vi "BIMS for Export Control.vi"() -> ()   [LabVIEW 2015]
doc: "This program is currently beta software. It is designed to address the data requirements defined primarily by the DHB Ballistic Test Report.\n\nThe general operation of this program is based on the Ballistics Version 2005 application developed internally by DuPont as a research tool for the Spruance Plant Ballistics Lab in Richmond, VA.\n\nPlease note that the original trigger control logic was modified and no longer depends on a safety interlock system to enable operation of a ballistic test.\n\nDuPont makes no warranties and assumes no liabilities in connection with any use of this program."
uses:
  <vilib>/addons/database/NI_Database_API.lvlib
  <vilib>/addons/database/Connection.llb/Conn Execute.vi
  <vilib>/addons/database/Recordset.llb/Rec Destroy - Connection.vi
  <vilib>/Utility/config.llb/NI_LVConfig.lvlib
  <vilib>/Utility/config.llb/Write Key (I32).vi
  Shot Record.ctl
  BIMS_Collector Globals.vi
  Collector State.ctl
  DataSource.ctl
  <vilib>/registry/registry.llb/Registry RtKey.ctl
  <vilib>/Utility/config.llb/Write Key (String).vi
  <vilib>/addons/database/Connection.llb/DB Tools Open Connec (Path).vi
panel:
  out "Loading":u16(ring)
  in  "runtimeMenusVisible":bool=TRUE
  in  "diagPageVisible":bool
  in  "RESET All":bool
  out "ConfigName":string
  out "TimeNow":string
  in  "EXIT":bool
  in  "mainTabCntrl":enum32{"Setup", "Measure", "History", "System"}(tab)=enum."System"
  in  "SampleEntryTabCntrl":enum32{"Environment", "Sample"}(tab)
  in  "ThreatDetails":u16(ring) caption="Detail" items=["2gr 223 cal.   FSP", "4gr 223 cal.   FSP", "16gr 223 cal.", "64gr .357 cal."]
  in  "ThreatGroups":u16(ring) caption="Group" items=["", "RCC", "FSP", "44 Magnum", "40 S&W", "9mm Luger", "357 Magnum", "357 Sig", "5.56 NATO / 223", "7.62 Win"]
  in  "PowderTypes":u16(ring) caption="Type" items=["", "ACCURATE, NO.2", "ACCURATE, NO.9", "Alliant Herc. Bullseye", "Alliant 2400", "Hercules", "Hi-Skor 700x", "Hi-Skor 800x", "IMR-4198", "IMR-4756", "IMR-4895", "Power Pistol", "Winchester Ball", "WINCHESTER-231", "WINCHESTER-296", "OTHER"]
  in  "Ballisticians":u16(ring) caption="Ballistician" items=["", "Luke Jeter", "Pat Fitzgerald", "James Singletary", "Aldo Tavarez"]
  in  "Recorders":u16(ring) caption="Recorder"
  in  "Shooters":u16(ring) caption="Shooter"
  in  "Methods":u16(ring) caption="Method" items=["", "V50", "NIJ", "V0", "Custom"]
  in  "RoomT":sgl caption="Temperature (° F)" format="%.1f"
  in  "RoomHum":sgl caption="Humidity (%)" min=0 max=100 format="%.1f"
  in  "SampleBackings":u16(ring)=3 caption="Type" items=["", "Clay", "Aluminum", "Air"]
  in  "clayCalArray":i16[](array[numeric])=[0, 0, 0, 0, 0] caption="Calibration (mm)" min=0 max=99 format="%02.0f"
  out "clayAverage":sgl caption="Clay Average (mm)" format="%#.1f"
  in  "clayTemp":sgl caption="Clay Temp (° F)" format="%.1f"
  out "threatDetails":T1 caption="Description"
  in  "SampleClamping":u16(ring) caption="Clamping" items=["", "None", "12 x 12", "12 x 15", "15 x 15 Flat", "15 x 15 Teeth", "16 x 16 Flat", "16 x 16 Teeth", "18 x 18", "20 x 20", "Hydro Pneumatic"]
  in  "Sample SubTabCntrl":T2(tab)
  in  "SampleID":string caption="Sample ID"
  in  "SampleDimensions":u16(ring) caption="Dimensions" items=["", "15 x 15", "12 x 12", "10.25 x 11.75", "15 x 16", "26 x 26", "8.5 x 11", "12 x 15", "16 x 16", "18 x 18", "20 x 16", "15 x 18", "24 x 24", "13 x 13", "7.5 x 7.5", "VEST PANEL", "CHEST PLATE", "HELMET", "NOT APPLICABLE"]
  in  "ModelMfrs":u16(ring) caption="Manufacturer" items=["DuPont Experimental", "Clark Schwebel", "Industriales Textiles", "Maydown", "Second Chance Body Armor", "Point Blank-Marine Interceptor", "Safari Land", "American Body Armor", "Europe", "Force One", "Textile Filter", "Hexcel Schwebel", "BGF", "M.C. GILL", "COLUMBIA", "Britax HEATH TECN", "ARLON", "TEX TECH INC.", "TELAIR", "CADDIN BODY ARMOR", "GEPCO", "3 TEX", "PACA BODY ARMOR", "VON ROL ISOLA", "SIOUX MANUFACTURING", "APEJ-TAIWAN", "FLOPPY BODY ARMOR", "UNICOR", "n/a", "Point Blank", "Diamond Back", "Other"]
  in  "SampleTypes":u16(ring) caption="Sample Type" items=["", "Fabric", "Hard", "Helmet", "Vest", "Paper"]
  in  "Submitters":u16(ring) caption="Submitter" items=["", "Aldo Tavarez", "James Singletary", "Jeff Hanks", "Karl Chang", "Minshon Chiou", "Other", "Navin Tejani", "Pat Fitzgerald", "Ron Egres", "Bryce VanArsdalen", "Kevin Mulcahy"]
  in  "ProjectID":string caption="Project ID"
  in  "BackLayers":i32 caption="# of Layers" min=0 max=99 step=5
  in  "FrontLayers":i32 caption="# of Layers" min=0 max=99 step=5
  in  "BackLayer":u16(ring) caption="Back Layer" items=["", "n/a", "CORDURA 500d"]
  in  "FrontLayer":u16(ring) caption="Front Layer" items=["", "n/a", "CORDURA 1000d"]
  out "totalNumLayers":i32 caption="Total # of Layers" min=0 max=100 step=5
  out "totalBAW":sgl caption="Total BAW (psf)" format="%.2f"
  in  "LayerTabControl":enum32{"1", "2", "3", "4", "5", "6"}(tab) caption="Inner Layers"
  out "fab1_totalWt":sgl caption="Fab1 Wt" min=0 max=99 step=5 format="%.2f"
  out "SampleAttribs_1":T3 caption="fabricAttribs_1"
  in  "Layer_1":T4={"plyNum"=0, "LotNum"="n/a", "RollNum"="n/a"} caption="Fabric #1" {"plyNum" min=0 max=99 step=5}
  in  "SampleStyle_1":u16(ring) items=["", "215490", "215590", "217583", "2182", "2710", "2722", "2754", "275580", "400063", "440094", "440094ML", "FC-TWE-1096-160.0-1072"]
  in  "Mfr_1":u16(ring) caption="vendor" items=["", "Barrday", "DSM", "DuPont AFS", "Dyneema", "Honeywell", "JPS", "TexTech"]
  in  "layerStitch_1":u16(ring) caption="Stitch" items=["", "1-inch quilt", "2-inch quilt", "Corner Bartack", "Corners", "Custom (Panel)", "Custom (Vest)", "Diamond", "Edge", "n/a", "Normal"]
  out "fab2_totalWt":sgl caption="Fab2 Wt" min=0 max=99 step=5 format="%.2f"
  out "SampleAttribs_2":T3 caption="fabricAttribs_2"
  in  "Layer_2":T4={"plyNum"=0, "LotNum"="n/a", "RollNum"="n/a"} caption="Fabric #2" {"plyNum" min=0 max=99 step=5}
  in  "SampleStyle_2":u16(ring)
  in  "Mfr_2":u16(ring) caption="vendor" items=["", "Barrday", "DSM", "DuPont AFS", "Dyneema", "Honeywell", "JPS", "TexTech"]
  in  "layerStitch_2":u16(ring) caption="Stitch" items=["", "1-inch quilt", "2-inch quilt", "Corner Bartack", "Corners", "Custom (Panel)", "Custom (Vest)", "Diamond", "Edge", "n/a", "Normal"]
  out "fab3_totalWt":sgl caption="Fab3 Wt" min=0 max=99 step=5 format="%.2f"
  out "SampleAttribs_3":T3 caption="fabricAttribs_3"
  in  "Layer_3":T4={"plyNum"=0, "LotNum"="n/a", "RollNum"="n/a"} caption="Fabric #3" {"plyNum" min=0 max=99 step=5}
  in  "SampleStyle_3":u16(ring)
  in  "Mfr_3":u16(ring) caption="vendor" items=["", "Barrday", "DSM", "DuPont AFS", "Dyneema", "Honeywell", "JPS", "TexTech"]
  in  "layerStitch_3":u16(ring) caption="Stitch" items=["", "1-inch quilt", "2-inch quilt", "Corner Bartack", "Corners", "Custom (Panel)", "Custom (Vest)", "Diamond", "Edge", "n/a", "Normal"]
  out "fab4_totalWt":sgl caption="Fab4 Wt" min=0 max=99 step=5 format="%.2f"
  out "SampleAttribs_4":T3 caption="fabricAttribs_4"
  in  "Layer_4":T4={"plyNum"=0, "LotNum"="n/a", "RollNum"="n/a"} caption="Fabric #4" {"plyNum" min=0 max=99 step=5}
  in  "SampleStyle_4":u16(ring)
  in  "Mfr_4":u16(ring) caption="vendor" items=["", "Barrday", "DSM", "DuPont AFS", "Dyneema", "Honeywell", "JPS", "TexTech"]
  in  "layerStitch_4":u16(ring) caption="Stitch" items=["", "1-inch quilt", "2-inch quilt", "Corner Bartack", "Corners", "Custom (Panel)", "Custom (Vest)", "Diamond", "Edge", "n/a", "Normal"]
  out "fab5_totalWt":sgl caption="Fab5 Wt" min=0 max=99 step=5 format="%.2f"
  out "SampleAttribs_5":T3 caption="fabricAttribs_5"
  in  "Layer_5":T4={"plyNum"=0, "LotNum"="n/a", "RollNum"="n/a"} caption="Fabric #5" {"plyNum" min=0 max=99 step=5}
  in  "SampleStyle_5":u16(ring)
  in  "Mfr_5":u16(ring) caption="vendor" items=["", "Barrday", "DSM", "DuPont AFS", "Dyneema", "Honeywell", "JPS", "TexTech"]
  in  "layerStitch_5":u16(ring) caption="Stitch" items=["", "1-inch quilt", "2-inch quilt", "Corner Bartack", "Corners", "Custom (Panel)", "Custom (Vest)", "Diamond", "Edge", "n/a", "Normal"]
  out "fab6_totalWt":sgl caption="Fab6 Wt" min=0 max=99 step=5 format="%.2f"
  out "SampleAttribs_6":T3 caption="fabricAttribs_6"
  in  "Layer_6":T4={"plyNum"=0, "LotNum"="n/a", "RollNum"="n/a"} caption="Fabric #6" {"plyNum" min=0 max=99 step=5}
  in  "SampleStyle_6":u16(ring)
  in  "Mfr_6":u16(ring) caption="vendor" items=["", "Barrday", "DSM", "DuPont AFS", "Dyneema", "Honeywell", "JPS", "TexTech"]
  in  "layerStitch_6":u16(ring) caption="Stitch" items=["", "1-inch quilt", "2-inch quilt", "Corner Bartack", "Corners", "Custom (Panel)", "Custom (Vest)", "Diamond", "Edge", "n/a", "Normal"]
  in  "SampleCoverings":u16(ring) caption="Sample Covering" items=["None", "RipStop", "Plastic bag", "Other"]
  in  "Assemblers":u16(ring) caption="Technician" items=["", "Not Known", "none", "Ron Egres", "Bryce VanArsdalen", "Mary Revels", "Matthew Street", "Patty Whitlow", "Tom Boyer"]
  in  "Thickness":dbl caption="Thickness (in)" format="%.3f"
  in  "totalSampleWt":sgl caption="Total Weight (lbs)" format="%.3f"
  in  "Comments":string caption="Remarks (optional):"
  in  "TestConditions":u16(ring) caption="Sample Condition" items=["", "Dry", "Wet", "Hot 160 DEG. F", "Cold", "Weapon Lubricant", "Motor Oil", "Conditioned", "Accelerated Aging"]
  in  "shotsTabCntrl":T5(tab)
  in  "Frag Rod":sgl format="%.1f"
  in  "MeasSrc":T6=enum."Screens" caption="Source"
  in  "Drag Corrected":bool=TRUE
  in  "ARM":bool
  in  "readyClock":bool caption="Clock"
  out "Impact/speed":sgl caption="Chronograph 1" min=0 max=10000 step=0.1 format="%.1f"
  out "SHOT STATUS":u16(ring) caption="Penetration" items=["Partial", "Complete"]
  out "residual/speed":sgl caption="Residual" min=0 max=10000 step=0.1 format="%.1f"
  out "SUBMIT DATE/TIME":string
  out "BACKFACE DEPTH":sgl caption="Backface\nDepth" min=0 max=200 step=5
  in  "MeasVelScrnSet1":sgl caption="Set #1" min=0 max=10000 step=0.1 format="%.1f"
  in  "Current/sthotstatus":u16(ring) caption="Penetration" items=["Partial", "Complete"]
  in  "Current/residual/speed":sgl caption="Residual Set" min=0 max=10000 step=0.1 format="%.1f"
  in  "currentDateTime":string caption="Date/Time"
  in  "MeasVelScrnSet2":sgl caption="Set #2" min=0 max=1000000 step=0.1 format="%.1f"
  out "%_Difference":sgl caption="% Vel Diff" format="%.3f"
  in  "backdepth":sgl caption="BF Depth"
  out "Redundant/speed":sgl caption="Chronograph 2" min=0 max=10000 step=0.1 format="%.1f"
  out "Current/avg/speed":sgl caption="Average" min=0 max=1000000 step=0.1 format="%.1f"
  out "Avg/speed":sgl caption="Average" min=0 max=10000 step=0.1 format="%.1f"
  out "SafetyInterlock":cluster{"ARMED":bool}
  out "DC_ factor":sgl=1.0 caption="DC Factor" format="%.4f"
  in  "Barrel Temp":sgl format="%.1f"
  in  "Shot Description":string caption="Description (optional)"
  in  "Powder Loading":sgl caption="Powder Load" min=0 max=100 step=0.1 format="%.3f"
  in  "Shot Angle":u16 max=90 step=1
  out "Projectile Mass":sgl caption="Projectile Mass (grains)" min=0 step=1
  in  "N.I.J":u16(ring) items=["n/a", "PASS", "FAIL"]
  out "Device S/N":string
  in  "addShot":bool caption="RANGE SETUP must be selected before shots can be added."
  in  "loadingUnits":enum32{"grams", "grains"}(radio)
  out "instruct_addShot":string="RANGE SETUP and THREAT must be selected before shots can be added."
  out "Set#1 Separation":sgl=4.0 caption="Outer" format="%.2f"
  out "Set#2 Separation":sgl=4.0 caption="Inner" format="%.2f"
  out "saveReq":string="Number of layers in sample ply specification and number of shots in shots table must be greater than 0 to enable saving."
  in  "VsVr Report":bool caption="Report"
  out "Table of Shots":string[][](table) caption="Shot Table"
  in  "MC Listbox of Shots":i32(listbox)
  in  "saveShots":bool
  in  "clearShots":bool
  out "highPartial":i32 caption="High Partial" min=0 max=10000 step=1
  out "lowComplete":i32 caption="Low Complete" min=0 max=10000 step=1
  out "rangeOfResults":i32 caption="Range of Results" min=0 max=10000 step=1
  out "zmr 2":sgl caption="Low C minus High P" format="%.1f"
  out "computed_V50":sgl caption="V50" format="%.1f"
  out "Pairs":i16 min=0 max=100 step=1
  in  "reportV50":bool caption="Report"
  in  "maxDev":sgl=125.0 caption="Max Deviation" min=0 max=300 step=25
  in  "undoLastShot":bool
  in  "deleteShot":bool
  in  "nextShot":bool
  in  "SHOTS":T7[](array[typedef]) {"Frag Rod" format="%.1f"; "UncorrectedAvgVel_PB" format="%.1f"; "UncorrectedRed_PB" format="%.1f"; "strikeVel_PB" format="%.1f"; "velLoss_PB" format="%.1f"; "avgVel_PB" format="%.1f"; "Redundant_Velocity" format="%.1f"; "Energy Loss (J)" format="%.3e"; "Projectile Mass" min=0 step=1 format="%.4f"; "Corrected residual" format="%.2f"; "Uncorrected Residual" format="%.1f"; "Corrected Impact" format="%.2f"; "Uncorrected Impact" format="%.1f"; "Shot Angle" max=90 step=1; "SHOT STATUS" items=["Partial", "Complete"]; "IMPACT VELOCITY" min=0 max=10000 step=0.1 format="%.1f"; "Barrel Temperature" format="%.1f"; "Powder Loading" format="%.4f"; "RESIDUAL  VELOCITY" min=0 max=10000 step=0.1 format="%.1f"}
  out "velProfile":cluster{dbl, dbl}[](graph) caption="Shot Velocity Measurement Profile"
  out "velCompProf":cluster{"vStrike":dbl, "vA":dbl} caption="Velocity in fps\n(computed)"
  out "velMeasProf":T8 caption="Velocity in fps\n(measured)"
  out "relativeTime":cluster{"ts2":dbl, "ts3":dbl, "ts1":dbl} caption="Relative time\n(microsec)"
  out "displacement":T9={"ds_v2"=6.75, "ds2"=5.0833, "ds_vB"=4.9167, "ds3"=4.75, "ds_vAvg"=6.9167, "ds_v1"=7.0833, "ds1"=8.75, "ds_vA"=8.9167, "ds0"=9.0833} caption="Distance from\ntarget (ft)" {"ds0" format="%_4g"; "ds_vA" format="%_4g"; "ds1" format="%_4g"; "ds_v1" format="%_4g"; "ds_vAvg" format="%_4g"; "ds3" format="%_4g"; "ds_vB" format="%#_4g"; "ds2" format="%#_4g"; "ds_v2" format="%_4g"}
  out "arrIDC":dbl[](array[numeric]) caption="Instantaneous Drag Coefficient"
  in  "rangeSetup":u16(ring)=1 caption="Range Dimensions" items=["Short (small frag)", "Standard (handgun)", "Long (rifle)"]
  out "mid_to_targ_dist":sgl=5.0 caption="Mid To Target (ft)"
  in  "historyTabCntrl":enum32{"Powder Loading", "Panel Search"}(tab)=enum."Panel Search"
  in  "Threat.freeTxt":string caption="Threat"
  in  "Powder.freeTxt":string caption="Powder"
  in  "QueryLoad":bool
  in  "lkupEndDate":timestamp caption="End Date" format="%<%x>T"
  in  "lkupStartDate":timestamp caption="Begin Date" format="%<%x>T"
  out "Vel.vs.Loading":cluster{dbl[], dbl[]}(graph)
  out "v50_table":string[][](table)
  in  "maxRecs":u16=1001 caption="Max # of SHOT Records" min=1 max=10000 step=100
  out "ActualNumRecs":i32=1001 caption="Actual # Returned"
  in  "ThreatSize_0":u16(ring) caption="Threat Size" items=["", "2", "4", "16", "17", "44", "55", "62", "64", "85", "123", "124", "125", "148", "158", "166", "180", "207", "240"]
  in  "panelSearch":bool
  in  "Mfr_0":u16(ring) caption="Manufacturer" items=["", "Barrday", "DSM", "DuPont AFS", "Dyneema", "Honeywell", "JPS", "TexTech"]
  in  "SampleStyle_0":u16(ring) caption="Sample Style"
  in  "srchParams":T10={"maxPanels"=1001, "lkupPanelStartDate"=timestamp(0 s since 1904-01-01), "lkupPanelEndDate"=timestamp(3345122114.0909824 s since 1904-01-01)} {"lkupPanelEndDate" format="%<%x>T"; "lkupPanelStartDate" format="%<%x>T"; "maxPanels" min=1 max=10000 step=100}
  out "actualNumPanels":i32 caption="Actual # Returned"
  out "pastPanels":string[][](table)
  in  "Record #":i32=1 min=0 max=16
  in  "reportV50_History":bool
  out "SampleAttribs_0":T11 caption="fabricAttribs_1"
  in  "Requestors_0":u16(ring) caption="Requestor" items=["", "Aldo Tavarez", "Bryce VanArsdalen", "James Singletary", "Jeff Hanks", "Karl Chang", "Kevin Mulcahy", "Minshon Chiou", "Navin Tejani", "Other", "Pat Fitzgerald", "Ron Egres"]
  in  "aboutTabCntrl":T12(tab)
  in  "RefreshMetadata":bool
  out "LastShot":i32 caption="Shot"
  out "LastSample":i32 caption="Sample"
  in  "PublishNewRecords":bool
  in  "Folder":string="esvrs11" caption="Publish Folder"
  in  "clearErrors":bool
  in  "useBMC":bool caption="Use Message Center?"
  in  "Server":string="esvrs11"
  in  "Site":string="ICE1"
  in  "TestStandards":u16(ring)=2 caption="Standard" items=["n/a", "NIJ 0101.04", "MIL-STD-662F"]
  in  "WeaponTypes":u16(ring) caption="Weapon" items=["", "Universal Receiver", "Other"]
  in  "processShots":bool
  out "DIO":u32=21 format="%.0b"
  in  "line direction map":i32=1792 format="%.0b"
  out "Corrected Average":sgl=1527.9313 format="%.2f"
  out "CorrectedVelScrnSet2":sgl=1551.8816 caption="Corrected Redundant" format="%.2f"
  out "conversion factor":sgl=0.3048037 format="%.5f"
  out "#_completes":i32
  out "#_partials":i32
  in  "percent warning":sgl=1.0 format="%.2f"
  in  "SoftwareVersion":dbl caption="Version" format="%.2f"
  out "impact/ID":u32=83886081 format="%.0x"
  out "residual/ID":u32=83951617 format="%.0x"
  out "Red/ID":u32=84017153 format="%.0x"
  out "correction coefficient":sgl format="%.8f"
  out "Corrected Residual":sgl=751.9905 format="%.2f"
  out "CorrectedVelScrnSet1":sgl=1503.981 format="%.2f"
  out "Barrel to Screen":sgl=7.8333 format="%.2f"
  in  "Set#1_to_Target":sgl=7.083333 format="%.2f"
  out "Residual/Separation":sgl=4.0 format="%.2f"
  in  "Residual/Target Dist":sgl=7.083333 format="%.2f"
  out "Z.M.R.":sgl min=0 step=0.1 format="%.1f"
  in  "old threat":u16
  out "Complete":sgl[](array[numeric]) format="%.2f"
  out "factor array":sgl[](array[numeric]) format="%.4f"
  out "Partial":sgl[](array[numeric]) format="%.2f"
  in  "DAQ Card":i16=1
  in  "Impact Timer":i16 min=0 max=3 step=1
  in  "Redundant Timer":i16=1 min=0 max=3 step=1
  in  "Residual  Timer":i16=2 min=0 max=3 step=1
  out "Impact factor":sgl=1.0 caption="Impact" min=0 max=1 format="%.5f"
  out "Residual factor":sgl=1.0 caption="Residual" min=0 max=1 format="%.5f"
  in  "Areal Density":dbl format="%.2f"
  in  "Areal density text":string
  in  "Fabric Description":string caption="Fabric Desc"
  in  "clayCalib":string="##-##-##-##-##" caption="Calibration"
  in  "lookupRec":bool caption="lookup"
  out "STOP (Shots MC LB)":bool=TRUE
  out "configPath":path=path "P:/Private/My Projects/AFS/BIMS/2008/BIMS_Collector.ini" caption="Configuration Path (INI)"
  in  "minV50":i32=1500 caption="Minimum V50"
  in  "Type of work":string="QC"
  in  "Threat":u16(ring) caption="Threat (long description)"
  out "massUnits":string="GRAMS" caption="Weight Units"
  out "lengthUnits":string="FOOT" caption="Distance Units"
  in  "SampleDescrip":u16(ring) caption="Misc. Sample Description (legacy)"
  in  "serialNum":string caption="Serial #"
  in  "Models":u16(ring) caption="Model #" items=["n/a"]
  in  "InterlockExists":bool=TRUE caption="Safety Interlock Hardware Exist?"
  in  "ScreenSetAvgg":bool caption="Average Screen Sets?"
  in  "Sort by AVG":bool=TRUE caption="Sort shots by average velocity"
  in  "useBallisitican":bool=TRUE caption="Use Ballistician field in Setup?"
  in  "useRecorder":bool caption="Use Recorder field in Setup?"
  in  "useShooter":bool caption="Use Shooter field in Setup?"
  out "SMErr":errorcluster
  out "U/I EvErr":errorcluster
  out "booleanDump":bool
  out "GrainSize":u16 caption="Grain"
  in  "LayerStitchTypes":u16(ring) caption="Stitch" items=["", "Custom (Vest)", "Corners", "1-inch quilt", "2-inch quilt", "Normal", "Custom (Panel)", "Corner Bartack", "Diamond", "Edge", "n/a"]
  # "Effectively restarts the application from scratch, as if the user pressed the EXIT button and then restarted the application."
  # "Configured for"
  # "Threat"
  # "*"
  # "*"
  # "Test"
  # "Powder"
  # "*"
  # "Personnel"
  # "Room"
  # "*"
  # "Backing"
  # "*"
  # "*"
  # "*"
  # "Body Side"
  # "Strike Face"
  # "Layer"
  # "Mfr"
  # "Style"
  # "# of Plies"
  # "Lot"
  # "Roll"
  # "Stitch"
  # "Internal ID"
  # "Fiber"
  # "Denier"
  # "Construction"
  # "Weave"
  # "Finish"
  # "Basis weight (oz/yd²)"
  # "Yarn Merge"
  # "Total Weight"
  # "*"
  # "*"
  # "*"
  # "1"
  # "2"
  # "3"
  # "4"
  # "5"
  # "6"
  # "Required"
  # "*"
  # "Timing System"
  # "Shot Parameters"
  # "cm"
  # "deg"
  # "degF"
  # "Velocity Measurements"
  # "Observations"
  # "Screens\nSeparation"
  # "Ft"
  # "Table Functions"
  # "Summary"
  # "Reports"
  # "Test Record"
  # "Edit Shot Records"
  # "Corrected"
  # "Shot #"
  # "t0"
  # "0"
  # "S Strike"
  # "0"
  # "Internal ID#"
  # "Fiber"
  # "Denier"
  # "Pick"
  # "Weave"
  # "Finish"
  # "oz/yd²"
  # "Asset"
  # "DuPont Ballistics Information Management System\n\nBIMS\nFor Export Control\n\n\nBallistic Performance\nData Collector\n\nJune 2010"
  # "DuET Measurement System Technologies\nDUCOM 8 695-2330 for technical support\n\nCopyright © 2010 DuPont Company"
  # "Last Assigned\nRecord Numbers"
  # "Deployment Configuration"
  # "Data items support Point Blank requirements:"
  # "Correction Factors"
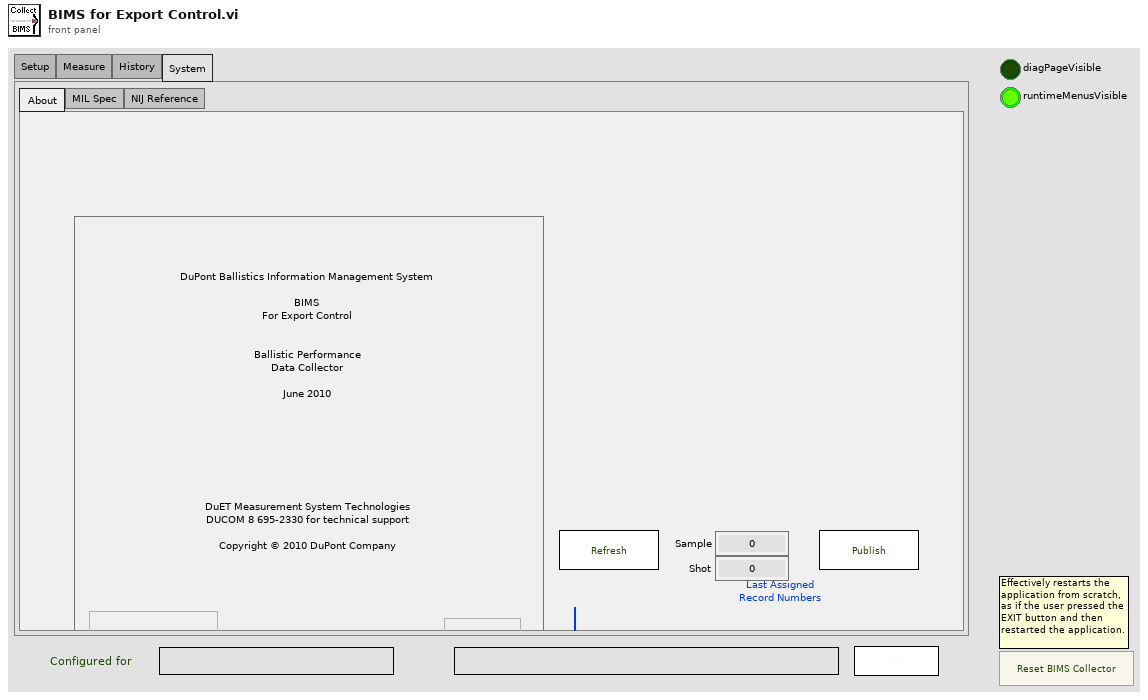
[diagram p1: front panel]
types:
  T1 = cluster{"barrelLength":string, "dragCorrection":string, "detailDescription":string, "barrelCaliber":string, "grainSize":string, "Make":string, "Model":string}
  T2 = enum32{"General Specification", "Ply Specification", "Preparation"}
  T3 = cluster{"Fabric.fiber":string, "Fabric.denier":string, "pick":string, "weave":string, "finish":string, "ozPerYd2":string, "fabricID_DHB":string, "yarnMerge":string}
  T4 = cluster{"plyNum":i32, "LotNum":string, "RollNum":string}
  T5 = enum32{"Ready-Aim-Fire", "Shots Table", "Edit", "Instantaneous DC"}
  T6 = typedef "DataSource.ctl" = enum16{"Simulated", "Radar", "Screens"}
  T7 = typedef "Shot Record.ctl" = cluster{"Uncorrected Impact":sgl, "Uncorrected Residual":sgl, "avgVel_PB":sgl, "IMPACT VELOCITY":sgl, "RESIDUAL  VELOCITY ":sgl, "Shot Description":string, "Powder Loading ":sgl, "Barrel Temperature":sgl, "TIME / DATE":string, "shot order":i32, "SHOT STATUS":u16, "Shot Angle":u16, "Corrected Impact":sgl, "Corrected residual":sgl, "Projectile Mass":sgl, "usedv50":bool, "Energy Loss (J)":sgl, "BackFace\nDepth":sgl, "BackFace\nDiameter":sgl, "Redundant_Velocity":sgl, "velLoss_PB":sgl, "strikeVel_PB":sgl, "UncorrectedRed_PB":sgl, "CorrectedRed_PB":sgl, "UncorrectedAvgVel_PB":sgl, "V50userExcl":bool, "Frag Rod":sgl}
  T8 = cluster{"v2":dbl, "vB":dbl, "vOuter":dbl, "v1":dbl, "vA":dbl, "vInner":dbl}
  T9 = cluster{"ds_v2":dbl, "ds2":dbl, "ds_vB":dbl, "ds3":dbl, "ds_vAvg":dbl, "ds_v1":dbl, "ds1":dbl, "ds_vA":dbl, "ds0":dbl}
  T10 = cluster{"maxPanels":u16, "lkupPanelStartDate":timestamp, "lkupPanelEndDate":timestamp}
  T11 = cluster{"Fabric.fiber":string, "Fabric.denier":string, "pick":string, "weave":string, "finish":string, "ozPerYd2":string, "fabricID_DHB":string, "asset":string}
  T12 = enum32{"About ", "MIL Spec", "NIJ Reference", "Internal Use"}
  T13 = typedef "Collector State.ctl" = enum16{"POLL", "INITIALIZE", "V50 Report or GET Record", "VsVr Report", "SAVE SHOTS", "ADD SHOT", "CLEAR SHOTS", "NEXT SHOT", "DELETE SHOT", "READY CLOCK", "PROC SHOTS", "CHECK DAQ"}
  T14 = enum8{"Enabled", "Disabled", "Disabled and Grayed Out"}
  T15 = enum32{"Page Enabled", "Page Disabled", "Page Disabled & Grayed"}
  T16 = typedef "Registry RtKey.ctl" = enum32{"HKEY_CLASSES_ROOT", "HKEY_CURRENT_USER", "HKEY_LOCAL_MACHINE", "HKEY_USERS", "HKEY_PERFORMANCE_DATA", "HKEY_CURRENT_CONFIG", "HKEY_DYN_DATA"}
  T17 = cluster{"[0]":string, "[1]":string, "[2]":string, "[3]":string, "[4]":string, "[5]":string, "[6]":string, "[7]":string, "[8]":string, "[9]":string}[]
  T18 = cluster{"[0]":string, "[1]":string, "[2]":string, "[3]":string, "[4]":string, "[5]":string, "[6]":string, "[7]":string, "[8]":string}[]
  T19 = typedef "Collector State.ctl" = enum16{"POLL", "INITIALIZE", "V50 Report or GET Record", "VsVr Report", "SAVE SHOTS", "ADD SHOT", "CLEAR SHOTS", "NEXT SHOT", "DELETE SHOT", "PROCESS SHOTS", "READY CLOCK", "CHECK DAQ"}
  T20 = cluster{"Fabric.fiber":string, "Fabric.denier":string, "pick":string, "weave":string, "finish":string, "ozPerYd2":string, "fabricID_DHB":string, "yarnMerge":string}[]
  T21 = cluster{"SampleTypes":refnum<vi>, "SampleDescrip":refnum<vi>}
  T22 = cluster{"max dev":sgl, "residual separation":sgl, "Set#1 Separation":sgl, "Set#2 Separation ":sgl, "impact target dist":sgl, "resid target dist":sgl, "barrel screen dist":sgl, "midpt_to_target_dist":sgl}
  T23 = cluster{"fiber":string, "denier":string, "pick":string, "weave":string, "finish":string, "ozPerYd2":string, "internal_ID":string, "asset":string}[]
  T24 = cluster{"numOfPlies":i32, "LotNum":string, "RollNum":string}[]
  T25 = cluster{string, string, string, string, string, string, string, string, "clayCalib":string, string}
  T26 = cluster{string, string, string, string, string, string, string}
  T27 = cluster{"SampleID":string, "element":string, "Type of work":string, "serialNum":string, "element":string, string, string, string, "element":string, string}
  T28 = cluster{"SampleID":string, "element":string, string, string, string, "element":string}
  T29 = cluster{"[0]":string, "[1]":string, "[2]":string, "[3]":string, "[4]":string, "[5]":string, "[6]":string, "[7]":string, "[8]":string, "[9]":string}
  T30 = cluster{"[0]":string, "[1]":string, "[2]":string, "[3]":string, "[4]":string, "[5]":string, "[6]":string, "[7]":string, "[8]":string}
  T31 = cluster{"element":string, "element":string, "grainSize":string, "element":string, "barrelLength":string, string, "element":string, "element":string, "element":string}
  T32 = cluster{"element":string, "grainSize":string, "element":string, "barrelLength":string, string, "element":string}
  T33 = typedef "NI_Database_API.lvlib/Conn ObjectReference.ctl" = refnum<k1>
  T34 = typedef "NI_Database_API.lvlib/Rec ObjectReference.ctl" = refnum<k1>
  T35 = typedef "NI_LVConfig.lvlib/Config Data RefNum.ctl" = refnum<k1>
  T36 = cluster{"task ID out":u32, "task ID out":u32, "task ID out":u32}
  T37 = enum32{"invalid app kind", "Development System", "Run Time System", "Student Edition", "Embedded LabVIEW", "Evaluation", "Custom"}
  T38 = typedef "LVRowAndColumnTypeDef.ctl" = cluster{"Row":i32, "Column":i32}
  T39 = cluster{"barrelLength":string, "dragCoefficient":string, "detailDescription":string, "barrelCaliber":string, "grainSize":string, "Make":string, "Model":string}
  T40 = cluster{"fiber":string, "denier":string, "construction":string, "weave":string, "finish":string, "ozPerYd2":string, "fabricStyle_DHB":string, "yarnMerge":string}
  T41 = cluster{"plyNum":i32, "LotNum":string, "RollNum":string}[]
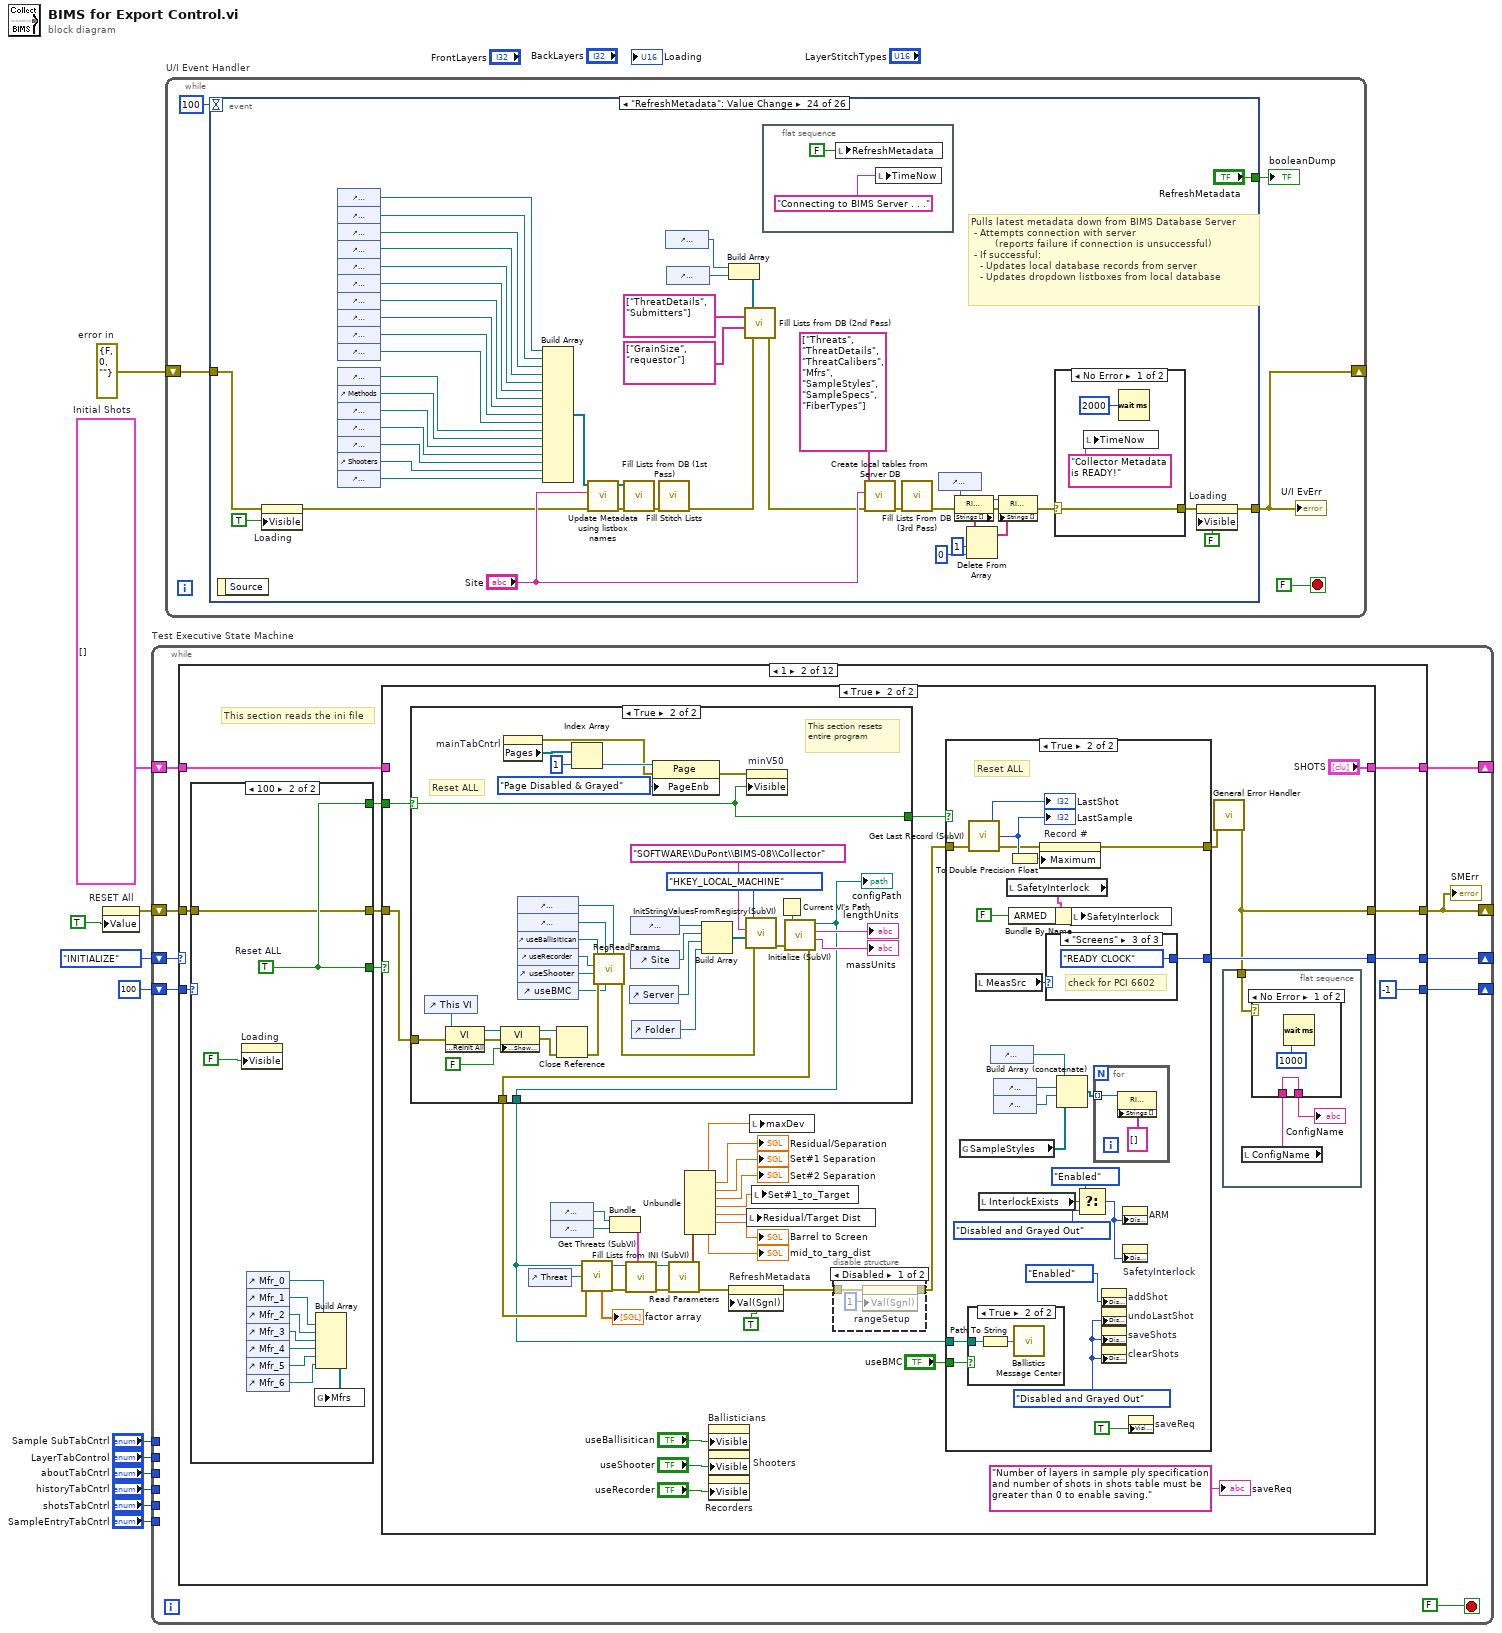
[diagram p0: block diagram]
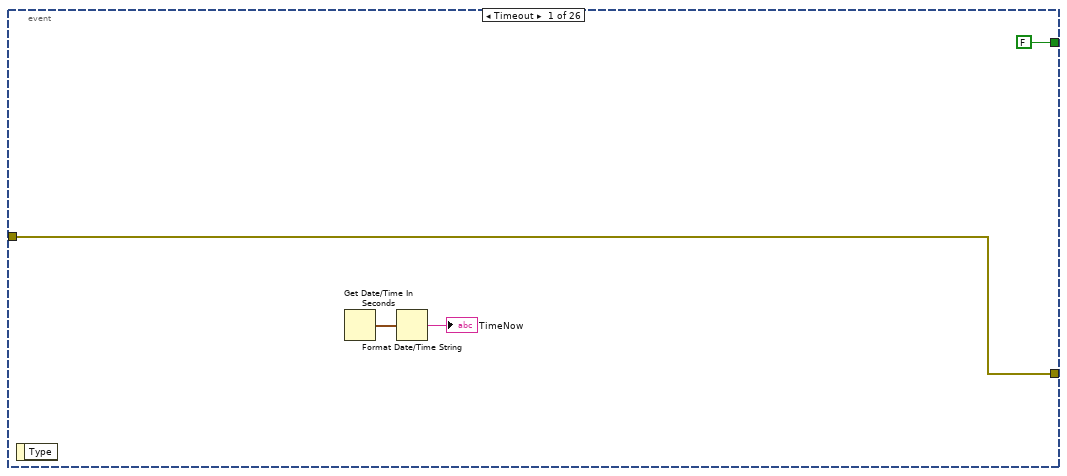
[diagram p2: hidden frame]
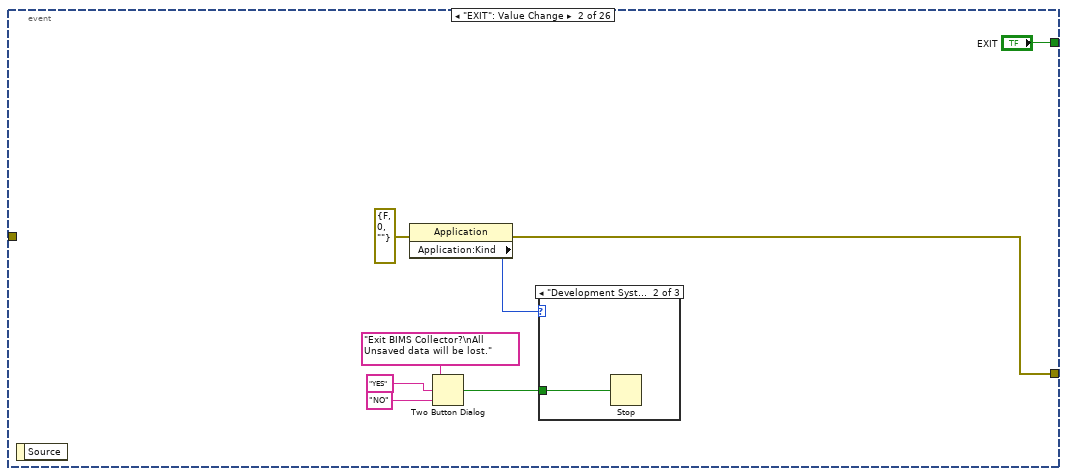
[diagram p3: hidden frame]
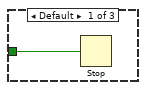
[diagram p4: hidden frame]
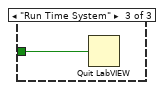
[diagram p5: hidden frame]
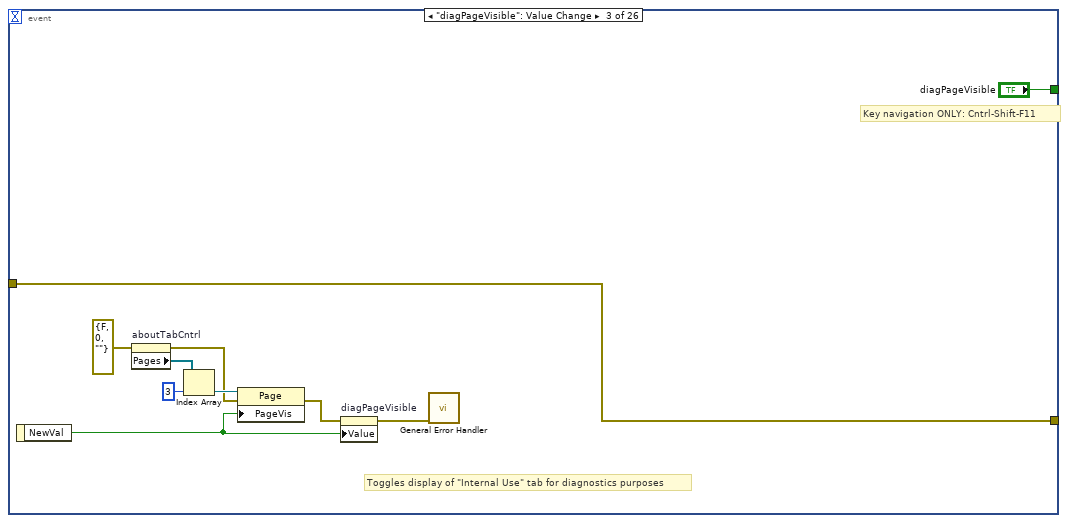
[diagram p6: hidden frame]
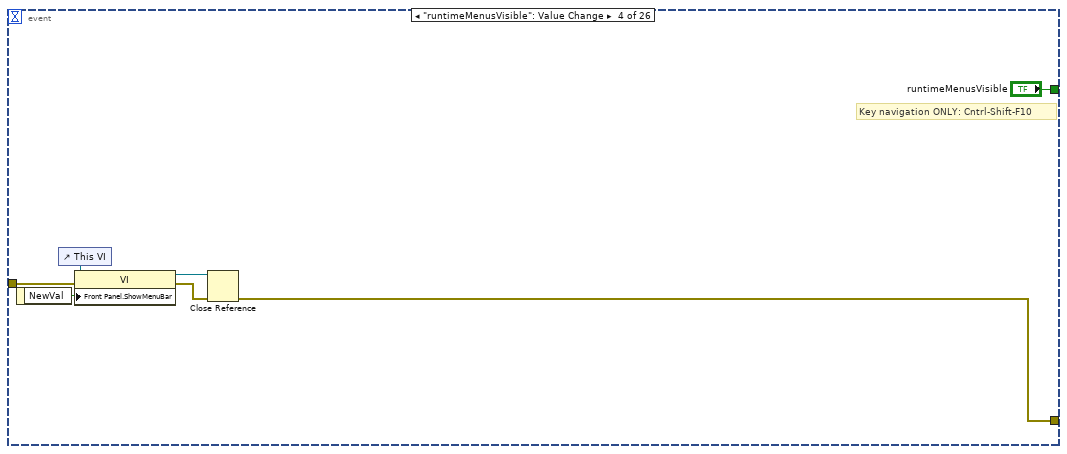
[diagram p7: hidden frame]
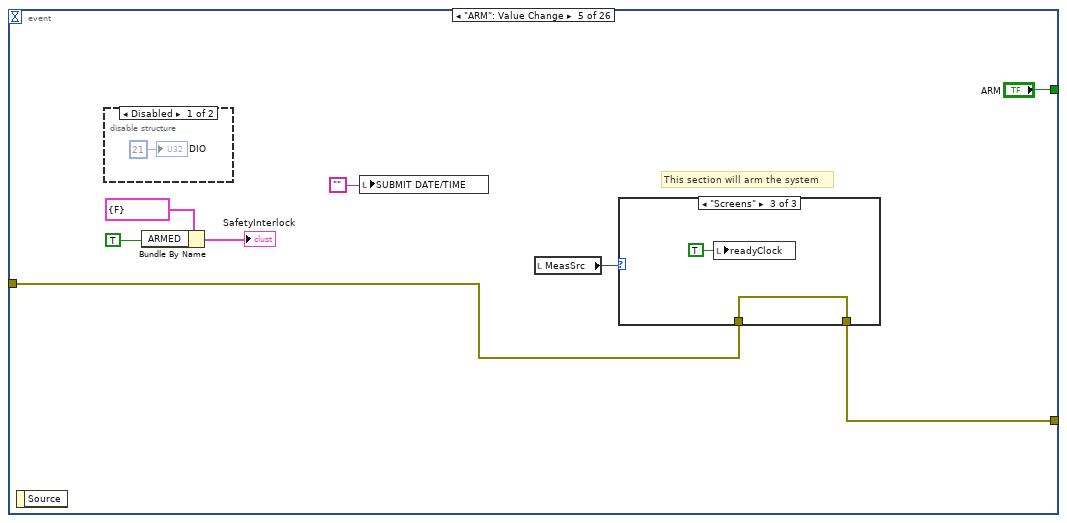
[diagram p8: hidden frame]
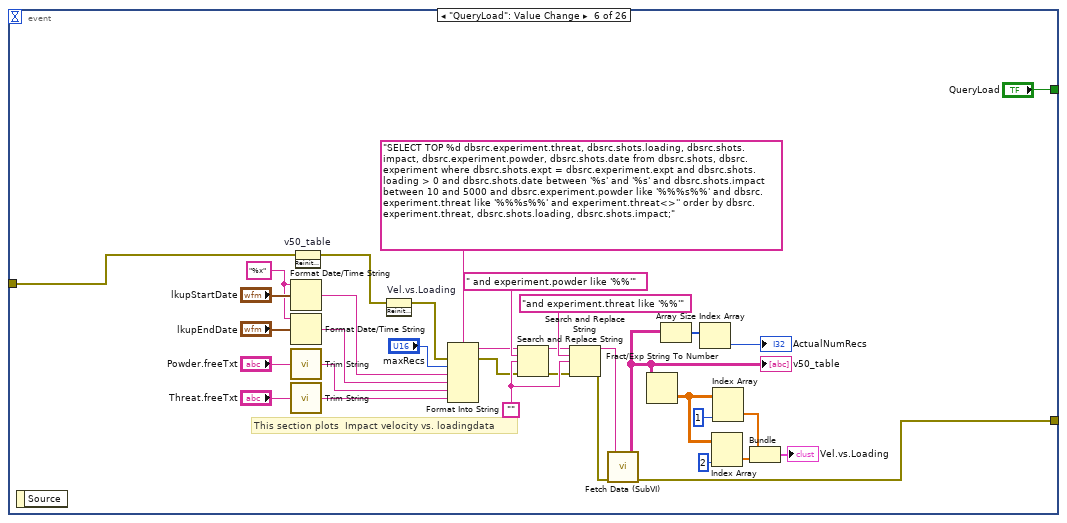
[diagram p12: hidden frame]
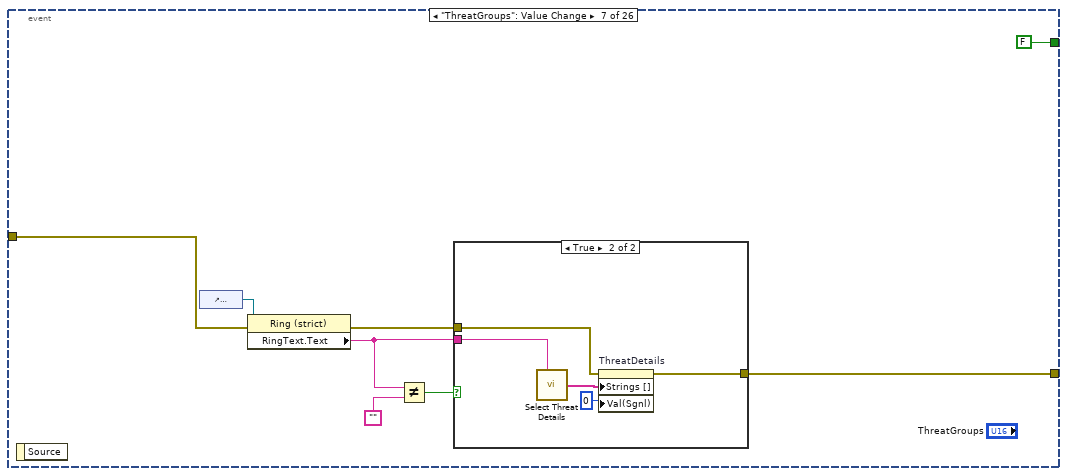
[diagram p13: hidden frame]
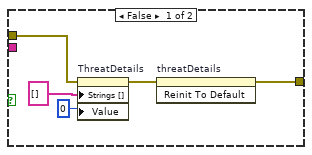
[diagram p14: hidden frame]
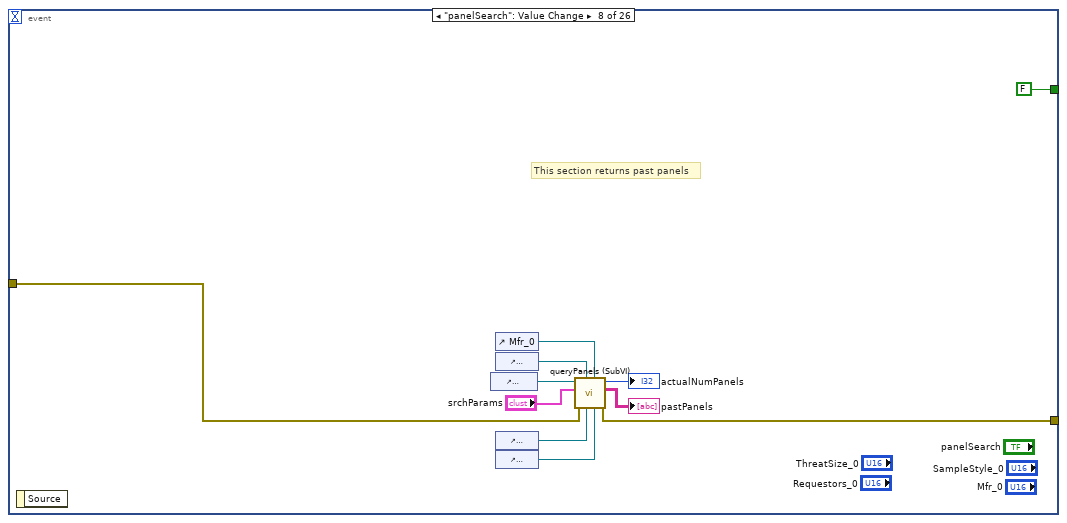
[diagram p15: hidden frame]
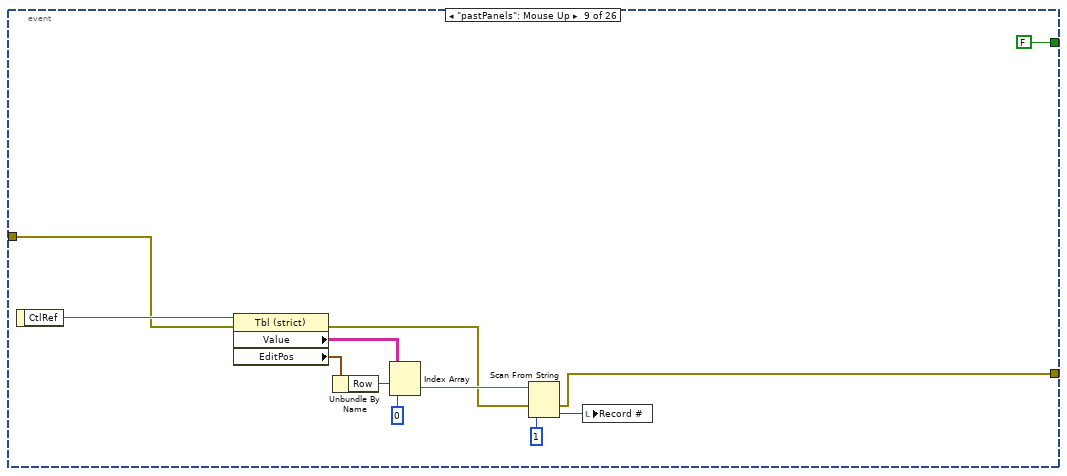
[diagram p16: hidden frame]
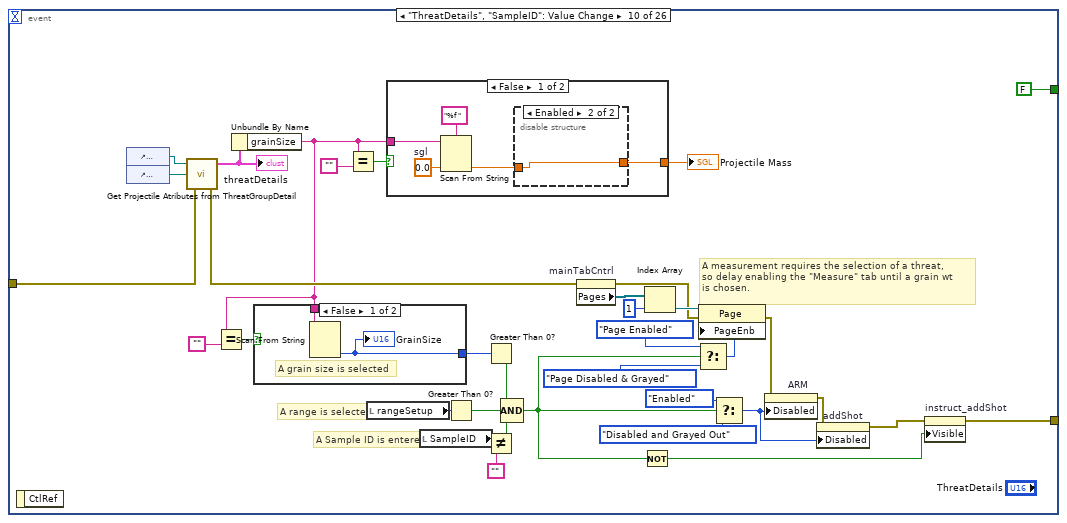
[diagram p17: hidden frame]
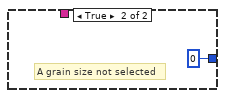
[diagram p18: hidden frame]
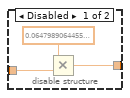
[diagram p19: hidden frame]
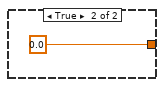
[diagram p20: hidden frame]
diagram:
  w7 = errorcluster {"status"=FALSE, "code"=0, "source"=""}  # error in
  w8 = T7[] []  # Initial Shots
  n1 = property on="RESET All" class="Bool (strict)"("Value"=TRUE ("RESET")) -> (error out=w10:errorcluster)  [unwired: 2 in, 1 out]
  n2 = while "Test Executive State Machine" {
    shift-left: 100 -> [w18]
    shift-right: [w19] -> _
    shift-left: Collector_State."INITIALIZE" ("progState") -> [w15]
    shift-right: [w20] -> _
    shift-right: [w16] -> _
    shift-left: w8 -> [w17]
    shift-right: [w13] -> _
    shift-left: w10 -> [w14]
    tunnel: "LayerTabControl" -> [_]
    tunnel: "aboutTabCntrl" -> [_]
    tunnel: "historyTabCntrl" -> [_]
    tunnel: "shotsTabCntrl" -> [_]
    tunnel: "SampleEntryTabCntrl" -> [_]
    tunnel: "Sample SubTabCntrl" -> [_]
    stop <- FALSE stop-if-true
    n3 = case shown="1" w15 {
      tunnel: [w37 w137 Collector_State."POLL" ("progState") Collector_State."POLL" ("progState") w1073 Collector_State."PROCESS SHOTS" ("progState") Collector_State."POLL" ("progState") Collector_State."PROCESS SHOTS" ("progState") Collector_State."PROCESS SHOTS" ("progState") Collector_State."POLL" ("progState") Collector_State."POLL" ("progState") w1736] -> w20
      tunnel: [-1 -1 ("index of element") -1 ("index of element") -1 ("index of element") w1072 -1 ("index of element") -1 -1 ("index of element") -1 ("index of element") -1 -1 ("index of element") w1735] -> w19
      tunnel: w18 -> [_ w138 _ _ _ _ _ _ _ _ _ _]
      tunnel: w17 -> [w34 w136 w293 w820 w1066 w1329 w1374 w1397 w1403 w1456 w1508 w1739]
      tunnel: [w34 w135 w293 w820 w1065 w1324 w1378 w1396 w1402 w1456 w1512 w1739] -> w16
      tunnel: w14 -> [_ w131 w290 w818 w1068 w1323 w1370 w1386 w1398 w1452 w1507 w1730]
      tunnel: [w28 w132 w289 w817 w1067 w1321 w1370 w1384 w1399 w1451 w1506 w1731] -> w13
      frame 0, Default {
        w53 = Collector_State."POLL"  # progStateType
        w43 = TRUE  # element
        w46 = 4  # SAVE
        # "This section checks for any buttons, maintains routine check of the paramters"
        n4 = case shown="\"System\"" "mainTabCntrl" {
          tunnel: w34 -> [_ w98 _ _]
          frame "Setup", Default {
            n5 = control-ref of="layerStitch_1"() -> (w66:refnum<vi>)
            n6 = control-ref of="layerStitch_2"() -> (w65:refnum<vi>)
            n7 = control-ref of="layerStitch_3"() -> (w64:refnum<vi>)
            n8 = control-ref of="layerStitch_4"() -> (w63:refnum<vi>)
            n9 = control-ref of="layerStitch_5"() -> (w62:refnum<vi>)
            n10 = control-ref of="layerStitch_6"() -> (w61:refnum<vi>)
            n11 = control-ref of="SampleStyle_0"() -> (w59:refnum<vi>)
            n12 = control-ref of="SampleStyle_1"() -> (w80:refnum<vi>)
            n13 = control-ref of="SampleStyle_2"() -> (w81:refnum<vi>)
            n14 = control-ref of="SampleStyle_3"() -> (w82:refnum<vi>)
            n15 = control-ref of="SampleStyle_4"() -> (w83:refnum<vi>)
            n16 = control-ref of="SampleStyle_5"() -> (w84:refnum<vi>)
            n17 = control-ref of="SampleStyle_6"() -> (w85:refnum<vi>)
            n18 = Build Array(w59, w80, w81, w82, w83, w84, w85) -> (w78:refnum<vi>[])
            n19 = global write "BIMS_Collector Globals.vi" "SampleStyles"(w78) -> ()
            n20 = Build Array(w66, w65, w64, w63, w62, w61) -> (w67:refnum<vi>[])
            n21 = global write "BIMS_Collector Globals.vi" "LayerStitchTypeRefs"(w67) -> ()
            n22 = local read "SampleAttribs_1"() -> (w72:T3)
            n23 = local read "SampleAttribs_2"() -> (w74:T3)
            n24 = local read "SampleAttribs_3"() -> (w75:T3)
            n25 = local read "SampleAttribs_4"() -> (w76:T3)
            n26 = local read "SampleAttribs_5"() -> (w77:T3)
            n27 = local read "SampleAttribs_6"() -> (w73:T3)
            n28 = Build Array(w72, w74, w75, w76, w77, w73) -> (w71:T20)
            n29 = global write "BIMS_Collector Globals.vi" "SampleAttribs"(w71) -> ()
            n30 = local read "Fabric Description"() -> (w70:string)
            n31 = control-ref of="Mfr_0"() -> (w60:refnum<vi>)
            n32 = control-ref of="Mfr_1"() -> (w91:refnum<vi>)
            n33 = control-ref of="Mfr_2"() -> (w90:refnum<vi>)
            n34 = control-ref of="Mfr_3"() -> (w89:refnum<vi>)
            n35 = control-ref of="Mfr_4"() -> (w88:refnum<vi>)
            n36 = control-ref of="Mfr_5"() -> (w87:refnum<vi>)
            n37 = control-ref of="Mfr_6"() -> (w86:refnum<vi>)
            n38 = String Subset(string=w70, length (rest)=75 ("length (rest)")) -> (substring=w69:string)  [unwired: 1 out]
            n39 = Build Array(w60, w91, w90, w89, w88, w87, w86) -> (w79:refnum<vi>[])
            n40 = local write "Fabric Description"(w69) -> ()
            n41 = global write "BIMS_Collector Globals.vi" "Mfrs"(w79) -> ()
          }
          frame "Measure" {
            # "Disable and gray out the \"Save\" button\nIF the shot table has no shots, \nOR if there are no plies; otherwise, enable it."
            # "Disable and gray out the \"Clear Shots\" button\nIF the shot table has no shots; otherwise, enable it."
            n42 = local read "totalNumLayers"() -> (w107:i32)
            n43 = Array Size(array=w98) -> (size(s)=w108:i32)
            n44 = Equal To 0?(x=w107) -> (x = 0?=w106:bool)
            n45 = Equal To 0?(x=w108) -> (x = 0?=w104:bool)
            n46 = Or(x=w104, y=w106) -> (x .or. y?=w97:bool)
            n47 = property on="saveReq" class="Str"("Visible"=w97) -> ()  [unwired: 2 in, 2 out]
            n48 = Select(t=T14."Disabled and Grayed Out" ("Disabled"), s=w104, f=T14."Enabled" ("Disabled")) -> (s? t:f=w105:T14)
            n49 = Select(t=T14."Disabled and Grayed Out" ("Disabled"), s=w97, f=T14."Enabled" ("Disabled")) -> (s? t:f=w92:T14)
            n50 = property on="reportV50" class="Bool"("Disabled"=w92) -> ()  [unwired: 2 in, 2 out]
            n51 = property on="saveShots" class="Bool"("Disabled"=w92) -> ()  [unwired: 2 in, 2 out]
            n52 = property on="clearShots" class="Bool"("Disabled"=w105) -> ()  [unwired: 2 in, 2 out]
            n53 = local read "Shot Description"() -> (w101:string)
            n54 = String Subset(string=w101, length (rest)=30 ("length (rest)")) -> (substring=w99:string)  [unwired: 1 out]
            n55 = local write "Shot Description"(w99) -> ()
            "SHOT STATUS" <- "Current/sthotstatus"
            "BACKFACE DEPTH" <- "backdepth"
          }
          frame "History" {
          }
          frame "System" {
          }
        }
        n56 = Get Date/Time String(want seconds? (F)=TRUE) -> (date string=w26:string, time string=w27:string)  [unwired: 2 in]
        n57 = call <vilib>:"Space Constant.vi"() -> ("String"=w24:string)
        n58 = Concatenate Strings(w26, w24, w27) -> (w25:string)
        n59 = local write "currentDateTime"(w25) -> ()
        n60 = Or(x="undoLastShot", y="deleteShot") -> (x .or. y?=w41:bool)
        n61 = Or(x="reportV50", y="reportV50_History") -> (x .or. y?=w49:bool)
        n62 = flat-sequence {
          tunnel: [w58] -> w22
          frame #0 {
            n63 = Wait (ms)(milliseconds to wait=u32 200 ("millisecond timer value")) -> ()  [unwired: 1 out]
          }
          frame #1 {
            n64 = local read "SMErr"() -> (w58:errorcluster)
          }
        }
        n65 = Build Array("RESET All", w49, "VsVr Report", "saveShots", "addShot", "clearShots", "nextShot", w41, "processShots", "readyClock") -> (w44:bool[])
        n66 = Search 1D Array(1D array=w44, element=w43) -> (index of element=w55:i32)  [unwired: 1 out]
        n67 = Increment(x=w55) -> (x+1=w56:i32)
        n68 = Equal?(x=w56, y=w46) -> (x = y?=w47:bool)
        n69 = case shown="False" w47 {
          tunnel: w56 -> [w110 w122]
          tunnel: [w111 w127] -> w54
          tunnel: w22 -> [w109 w118]
          tunnel: [w109 w116] -> w28
          frame False {
            w113 = 0  # Not Found
            n70 = Equal?(x=w110, y=w113) -> (x = y?=w112:bool)
            n71 = case shown="True" w112 {
              tunnel: w110 -> [w114 _]
              tunnel: [w114 w115] -> w111
              frame False {
              }
              frame True {
                w115 = 11  # CheckDAQ
                # "USUAL SCENARIO"
              }
            }
          }
          frame True {
            # "Before allowing data record to be saved,\nprompt user to validate."
            n72 = call "Get Last Record (SubVI).vi"("error in"=w118) -> ("error out"=w117:errorcluster, "experiment record"=w119:i32, "shot record"=w120:i32)  [unwired: 2 out]
            n73 = local write "LastShot"(w120) -> ()
            n74 = local write "LastSample"(w119) -> ()
            n75 = To Double Precision Float(number=w119) -> (double precision float=w121:dbl)
            n76 = Two Button Dialog(message="Are ALL Data Valid?", 1:"NO" ("F button name (\"Cancel\")"), 2:"YES" ("T button name (\"OK\")")) -> (T button?=w126:bool)
            n77 = property on="Record #" class="DigNum (strict)"(error in=w117, "Maximum"=w121) -> (error out=w116:errorcluster)  [unwired: 1 in, 1 out]
            n78 = case shown="True" w126 {
              tunnel: [0 ("index of element") w129] -> w127
              tunnel: w122 -> [_ w129]
              frame False {
                # "POLL"
              }
              frame True {
              }
            }
          }
        }
        n79 = To Variant(anything=w54) -> (Variant=w52:variant)
        n80 = Variant To Data(type=w53, Variant=w52) -> (data=w37:T13)  [unwired: 1 in, 1 out]
        "STOP (Shots MC LB)" <- TRUE ("STOP (Shots MC LB)")
      }
      frame 1 {
        # "This section reads the ini file"
        n81 = case shown="100" w138 {
          tunnel: [w144 w163] -> w139
          tunnel: [w142 w163] -> w134
          tunnel: w131 -> [w141 w155]
          tunnel: [w140 w155] -> w130
          frame 0, Default {
            n82 = local read "RESET All"() -> (w143:bool)
            n83 = case shown="True" w143 {
              tunnel: [TRUE w151] -> w144
              tunnel: [FALSE w151] -> w142
              tunnel: w141 -> [w145 w148]
              tunnel: [w145 w148] -> w140
              frame False {
                # "Refresh"
              }
              frame True {
                n84 = Two Button Dialog(message="Resetting will remove all unsaved data.\n\nDo you really  want to reset? ", 1:"NO" ("F button name (\"Cancel\")"), 2:"YES" ("T button name (\"OK\")")) -> (T button?=w151:bool)
              }
            }
          }
          frame 100 {
            w163 = TRUE  # Reset ALL
            n85 = property on="Loading" class="Ring (strict)"("Visible"=FALSE) -> ()  [unwired: 2 in, 2 out]
            n86 = control-ref of="Mfr_0"() -> (w153:refnum<vi>)
            n87 = control-ref of="Mfr_1"() -> (w162:refnum<vi>)
            n88 = control-ref of="Mfr_2"() -> (w161:refnum<vi>)
            n89 = control-ref of="Mfr_3"() -> (w160:refnum<vi>)
            n90 = control-ref of="Mfr_4"() -> (w159:refnum<vi>)
            n91 = control-ref of="Mfr_5"() -> (w158:refnum<vi>)
            n92 = control-ref of="Mfr_6"() -> (w157:refnum<vi>)
            n93 = Build Array(w153, w162, w161, w160, w159, w158, w157) -> (w156:refnum<vi>[])
            n94 = global write "BIMS_Collector Globals.vi" "Mfrs"(w156) -> ()
          }
        }
        n95 = case shown="True" w139 {
          tunnel: [Collector_State."POLL" ("progState") w201] -> w137
          tunnel: w136 -> [w166 _]
          tunnel: [w166 "SHOTS"] -> w135
          tunnel: w134 -> [_ w202]
          tunnel: [w164 w181] -> w132
          tunnel: w130 -> [w164 w200]
          frame False {
            n96 = local write "RESET All"(FALSE ("RESET")) -> ()
          }
          frame True {
            n97 = case shown="True" w202 {
              selector: w202 -> [_ w233]
              tunnel: [w216 w233] -> w182
              tunnel: [w215 w248] -> w183
              tunnel: w200 -> [w215 w235]
              tunnel: [w214 w232] -> w179
              frame False {
                w216 = FALSE  # Reset All
                # "Refresh"
                n98 = local read "configPath"() -> (w214:path)
              }
              frame True {
                # "This section resets\nentire program"
                # "Reset ALL"
                n99 = control-ref of="This VI"() -> (w225:refnum<vi>)
                n100 = invoke on="Invoke Node" class="VI" method="Default Vals.Reinit All"(reference=w225, error in=w235) -> (reference out=w224:refnum<vi>, error out=w223:errorcluster)  [unwired: 1 in, 1 out]
                n101 = property class="VI"(reference=w224, error in=w223, "Front Panel.ShowMenuBar"=FALSE ("Front Panel Window:Show Menu Bar")) -> (reference out=w221:refnum<vi>, error out=w219:errorcluster)
                n102 = property on="mainTabCntrl" class="TabCtl (strict)"() -> (error out=w227:errorcluster, "Pages"=w229:refnum<vi>[])  [unwired: 2 in, 1 out]
                n103 = control-ref of="ScreenSetAvgg"() -> (w243:refnum<vi>)
                n104 = control-ref of="InterlockExists"() -> (w244:refnum<vi>)
                n105 = control-ref of="useBallisitican"() -> (w245:refnum<vi>)
                n106 = control-ref of="useRecorder"() -> (w246:refnum<vi>)
                n107 = control-ref of="useShooter"() -> (w247:refnum<vi>)
                n108 = control-ref of="useBMC"() -> (w218:refnum<vi>)
                n109 = Close Reference(reference=w221, error in (no error)=w219) -> (error out=w220:errorcluster)
                n110 = Index Array(array=w229, index=1) -> (element=w231:refnum<vi>)
                n111 = call "RegReadParams.vi"("ScreenSetAveraging_Ref"=w243, "useBMC_Ref"=w218, "InterlockExist_Ref"=w244, "errorIN"=w220, "useShooter_Ref"=w247, "useRecorder_Ref"=w246, "useBallistician_Ref"=w245) -> ("error out"=w242:errorcluster)  [unwired: 4 out]
                n112 = control-ref of="Server"() -> (w234:refnum<vi>)
                n113 = control-ref of="ConfigName"() -> (w238:refnum<vi>)
                n114 = control-ref of="Site"() -> (w236:refnum<vi>)
                n115 = control-ref of="Folder"() -> (w217:refnum<vi>)
                n116 = property on="Property Node" class="Page"(reference=w231, error in=w227, "PageEnb"=T15."Page Disabled & Grayed" ("Page Enabled State")) -> (error out=w226:errorcluster)  [unwired: 1 out]
                n117 = Build Array(w238, w236, w234, w217) -> (w239:refnum<vi>[])
                n118 = call "InitStringValuesFromRegistry(SubVI).vi"("error in"=w242, "String References"=w239, "subkey"="SOFTWARE\\DuPont\\BIMS-08\\Collector", "root key (HKEY_LOCAL_MACHINE)"=Registry_RtKey."HKEY_LOCAL_MACHINE") -> ("error out"=w241:errorcluster)  [unwired: 3 out]
                n119 = property on="minV50" class="DigNum (strict)"(error in=w226, "Visible"=w233) -> ()  [unwired: 1 in, 2 out]
                n120 = Current VI's Path() -> (path=w251:path)
                n121 = call "Initialize (SubVI).vi"("path"=w251, "error IN"=w241) -> ("pathConfigOUT"=w232:path, "lengthUnits"=→"lengthUnits":string, "massUnits"=→"massUnits":string, "error out"=w248:errorcluster)  [unwired: 1 out]
                "configPath" <- w232
              }
            }
            n122 = control-ref of="Threat"() -> (w186:refnum<vi>)
            n123 = control-ref of="SampleTypes"() -> (w188:refnum<vi>)
            n124 = control-ref of="SampleDescrip"() -> (w195:refnum<vi>)
            n125 = call "Get Threats (SubVI).vi"("pathConfigIN"=w179, "refThreat"=w186, "error in"=w183) -> ("pathConfigOUT"=w190:path, "factorOut"=→"factor array":sgl[], "error out"=w193:errorcluster)  [unwired: 4 out]
            n126 = Bundle("SampleTypes"=w188, "SampleDescrip"=w195) -> (w194:T21)  [unwired: 1 out]
            n127 = call "Fill Lists from INI (SubVI).vi"("clusterListboxes"=w194, "error in"=w193, "pathConfigIN"=w190) -> ("error out"=w192:errorcluster, "pathConfigOUT"=w191:path)  [unwired: 4 out]
            n128 = call "Read Parameters.vi"("error in (no error)"=w192, "appended path"=w191) -> ("error out"=w185:errorcluster, "rangeParams"=w187:T22)  [unwired: 4 out]
            n129 = Unbundle(w187) -> ("max dev"=w168:sgl, "residual separation"=→"Residual/Separation":sgl, "Set#1 Separation"=→"Set#1 Separation":sgl, "Set#2 Separation"=→"Set#2 Separation":sgl, "impact target dist"=w172:sgl, "resid target dist"=w173:sgl, "barrel screen dist"=→"Barrel to Screen":sgl, "midpt_to_target_dist"=→"mid_to_targ_dist":sgl)
            n130 = property on="Ballisticians" class="Ring (strict)"("Visible"="useBallisitican") -> ()  [unwired: 2 in, 2 out]
            n131 = property on="Shooters" class="Ring (strict)"("Visible"="useShooter") -> ()  [unwired: 2 in, 2 out]
            n132 = property on="Recorders" class="Ring (strict)"("Visible"="useRecorder") -> ()  [unwired: 2 in, 2 out]
            n133 = property on="RefreshMetadata" class="Bool (strict)"(error in=w185, "Val(Sgnl)"=TRUE) -> (error out=w180:errorcluster)  [unwired: 1 in, 1 out]
            n134 = local write "Residual/Target Dist"(w173) -> ()
            n135 = local write "maxDev"(w168) -> ()
            n136 = local write "Set#1_to_Target"(w172) -> ()
            n137 = disable-structure shown="Disabled" {
              disable-tunnel: w180 -> [w205 w207]
              disable-tunnel: [w204 w207] -> w176
              frame Disabled {
                n138 = property on="rangeSetup" class="Ring (strict)"(error in=w205, "Val(Sgnl)"=u16 1 ("Value (Signaling)")) -> (error out=w204:errorcluster)  [unwired: 1 in, 1 out]
              }
              frame Enabled {
              }
            }
            n139 = case shown="True" w182 {
              tunnel: [Collector_State."POLL" ("progState") w277] -> w201
              tunnel: [w252 w262] -> w199
              tunnel: w176 -> [w252 w271]
              tunnel: w179 -> [_ w261]
              tunnel: "useBMC" -> [_ w260]
              frame False {
                # "Refresh"
              }
              frame True {
                w254 = T14."Disabled and Grayed Out" ("Disabled")
                # "Reset ALL"
                n140 = global read "BIMS_Collector Globals.vi" "SampleStyles"() -> (w264:refnum<vi>[])
                n141 = case shown="True" w260 {
                  tunnel: w261 -> [_ w279]
                  frame False {
                  }
                  frame True {
                    n142 = Path To String(path=w279) -> (string=w280:string)
                    n143 = call "Ballistics Message Center.vi"("INI File Name"=w280) -> ()
                  }
                }
                n144 = call "Get Last Record (SubVI).vi"("error in"=w271) -> ("error out"=w263:errorcluster, "experiment record"=w269:i32, "shot record"=→"LastShot":i32)  [unwired: 2 out]
                "LastSample" <- w269
                n145 = local read "MeasSrc"() -> (w278:T6)
                n146 = local read "InterlockExists"() -> (w276:bool)
                n147 = control-ref of="ThreatDetails"() -> (w259:refnum<vi>)
                n148 = control-ref of="SampleStyle_0"() -> (w266:refnum<vi>)
                n149 = control-ref of="ThreatGroups"() -> (w265:refnum<vi>)
                n150 = local read "SafetyInterlock"() -> (w274:cluster{"ARMED":bool})
                n151 = Bundle By Name(cluster=w274, "ARMED"=FALSE) -> (w273:cluster{"ARMED":bool})
                n152 = To Double Precision Float(number=w269) -> (double precision float=w268:dbl)
                n153 = property on="Record #" class="DigNum (strict)"(error in=w263, "Maximum"=w268) -> (error out=w262:errorcluster)  [unwired: 1 in, 1 out]
                n154 = case shown="\"Screens\"" w278 {
                  tunnel: [Collector_State."POLL" ("progState") Collector_State."POLL" ("progState") Collector_State."READY CLOCK" ("progState")] -> w277
                  frame "Simulated", Default {
                  }
                  frame "Radar" {
                  }
                  frame "Screens" {
                    # "check for PCI 6602"
                  }
                }
                n155 = Build Array (concatenate)(w259, w266, w265, w264) -> (w267:refnum<vi>[])
                n156 = local write "SafetyInterlock"(w273) -> ()
                n157 = Select(t=T14."Enabled" ("Disabled"), s=w276, f=T14."Disabled and Grayed Out" ("Disabled")) -> (s? t:f=w275:T14)
                n158 = for {
                  tunnel: w267 -> [w281] mode=indexing
                  n159 = property on="Property Node" class="Ring (strict)"(reference=w281, "Strings []"=string[] []) -> ()  [unwired: 1 in, 2 out]
                }
                n160 = property on="addShot" class="Bool"("Disabled"=T14."Enabled") -> ()  [unwired: 2 in, 2 out]
                n161 = property on="undoLastShot" class="Bool"("Disabled"=w254) -> ()  [unwired: 2 in, 2 out]
                n162 = property on="saveShots" class="Bool"("Disabled"=w254) -> ()  [unwired: 2 in, 2 out]
                n163 = property on="clearShots" class="Bool"("Disabled"=w254) -> ()  [unwired: 2 in, 2 out]
                n164 = property on="ARM" class="Bool"("Disabled"=w275) -> ()  [unwired: 2 in, 2 out]
                n165 = property on="SafetyInterlock" class="Clust (strict)"("Disabled"=w275) -> ()  [unwired: 2 in, 2 out]
                n166 = property on="saveReq" class="Str"("Visible"=TRUE) -> ()  [unwired: 2 in, 2 out]
              }
            }
            n167 = call <vilib>:"General Error Handler.vi"("error in (no error)"=w199) -> ("error out"=w181:errorcluster)  [unwired: 2 in, 12 out]
            n168 = flat-sequence {
              tunnel: w181 -> [w208]
              frame #0 {
                n169 = local read "ConfigName"() -> (w209:string)
                n170 = case shown="No Error" w208 {
                  tunnel: [w212 "NOT READY!" ("ConfigName")] -> w210
                  tunnel: w209 -> [w212 _]
                  frame No Error {
                    n171 = Wait (ms)(milliseconds to wait=u32 1000) -> ()  [unwired: 1 out]
                  }
                  frame Error {
                  }
                }
                "ConfigName" <- w210
              }
            }
            "saveReq" <- "Number of layers in sample ply specification and number of shots in shots table must be greater than 0 to enable saving." ("saveReq")
          }
        }
      }
      frame 2 {
        w319 = TRUE  # Enable
        # "The custom Excel template file is \nexpected in the C:\\Ballistics folder."
        n172 = case shown="False" "lookupRec" {
          selector: "lookupRec" -> [_ w799]
          tunnel: [w336 w786] -> w317
          tunnel: [w335 w772] -> w316
          tunnel: [w334 w789] -> w315
          tunnel: [w333 w791] -> w314
          tunnel: [w332 w787] -> w313
          tunnel: [w331 w749] -> w312
          tunnel: [w330 w736] -> w299
          tunnel: [w329 w738] -> w298
          tunnel: [w328 w739] -> w297
          tunnel: [w327 "Record #"] -> w296
          tunnel: [w326 w788] -> w295
          tunnel: [w325 w738] -> w288
          tunnel: w293 -> [w324 _]
          tunnel: [w323 w761] -> w291
          tunnel: w290 -> [w323 w762]
          tunnel: [w322 w733] -> w286
          frame False {
            n173 = stacked-sequence {
              tunnel: [_ _ _ _ _ w659] -> w331
              tunnel: [_ w398 _ _ _ _] -> w335
              tunnel: [_ _ _ _ w503 _] -> w332
              tunnel: [_ _ _ w449 _ _] -> w333
              tunnel: [_ _ w420 _ _ _] -> w334
              tunnel: [w342 _ _ _ _ _] -> w336
              tunnel: [_ _ _ _ _ w665] -> w330
              tunnel: [_ _ _ _ _ w661] -> w329
              tunnel: [_ _ _ _ _ w660] -> w328
              tunnel: [_ _ _ _ _ w664] -> w327
              tunnel: [_ _ _ _ _ w663] -> w326
              tunnel: [_ _ _ _ _ w662] -> w325
              tunnel: w324 -> [_ _ w419 _ w502 _]
              frame #0 {
                # "FABRIC"
                n174 = local read "fab1_totalWt"() -> (w345:sgl)
                n175 = local read "fab3_totalWt"() -> (w347:sgl)
                n176 = local read "fab5_totalWt"() -> (w349:sgl)
                n177 = global read "BIMS_Collector Globals.vi" "LayerStitchTypeRefs"() -> (w337:refnum<vi>[])
                n178 = global read "BIMS_Collector Globals.vi" "SampleAttribs"() -> (w338:T23)
                n179 = global read "BIMS_Collector Globals.vi" "SampleStyles"() -> (w340:refnum<vi>[])
                n180 = global read "BIMS_Collector Globals.vi" "LayerSpecs"() -> (w339:T24)
                n181 = global read "BIMS_Collector Globals.vi" "Mfrs"() -> (w341:refnum<vi>[])
                n182 = local read "fab2_totalWt"() -> (w346:sgl)
                n183 = local read "fab4_totalWt"() -> (w348:sgl)
                n184 = local read "fab6_totalWt"() -> (w350:sgl)
                n185 = Build Array(w345, w346, w347, w348, w349, w350) -> (w344:sgl[])
                n186 = for {
                  tunnel: w344 -> [w352] mode=indexing
                  tunnel: [w358] -> w343 mode=indexing
                  tunnel: w338 -> [w356] mode=indexing
                  tunnel: w339 -> [w355] mode=indexing
                  tunnel: w341 -> [w354] mode=indexing
                  tunnel: w340 -> [w353] mode=indexing
                  tunnel: w337 -> [w351] mode=indexing
                  n187 = Less Or Equal To 0?(x=w352) -> (x <= 0?=w357:bool)
                  n188 = case shown="False" w357 {
                    tunnel: [w380 w382] -> w358
                    tunnel: w356 -> [w379 _]
                    tunnel: w355 -> [w364 _]
                    tunnel: w354 -> [w373 _]
                    tunnel: w353 -> [w370 _]
                    tunnel: w352 -> [w363 _]
                    tunnel: w351 -> [w359 _]
                    frame False {
                      n189 = Unbundle By Name(w364) -> ("numOfPlies"=w362:i32, "LotNum"=w376:string, "RollNum"=w377:string)
                      n190 = Unbundle By Name(w379) -> ("internal_ID"=w367:string, "fiber"=w368:string, "denier"=w375:string, "pick"=w374:string, "weave"=w365:string, "finish"=w366:string, "ozPerYd2"=w378:string)
                      n191 = Format Into String(w362) -> (resulting string=w372:string)  [unwired: 3 in, 1 out]
                      n192 = call "Dropdown Selection (SubVI).vi"("reference"=w373) -> ("element"=w371:string)
                      n193 = call "Dropdown Selection (SubVI).vi"("reference"=w370) -> ("element"=w369:string)
                      n194 = Format Into String(w363) -> (resulting string=w361:string)  [unwired: 3 in, 1 out]
                      n195 = call "Dropdown Selection (SubVI).vi"("reference"=w359) -> ("element"=w360:string)
                      n196 = Build Array(w372, w371, w369, w367, w368, w375, w374, w365, w366, w376, w377, w378, w361, w360) -> (w380:string[])
                    }
                    frame True {
                      n197 = call <vilib>:"Space Constant.vi"() -> ("String"=w383:string)
                      n198 = Initialize Array(w383, 12 ("dimension size")) -> (w382:string[])
                    }
                  }
                }
                n199 = Transpose 2D Array(2D array=w343) -> (transposed array=w342:string[][])
              }
              frame #1 {
                w384 = "%.1f" ("format string")
                # "muzzel / midpoint"
                # "muzzle / scr#1"
                # "muzzle / target"
                # "scr#2 / target"
                # "RANGE"
                n200 = local read "Set#1 Separation"() -> (w391:sgl)
                n201 = local read "mid_to_targ_dist"() -> (w388:sgl)
                n202 = local read "Barrel to Screen"() -> (w385:sgl)
                n203 = local read "clayAverage"() -> (w406:sgl)
                n204 = Divide(x=w391, y=sgl 2.0) -> (x/y=w386:sgl)
                n205 = local read "RoomHum"() -> (w401:sgl)
                n206 = local read "clayTemp"() -> (w404:sgl)
                n207 = local read "clayCalib"() -> (w407:string)
                n208 = local read "RoomT"() -> (w402:sgl)
                n209 = Add(x=w385, y=w388) -> (x+y=w392:sgl)
                n210 = Subtract(x=w385, y=w386) -> (x-y=w387:sgl)
                n211 = Subtract(x=w388, y=w386) -> (x-y=w389:sgl)
                n212 = Format Into String(w392) -> (resulting string=w393:string)  [unwired: 3 in, 1 out]
                n213 = Format Into String(w387) -> (resulting string=w394:string)  [unwired: 3 in, 1 out]
                n214 = Format Into String(w391) -> (resulting string=w395:string)  [unwired: 3 in, 1 out]
                n215 = Format Into String(w389) -> (resulting string=w396:string)  [unwired: 3 in, 1 out]
                n216 = Format Into String(w388) -> (resulting string=w397:string)  [unwired: 3 in, 1 out]
                n217 = Format Into String(w401) -> (resulting string=w399:string)  [unwired: 3 in, 1 out]
                n218 = Format Into String(format string=w384, w402) -> (resulting string=w400:string)  [unwired: 2 in, 1 out]
                n219 = Format Into String(format string=w384, w404) -> (resulting string=w403:string)  [unwired: 2 in, 1 out]
                n220 = Format Into String(format string=w384, w406) -> (resulting string=w405:string)  [unwired: 2 in, 1 out]
                n221 = Bundle(w393, w394, w395, w396, w397, w399, w400, w403, "clayCalib"=w407, w405) -> (w408:T25)  [unwired: 1 out]
                n222 = Cluster To Array(cluster=w408) -> (array=w398:string[])
              }
              frame #2 {
                # "RESULTS"
                n223 = control-ref of="Methods"() -> (w409:refnum<vi>)
                n224 = call "Dropdown Selection (SubVI).vi"("reference"=w409) -> ("element"=w410:string)
                n225 = for {
                  tunnel: w419 -> [w447] mode=indexing
                  tunnel: [w446] -> w418 mode=indexing
                  tunnel: [w445] -> w417
                  i -> [w445]
                  n226 = Unbundle By Name(w447) -> ("BackFace\nDepth"=w446:sgl)
                }
                n227 = Increment(x=w417) -> (x+1=w415:i32)
                n228 = Add Array Elements(numeric array=w418) -> (sum=w416:sgl)
                n229 = To Single Precision Float(number=w415) -> (single precision float=w414:sgl)
                n230 = Divide(x=w416, y=w414) -> (x/y=w413:sgl)
                n231 = Format Into String(format string="%1.1f", w413) -> (resulting string=w412:string)  [unwired: 2 in, 1 out]
                n232 = case shown="\"V50\"" w410 {
                  tunnel: [w435 w444] -> w422
                  tunnel: w412 -> [w423 w443]
                  frame "V50" {
                    w429 = "%1d" ("format string")
                    n233 = local read "Z.M.R."() -> (w427:sgl)
                    n234 = Less Than 0?(x=w427) -> (x < 0?=w428:bool)
                    n235 = local read "rangeOfResults"() -> (w431:i32)
                    n236 = local read "computed_V50"() -> (w434:sgl)
                    n237 = local read "lowComplete"() -> (w432:i32)
                    n238 = local read "highPartial"() -> (w433:i32)
                    n239 = case shown="True" w428 {
                      tunnel: w427 -> [w440 _]
                      tunnel: [w440 sgl 0.0 ("Z.M.R.")] -> w426
                      frame False {
                      }
                      frame True {
                      }
                    }
                    n240 = Format Into String(format string="%1.1f", w434) -> (resulting string=w438:string)  [unwired: 2 in, 1 out]
                    n241 = Format Into String(format string=w429, w433) -> (resulting string=w437:string)  [unwired: 2 in, 1 out]
                    n242 = Format Into String(format string=w429, w432) -> (resulting string=w436:string)  [unwired: 2 in, 1 out]
                    n243 = Format Into String(format string=w429, w431) -> (resulting string=w439:string)  [unwired: 2 in, 1 out]
                    n244 = Format Into String(format string="%1.1f", w426) -> (resulting string=w425:string)  [unwired: 2 in, 1 out]
                    n245 = Bundle(w438, w437, w436, w439, w425, w423, w423) -> (w435:T26)  [unwired: 1 out]
                  }
                  frame Default {
                    w442 = "" ("Empty String Constant")
                    n246 = Bundle(w442, w442, w442, w442, w442, w443, w443) -> (w444:T26)  [unwired: 1 out]
                  }
                }
                n247 = Cluster To Array(cluster=w422) -> (array=w421:string[])
                n248 = Build Array(w421) -> (w420:string[][])
              }
              frame #3 {
                # "SAMPLE"
                n249 = local read "Site"() -> (w448:string)
                n250 = case shown="\"SPR1\"" w448 {
                  tunnel: [w451 w475 w488] -> w449
                  frame "ICE1", Default {
                    # "PB Req"
                    n251 = control-ref of="Methods"() -> (w452:refnum<vi>)
                    n252 = call "Dropdown Selection (SubVI).vi"("reference"=w452) -> ("element"=w454:string)
                    n253 = Equal?(x=w454, y="V50") -> (x = y?=w453:bool)
                    n254 = local read "totalSampleWt"() -> (w464:sgl)
                    n255 = case shown="True" w453 {
                      tunnel: ["n/a" w474] -> w458
                      frame False {
                      }
                      frame True {
                        n256 = local read "minV50"() -> (w473:i32)
                        n257 = Format Into String(w473) -> (resulting string=w474:string)  [unwired: 3 in, 1 out]
                      }
                    }
                    n258 = control-ref of="SampleDimensions"() -> (w470:refnum<vi>)
                    n259 = control-ref of="SampleCoverings"() -> (w471:refnum<vi>)
                    n260 = control-ref of="Models"() -> (w457:refnum<vi>)
                    n261 = local read "serialNum"() -> (w466:string)
                    n262 = local read "SampleID"() -> (w468:string)
                    n263 = local read "Thickness"() -> (w461:dbl)
                    n264 = local read "totalBAW"() -> (w460:sgl)
                    n265 = call "Dropdown Selection (SubVI).vi"("reference"=w470) -> ("element"=w467:string)
                    n266 = call "Dropdown Selection (SubVI).vi"("reference"=w457) -> ("element"=w456:string)
                    n267 = call "Dropdown Selection (SubVI).vi"("reference"=w471) -> ("element"=w465:string)
                    n268 = Format Into String(w464) -> (resulting string=w463:string)  [unwired: 3 in, 1 out]
                    n269 = Format Into String(w461) -> (resulting string=w462:string)  [unwired: 3 in, 1 out]
                    n270 = Format Into String(w460) -> (resulting string=w459:string)  [unwired: 3 in, 1 out]
                    n271 = Bundle("SampleID"=w468, "element"=w467, "Type of work"="Type of work", "serialNum"=w466, "element"=w456, w463, w462, w459, "element"=w465, w458) -> (w469:T27)  [unwired: 1 out]
                    n272 = Cluster To Array(cluster=w469) -> (array=w451:string[])
                  }
                  frame "SPR0" {
                    n273 = local read "totalSampleWt"() -> (w481:sgl)
                    n274 = control-ref of="SampleDimensions"() -> (w486:refnum<vi>)
                    n275 = control-ref of="SampleCoverings"() -> (w487:refnum<vi>)
                    n276 = local read "SampleID"() -> (w484:string)
                    n277 = local read "Thickness"() -> (w478:dbl)
                    n278 = local read "totalBAW"() -> (w477:sgl)
                    n279 = call "Dropdown Selection (SubVI).vi"("reference"=w486) -> ("element"=w483:string)
                    n280 = call "Dropdown Selection (SubVI).vi"("reference"=w487) -> ("element"=w482:string)
                    n281 = Format Into String(w481) -> (resulting string=w480:string)  [unwired: 3 in, 1 out]
                    n282 = Format Into String(w478) -> (resulting string=w479:string)  [unwired: 3 in, 1 out]
                    n283 = Format Into String(w477) -> (resulting string=w476:string)  [unwired: 3 in, 1 out]
                    n284 = Bundle("SampleID"=w484, "element"=w483, w480, w479, w476, "element"=w482) -> (w485:T28)  [unwired: 1 out]
                    n285 = Cluster To Array(cluster=w485) -> (array=w475:string[])
                  }
                  frame "SPR1" {
                    n286 = local read "totalSampleWt"() -> (w494:sgl)
                    n287 = control-ref of="SampleDimensions"() -> (w499:refnum<vi>)
                    n288 = control-ref of="SampleCoverings"() -> (w500:refnum<vi>)
                    n289 = local read "SampleID"() -> (w497:string)
                    n290 = local read "Thickness"() -> (w491:dbl)
                    n291 = local read "totalBAW"() -> (w490:sgl)
                    n292 = call "Dropdown Selection (SubVI).vi"("reference"=w499) -> ("element"=w496:string)
                    n293 = call "Dropdown Selection (SubVI).vi"("reference"=w500) -> ("element"=w495:string)
                    n294 = Format Into String(w494) -> (resulting string=w493:string)  [unwired: 3 in, 1 out]
                    n295 = Format Into String(w491) -> (resulting string=w492:string)  [unwired: 3 in, 1 out]
                    n296 = Format Into String(w490) -> (resulting string=w489:string)  [unwired: 3 in, 1 out]
                    n297 = Bundle("SampleID"=w497, "element"=w496, w493, w492, w489, "element"=w495) -> (w498:T28)  [unwired: 1 out]
                    n298 = Cluster To Array(cluster=w498) -> (array=w488:string[])
                  }
                }
              }
              frame #4 {
                n299 = local read "Site"() -> (w501:string)
                n300 = case shown="\"ICE1\", Default" w501 {
                  tunnel: [w513 w563 w615] -> w503
                  tunnel: w502 -> [w506 w556 w608]
                  frame "ICE1", Default {
                    # "SHOT TABLE"
                    n301 = control-ref of="Methods"() -> (w505:refnum<vi>)
                    n302 = call "Dropdown Selection (SubVI).vi"("reference"=w505) -> ("element"=w504:string)
                    n303 = for {
                      tunnel: w506 -> [w545] mode=indexing
                      shift-right: [w522] -> _
                      shift-left: T17 [] -> [w524]
                      tunnel: [w522] -> w509
                      tunnel: w504 -> [w518]
                      n304 = Unbundle By Name(w545) -> ("shot order"=w544:i32, "Powder Loading"=w543:sgl, "Uncorrected Impact"=w542:sgl, "UncorrectedRed_PB"=w541:sgl, "UncorrectedAvgVel_PB"=w540:sgl, "velLoss_PB"=w539:sgl, "strikeVel_PB"=w538:sgl, "SHOT STATUS"=w527:u16, "usedv50"=w537:bool, "Shot Angle"=w519:u16, "BackFace\nDepth"=w520:sgl)
                      n305 = case shown="\"V50\"" w518 {
                        tunnel: w537 -> [w547 _]
                        tunnel: [w546 w551] -> w536
                        tunnel: w519 -> [_ w550]
                        frame "V50" {
                          n306 = case shown="True" w547 {
                            tunnel: ["" ("Empty String Constant") "*"] -> w546
                            frame False {
                            }
                            frame True {
                            }
                          }
                        }
                        frame Default {
                          n307 = Format Into String(w550) -> (resulting string=w551:string)  [unwired: 3 in, 1 out]
                        }
                      }
                      n308 = case shown="1" w527 {
                        tunnel: ["P" "C"] -> w526
                        frame 0, Default {
                        }
                        frame 1 {
                        }
                      }
                      n309 = Format Into String(format string="%2d", w544) -> (resulting string=w529:string)  [unwired: 2 in, 1 out]
                      n310 = Format Into String(w543) -> (resulting string=w530:string)  [unwired: 3 in, 1 out]
                      n311 = Format Into String(w542) -> (resulting string=w531:string)  [unwired: 3 in, 1 out]
                      n312 = Format Into String(w541) -> (resulting string=w532:string)  [unwired: 3 in, 1 out]
                      n313 = Format Into String(w540) -> (resulting string=w533:string)  [unwired: 3 in, 1 out]
                      n314 = Format Into String(w539) -> (resulting string=w534:string)  [unwired: 3 in, 1 out]
                      n315 = Format Into String(w538) -> (resulting string=w535:string)  [unwired: 3 in, 1 out]
                      n316 = Format Into String(w520) -> (resulting string=w528:string)  [unwired: 3 in, 1 out]
                      n317 = Build Array(w529, w530, w531, w532, w533, w534, w535, w526, w536, w528) -> (w523:string[])
                      n318 = Array To Cluster(array=w523) -> (cluster=w525:T29)
                      n319 = Build Array (concatenate)(w524, w525) -> (w522:T17)
                    }
                    n320 = Array Size(array=w509) -> (size(s)=w511:i32)
                    n321 = Equal To 0?(x=w511) -> (x = 0?=w507:bool)
                    n322 = case shown="True" w507 {
                      tunnel: [w514 T17 [{"[0]"="", "[1]"="", "[2]"="", "[3]"="", "[4]"="", "[5]"="", "[6]"="", "[7]"="", "[8]"="", "[9]"=""}]] -> w508
                      tunnel: w509 -> [w514 _]
                      frame False {
                      }
                      frame True {
                      }
                    }
                    n323 = Sort 1D Array(array=w508) -> (sorted array=w510:T17)
                    n324 = for {
                      tunnel: w510 -> [w517] mode=indexing
                      tunnel: [w516] -> w513 mode=indexing
                      n325 = Cluster To Array(cluster=w517) -> (array=w516:string[])
                    }
                  }
                  frame "SPR0" {
                    # "SHOT TABLE"
                    n326 = control-ref of="Methods"() -> (w555:refnum<vi>)
                    n327 = call "Dropdown Selection (SubVI).vi"("reference"=w555) -> ("element"=w554:string)
                    n328 = for {
                      tunnel: w556 -> [w593] mode=indexing
                      shift-right: [w574] -> _
                      shift-left: T18 [] -> [w576]
                      tunnel: [w574] -> w559
                      tunnel: w554 -> [w570]
                      n329 = Unbundle By Name(w593) -> ("shot order"=w592:i32, "Powder Loading"=w591:sgl, "Uncorrected Impact"=w590:sgl, "UncorrectedRed_PB"=w589:sgl, "strikeVel_PB"=w588:sgl, "SHOT STATUS"=w579:u16, "usedv50"=w587:bool, "Shot Angle"=w571:u16, "BackFace\nDepth"=w572:sgl, "V50userExcl"=w569:bool, "Shot Description"=w568:string)
                      n330 = case shown="\"V50\"" w570 {
                        tunnel: w587 -> [w596 _]
                        tunnel: [w595 w603] -> w586
                        tunnel: w571 -> [_ w602]
                        tunnel: w569 -> [w594 _]
                        frame "V50" {
                          n331 = case shown="True" w594 {
                            tunnel: w596 -> [w598 _]
                            tunnel: [w597 "!"] -> w595
                            frame False {
                              n332 = case shown="False" w598 {
                                tunnel: ["" ("Empty String Constant") "*"] -> w597
                                frame False {
                                }
                                frame True {
                                }
                              }
                            }
                            frame True {
                            }
                          }
                        }
                        frame Default {
                          n333 = Format Into String(w602) -> (resulting string=w603:string)  [unwired: 3 in, 1 out]
                        }
                      }
                      n334 = case shown="1" w579 {
                        tunnel: ["P" "C"] -> w578
                        frame 0, Default {
                        }
                        frame 1 {
                        }
                      }
                      n335 = Format Into String(format string="%2d", w592) -> (resulting string=w581:string)  [unwired: 2 in, 1 out]
                      n336 = Format Into String(w591) -> (resulting string=w582:string)  [unwired: 3 in, 1 out]
                      n337 = Format Into String(w590) -> (resulting string=w583:string)  [unwired: 3 in, 1 out]
                      n338 = Format Into String(w589) -> (resulting string=w584:string)  [unwired: 3 in, 1 out]
                      n339 = Format Into String(w588) -> (resulting string=w585:string)  [unwired: 3 in, 1 out]
                      n340 = Format Into String(w572) -> (resulting string=w580:string)  [unwired: 3 in, 1 out]
                      n341 = Build Array(w581, w582, w583, w584, w585, w578, w586, w580, w568) -> (w575:string[])
                      n342 = Array To Cluster(array=w575) -> (cluster=w577:T30)
                      n343 = Build Array (concatenate)(w576, w577) -> (w574:T18)
                    }
                    n344 = Array Size(array=w559) -> (size(s)=w561:i32)
                    n345 = Equal To 0?(x=w561) -> (x = 0?=w557:bool)
                    n346 = case shown="True" w557 {
                      tunnel: [w564 T18 [{"[0]"="", "[1]"="", "[2]"="", "[3]"="", "[4]"="", "[5]"="", "[6]"="", "[7]"="", "[8]"=""}]] -> w558
                      tunnel: w559 -> [w564 _]
                      frame False {
                      }
                      frame True {
                      }
                    }
                    n347 = Sort 1D Array(array=w558) -> (sorted array=w560:T18)
                    n348 = for {
                      tunnel: w560 -> [w567] mode=indexing
                      tunnel: [w566] -> w563 mode=indexing
                      n349 = Cluster To Array(cluster=w567) -> (array=w566:string[])
                    }
                  }
                  frame "SPR1" {
                    # "SHOT TABLE"
                    n350 = control-ref of="Methods"() -> (w607:refnum<vi>)
                    n351 = call "Dropdown Selection (SubVI).vi"("reference"=w607) -> ("element"=w606:string)
                    n352 = for {
                      tunnel: w608 -> [w645] mode=indexing
                      shift-right: [w626] -> _
                      shift-left: T18 [] -> [w628]
                      tunnel: [w626] -> w611
                      tunnel: w606 -> [w622]
                      n353 = Unbundle By Name(w645) -> ("shot order"=w644:i32, "Powder Loading"=w643:sgl, "Uncorrected Impact"=w642:sgl, "UncorrectedRed_PB"=w641:sgl, "strikeVel_PB"=w640:sgl, "SHOT STATUS"=w631:u16, "usedv50"=w639:bool, "Shot Angle"=w623:u16, "BackFace\nDepth"=w624:sgl, "V50userExcl"=w621:bool, "Shot Description"=w620:string)
                      n354 = case shown="\"V50\"" w622 {
                        tunnel: w639 -> [w648 _]
                        tunnel: [w647 w655] -> w638
                        tunnel: w623 -> [_ w654]
                        tunnel: w621 -> [w646 _]
                        frame "V50" {
                          n355 = case shown="True" w646 {
                            tunnel: w648 -> [w650 _]
                            tunnel: [w649 "!"] -> w647
                            frame False {
                              n356 = case shown="False" w650 {
                                tunnel: ["" ("Empty String Constant") "*"] -> w649
                                frame False {
                                }
                                frame True {
                                }
                              }
                            }
                            frame True {
                            }
                          }
                        }
                        frame Default {
                          n357 = Format Into String(w654) -> (resulting string=w655:string)  [unwired: 3 in, 1 out]
                        }
                      }
                      n358 = case shown="1" w631 {
                        tunnel: ["P" "C"] -> w630
                        frame 0, Default {
                        }
                        frame 1 {
                        }
                      }
                      n359 = Format Into String(format string="%2d", w644) -> (resulting string=w633:string)  [unwired: 2 in, 1 out]
                      n360 = Format Into String(w643) -> (resulting string=w634:string)  [unwired: 3 in, 1 out]
                      n361 = Format Into String(w642) -> (resulting string=w635:string)  [unwired: 3 in, 1 out]
                      n362 = Format Into String(w641) -> (resulting string=w636:string)  [unwired: 3 in, 1 out]
                      n363 = Format Into String(w640) -> (resulting string=w637:string)  [unwired: 3 in, 1 out]
                      n364 = Format Into String(w624) -> (resulting string=w632:string)  [unwired: 3 in, 1 out]
                      n365 = Build Array(w633, w634, w635, w636, w637, w630, w638, w632, w620) -> (w627:string[])
                      n366 = Array To Cluster(array=w627) -> (cluster=w629:T30)
                      n367 = Build Array (concatenate)(w628, w629) -> (w626:T18)
                    }
                    n368 = Array Size(array=w611) -> (size(s)=w613:i32)
                    n369 = Equal To 0?(x=w613) -> (x = 0?=w609:bool)
                    n370 = case shown="True" w609 {
                      tunnel: [w616 T18 [{"[0]"="", "[1]"="", "[2]"="", "[3]"="", "[4]"="", "[5]"="", "[6]"="", "[7]"="", "[8]"=""}]] -> w610
                      tunnel: w611 -> [w616 _]
                      frame False {
                      }
                      frame True {
                      }
                    }
                    n371 = Sort 1D Array(array=w610) -> (sorted array=w612:T18)
                    n372 = for {
                      tunnel: w612 -> [w619] mode=indexing
                      tunnel: [w618] -> w615 mode=indexing
                      n373 = Cluster To Array(cluster=w619) -> (array=w618:string[])
                    }
                  }
                }
              }
              frame #5 {
                n374 = local read "Site"() -> (w658:string)
                n375 = case shown="\"SPR1\"" w658 {
                  tunnel: [w689 w710 w730] -> w665
                  tunnel: [w688 w709 w729] -> w664
                  tunnel: [w687 w708 w728] -> w663
                  tunnel: [w686 w693 w713] -> w662
                  tunnel: ["" ("projNum") w693 w713] -> w661
                  tunnel: [w684 w707 w727] -> w660
                  tunnel: [w668 w696 w716] -> w659
                  frame "ICE1", Default {
                    # "THREAT"
                    # "Range # (supports a PB reporting requirement)"
                    # "Project Name goes here.\nSupports a PB reporting requirement."
                    # "GENERAL"
                    n376 = local read "threatDetails"() -> (w667:T1)
                    n377 = Unbundle By Name(w667) -> ("barrelLength"=w671:string)
                    n378 = Unbundle By Name(w667) -> ("grainSize"=w666:string)
                    n379 = local read "Shot Angle"() -> (w672:u16)
                    n380 = control-ref of="WeaponTypes"() -> (w681:refnum<vi>)
                    n381 = control-ref of="ThreatGroups"() -> (w680:refnum<vi>)
                    n382 = control-ref of="PowderTypes"() -> (w679:refnum<vi>)
                    n383 = control-ref of="Recorders"() -> (w682:refnum<vi>)
                    n384 = control-ref of="Shooters"() -> (w683:refnum<vi>)
                    n385 = Format Into String(w672) -> (resulting string=w673:string)  [unwired: 3 in, 1 out]
                    n386 = call "Dropdown Selection (SubVI).vi"("reference"=w681) -> ("element"=w677:string)
                    n387 = call "Dropdown Selection (SubVI).vi"("reference"=w680) -> ("element"=w676:string)
                    n388 = call "Dropdown Selection (SubVI).vi"("reference"=w679) -> ("element"=w675:string)
                    n389 = call "Dropdown Selection (SubVI).vi"("reference"=w682) -> ("element"=w674:string)
                    n390 = call "Dropdown Selection (SubVI).vi"("reference"=w683) -> ("element"=w670:string)
                    n391 = local read "Comments"() -> (w687:string)
                    n392 = local read "ProjectID"() -> (w684:string)
                    n393 = local read "LastSample"() -> (w692:i32)
                    n394 = Bundle("element"=w677, "element"=w676, "grainSize"=w666, "element"=w675, "barrelLength"=w671, w673, "element"="1", "element"=w670, "element"=w674) -> (w678:T31)  [unwired: 1 out]
                    n395 = control-ref of="TestStandards"() -> (w691:refnum<vi>)
                    n396 = control-ref of="Methods"() -> (w690:refnum<vi>)
                    n397 = Cluster To Array(cluster=w678) -> (array=w668:string[])
                    n398 = call "Dropdown Selection (SubVI).vi"("reference"=w691) -> ("element"=w686:string)
                    n399 = call "Dropdown Selection (SubVI).vi"("reference"=w690) -> ("element"=w689:string)
                    n400 = Increment(x=w692) -> (x+1=w688:i32)
                  }
                  frame "SPR0" {
                    w693 = "" ("projNum")
                    # "THREAT"
                    # "Project Name goes here.\nSupports a PB reporting requirement."
                    # "GENERAL"
                    n401 = local read "threatDetails"() -> (w695:T1)
                    n402 = Unbundle By Name(w695) -> ("barrelLength"=w698:string)
                    n403 = Unbundle By Name(w695) -> ("grainSize"=w694:string)
                    n404 = local read "Shot Angle"() -> (w699:u16)
                    n405 = control-ref of="ThreatGroups"() -> (w705:refnum<vi>)
                    n406 = control-ref of="PowderTypes"() -> (w704:refnum<vi>)
                    n407 = control-ref of="Ballisticians"() -> (w706:refnum<vi>)
                    n408 = Format Into String(w699) -> (resulting string=w700:string)  [unwired: 3 in, 1 out]
                    n409 = call "Dropdown Selection (SubVI).vi"("reference"=w705) -> ("element"=w702:string)
                    n410 = call "Dropdown Selection (SubVI).vi"("reference"=w704) -> ("element"=w701:string)
                    n411 = call "Dropdown Selection (SubVI).vi"("reference"=w706) -> ("element"=w697:string)
                    n412 = local read "Comments"() -> (w708:string)
                    n413 = local read "ProjectID"() -> (w707:string)
                    n414 = local read "LastSample"() -> (w712:i32)
                    n415 = Bundle("element"=w702, "grainSize"=w694, "element"=w701, "barrelLength"=w698, w700, "element"=w697) -> (w703:T32)  [unwired: 1 out]
                    n416 = control-ref of="Methods"() -> (w711:refnum<vi>)
                    n417 = Cluster To Array(cluster=w703) -> (array=w696:string[])
                    n418 = call "Dropdown Selection (SubVI).vi"("reference"=w711) -> ("element"=w710:string)
                    n419 = Increment(x=w712) -> (x+1=w709:i32)
                  }
                  frame "SPR1" {
                    w713 = "" ("projNum")
                    # "THREAT"
                    # "Project Name goes here.\nSupports a PB reporting requirement."
                    # "GENERAL"
                    n420 = local read "threatDetails"() -> (w715:T1)
                    n421 = Unbundle By Name(w715) -> ("barrelLength"=w718:string)
                    n422 = Unbundle By Name(w715) -> ("grainSize"=w714:string)
                    n423 = local read "Shot Angle"() -> (w719:u16)
                    n424 = control-ref of="ThreatGroups"() -> (w725:refnum<vi>)
                    n425 = control-ref of="PowderTypes"() -> (w724:refnum<vi>)
                    n426 = control-ref of="Ballisticians"() -> (w726:refnum<vi>)
                    n427 = Format Into String(w719) -> (resulting string=w720:string)  [unwired: 3 in, 1 out]
                    n428 = call "Dropdown Selection (SubVI).vi"("reference"=w725) -> ("element"=w722:string)
                    n429 = call "Dropdown Selection (SubVI).vi"("reference"=w724) -> ("element"=w721:string)
                    n430 = call "Dropdown Selection (SubVI).vi"("reference"=w726) -> ("element"=w717:string)
                    n431 = local read "Comments"() -> (w728:string)
                    n432 = local read "ProjectID"() -> (w727:string)
                    n433 = local read "LastSample"() -> (w732:i32)
                    n434 = Bundle("element"=w722, "grainSize"=w714, "element"=w721, "barrelLength"=w718, w720, "element"=w717) -> (w723:T32)  [unwired: 1 out]
                    n435 = control-ref of="Methods"() -> (w731:refnum<vi>)
                    n436 = Cluster To Array(cluster=w723) -> (array=w716:string[])
                    n437 = call "Dropdown Selection (SubVI).vi"("reference"=w731) -> ("element"=w730:string)
                    n438 = Increment(x=w732) -> (x+1=w729:i32)
                  }
                }
              }
            }
            n439 = Get Date/Time String() -> (date string=w322:string)  [unwired: 3 in, 1 out]
          }
          frame True {
            w738 = ""
            # "date"
            # "method"
            # "general"
            # "remark"
            # "threat"
            # "shots"
            # "sample"
            # "results"
            # "range"
            # "fabric"
            # "query db with the entered record number and use result to populate the xlt"
            n440 = Not(x=w799) -> (.not. x?=w798:bool)
            n441 = local write "lookupRec"(w798) -> ()
            n442 = Format Into String(format string="SELECT * FROM Experiments\nWHERE expt=%d;" ("query string"), error in=w762, "Record #") -> (resulting string=w795:string, error out=w763:errorcluster)  [unwired: 1 in]
            n443 = call "Fetch Data (SubVI).vi"("error IN"=w763, "query string"=w795) -> ("error OUT"=w761:errorcluster, "recordset data"=w797:string[][])  [unwired: 4 out]
            n444 = Index Array(array=w797) -> (element=w734:string[])  [unwired: 2 in]
            n445 = Index Array(array=w734, index=111) -> (element=w765:string)
            n446 = local read "Set#1 Separation"() -> (w779:sgl)
            n447 = call "Load Shots (SubVI).vi"("Record #"="Record #", "Method"=w765) -> ("Shot Array"=w787:string[][], "AvgDef"=w770:dbl)  [unwired: 1 in]
            n448 = local read "mid_to_targ_dist"() -> (w782:sgl)
            n449 = local read "Barrel to Screen"() -> (w785:sgl)
            n450 = Format Into String(w770) -> (resulting string=w768:string)  [unwired: 3 in, 1 out]
            n451 = Match Pattern(string=w765, regular expression="N.I.J.") -> (offset past match=w767:i32)  [unwired: 4 out]
            n452 = Greater Or Equal To 0?(x=w767) -> (x >= 0?=w764:bool)
            n453 = Divide(x=w779, y=sgl 2.0) -> (x/y=w784:sgl)
            n454 = case shown="False" w764 {
              tunnel: [w810 w811] -> w769
              tunnel: w768 -> [w807 w813]
              tunnel: w734 -> [w809 _]
              frame False {
                n455 = Index Array(array=w809, index #1=94 ("index"), index #2=119 ("index"), index #5=115 ("index")) -> (element #1=w808:string, element #2=w806:string, element #3=w805:string, element #4=w804:string, element #5=w803:string)  [unwired: 2 in]
                n456 = Build Array(w808, w806, w805, w804, w803, w807) -> (w810:string[])
              }
              frame True {
                w812 = "" ("Empty String Constant")
                n457 = Build Array(w812, w812, w812, w812, w812, w813, w813) -> (w811:string[])
              }
            }
            n458 = Add(x=w785, y=w782) -> (x+y=w778:sgl)
            n459 = Subtract(x=w785, y=w784) -> (x-y=w783:sgl)
            n460 = Subtract(x=w782, y=w784) -> (x-y=w781:sgl)
            n461 = Index Array(array=w734, index #1=91 ("index"), index #2=89 ("index"), index #3=97 ("index"), index #4=12 ("index"), index #5=7 ("index")) -> (element #1=w750:string, element #2=w748:string, element #3=w747:string, element #4=w744:string, element #5=w743:string)
            n462 = Index Array(array=w734, index #1=113 ("index"), index #2=112 ("index"), index #3=103 ("index")) -> (element #1=w759:string, element #2=w758:string, element #3=w757:string, element #4=w756:string, element #5=w752:string)  [unwired: 2 in]
            n463 = Format Into String(w778) -> (resulting string=w777:string)  [unwired: 3 in, 1 out]
            n464 = Format Into String(w783) -> (resulting string=w776:string)  [unwired: 3 in, 1 out]
            n465 = Format Into String(w779) -> (resulting string=w775:string)  [unwired: 3 in, 1 out]
            n466 = Format Into String(w781) -> (resulting string=w774:string)  [unwired: 3 in, 1 out]
            n467 = Format Into String(w782) -> (resulting string=w773:string)  [unwired: 3 in, 1 out]
            n468 = Build Array(w750, w748, w747, "", w744, w743) -> (w749:string[])
            n469 = Array Subset(array=w734, index=5, length=1) -> (w791:string[])
            n470 = Build Array(w777, w776, w775, w774, w773, w759, w758, w757, w756, w752) -> (w772:string[])
            n471 = Index Array(array=w734, index #1=4 ("index"), index #2=111 ("index")) -> (element #1=w739:string, element #2=w736:string)
            n472 = Index Array(array=w734, index=107) -> (element=w788:string)
            n473 = Index Array(array=w734, index=2) -> (element=w733:string)
            n474 = Build Array(w769) -> (w789:string[][])
            n475 = call "Get Model Construction.vi"("panel record"=w734) -> ("Fabric Array"=w786:string[][])
          }
        }
        n476 = To Variant(anything=w317) -> (Variant=w311:variant)
        n477 = To Variant(anything=w316) -> (Variant=w310:variant)
        n478 = To Variant(anything=w315) -> (Variant=w309:variant)
        n479 = To Variant(anything=w314) -> (Variant=w308:variant)
        n480 = To Variant(anything=w313) -> (Variant=w307:variant)
        n481 = To Variant(anything=w312) -> (Variant=w306:variant)
        n482 = To Variant(anything=w299) -> (Variant=w305:variant)
        n483 = To Variant(anything=w298) -> (Variant=w304:variant)
        n484 = To Variant(anything=w297) -> (Variant=w303:variant)
        n485 = To Variant(anything=w296) -> (Variant=w300:variant)
        n486 = To Variant(anything=w295) -> (Variant=w301:variant)
        n487 = To Variant(anything=w288) -> (Variant=w302:variant)
        n488 = To Variant(anything=w286) -> (Variant=w287:variant)
        n489 = call "TestReport_XL.vi"("Enable"=w319, "blockFabric"=w311, "blockRange"=w310, "blockResults"=w309, "blockSample"=w308, "blockShotTbl"=w307, "error in (no error)"=w291, "blockThreat"=w306, "testDate"=w287, "method"=w305, "projName"=w304, "projNum"=w303, "recNum"=w300, "remark"=w301, "standard"=w302) -> ("error out"=w318:errorcluster)  [unwired: 4 in, 8 out]
        n490 = call <vilib>:"Simple Error Handler.vi"("error in (no error)"=w318) -> ("error out"=w320:errorcluster)  [unwired: 1 in, 7 out]
        n491 = case shown="Error" w320 {
          selector: w320 -> [w814 w816]
          tunnel: [w814 w816] -> w289
          frame No Error {
            n492 = One Button Dialog(message=" V50 Ballistic Test Report is ready") -> ()  [unwired: 2 out]
          }
          frame Error {
          }
        }
      }
      frame 3 {
        w846 = TRUE  # Enable
        # "The custom Excel template file is \nexpected in the C:\\Ballistics folder."
        n493 = stacked-sequence {
          tunnel: [_ _ _ _ _ w1037] -> w839
          tunnel: [_ w910 _ _ _ _] -> w843
          tunnel: [_ _ _ _ w994 _] -> w840
          tunnel: [_ _ _ w961 _ _] -> w841
          tunnel: [_ _ w932 _ _ _] -> w842
          tunnel: [w854 _ _ _ _ _] -> w844
          tunnel: [_ _ _ _ _ w1058] -> w826
          tunnel: [_ _ _ _ _ "" ("projNum")] -> w825
          tunnel: [_ _ _ _ _ w1053] -> w824
          tunnel: [_ _ _ _ _ w1057] -> w823
          tunnel: [_ _ _ _ _ w1056] -> w822
          tunnel: [_ _ _ _ _ w1055] -> w821
          tunnel: w820 -> [_ _ w931 _ w987 _]
          frame #0 {
            # "FABRIC"
            n494 = local read "fab1_totalWt"() -> (w857:sgl)
            n495 = local read "fab3_totalWt"() -> (w859:sgl)
            n496 = local read "fab5_totalWt"() -> (w861:sgl)
            n497 = global read "BIMS_Collector Globals.vi" "LayerStitchTypeRefs"() -> (w849:refnum<vi>[])
            n498 = global read "BIMS_Collector Globals.vi" "SampleAttribs"() -> (w850:T23)
            n499 = global read "BIMS_Collector Globals.vi" "SampleStyles"() -> (w852:refnum<vi>[])
            n500 = local read "fab2_totalWt"() -> (w858:sgl)
            n501 = local read "fab4_totalWt"() -> (w860:sgl)
            n502 = local read "fab6_totalWt"() -> (w862:sgl)
            n503 = global read "BIMS_Collector Globals.vi" "LayerSpecs"() -> (w851:T24)
            n504 = global read "BIMS_Collector Globals.vi" "Mfrs"() -> (w853:refnum<vi>[])
            n505 = Build Array(w857, w858, w859, w860, w861, w862) -> (w856:sgl[])
            n506 = for {
              tunnel: w856 -> [w864] mode=indexing
              tunnel: [w870] -> w855 mode=indexing
              tunnel: w850 -> [w868] mode=indexing
              tunnel: w851 -> [w867] mode=indexing
              tunnel: w853 -> [w866] mode=indexing
              tunnel: w852 -> [w865] mode=indexing
              tunnel: w849 -> [w863] mode=indexing
              n507 = Less Or Equal To 0?(x=w864) -> (x <= 0?=w869:bool)
              n508 = case shown="False" w869 {
                tunnel: [w892 w894] -> w870
                tunnel: w868 -> [w891 _]
                tunnel: w867 -> [w876 _]
                tunnel: w866 -> [w885 _]
                tunnel: w865 -> [w882 _]
                tunnel: w864 -> [w875 _]
                tunnel: w863 -> [w871 _]
                frame False {
                  n509 = Unbundle By Name(w876) -> ("numOfPlies"=w874:i32, "LotNum"=w888:string, "RollNum"=w889:string)
                  n510 = Unbundle By Name(w891) -> ("internal_ID"=w879:string, "fiber"=w880:string, "denier"=w887:string, "pick"=w886:string, "weave"=w877:string, "finish"=w878:string, "ozPerYd2"=w890:string)
                  n511 = Format Into String(w874) -> (resulting string=w884:string)  [unwired: 3 in, 1 out]
                  n512 = call "Dropdown Selection (SubVI).vi"("reference"=w885) -> ("element"=w883:string)
                  n513 = call "Dropdown Selection (SubVI).vi"("reference"=w882) -> ("element"=w881:string)
                  n514 = call "Dropdown Selection (SubVI).vi"("reference"=w871) -> ("element"=w872:string)
                  n515 = Format Into String(w875) -> (resulting string=w873:string)  [unwired: 3 in, 1 out]
                  n516 = Build Array(w884, w883, w881, w879, w880, w887, w886, w877, w878, w888, w889, w890, w873, w872) -> (w892:string[])
                }
                frame True {
                  n517 = call <vilib>:"Space Constant.vi"() -> ("String"=w895:string)
                  n518 = Initialize Array(w895, 12 ("dimension size")) -> (w894:string[])
                }
              }
            }
            n519 = Transpose 2D Array(2D array=w855) -> (transposed array=w854:string[][])
          }
          frame #1 {
            w896 = "%.1f" ("format string")
            # "muzzel / midpoint"
            # "muzzle / scr#1"
            # "muzzle / target"
            # "scr#2 / target"
            # "RANGE"
            n520 = local read "Set#1 Separation"() -> (w903:sgl)
            n521 = local read "mid_to_targ_dist"() -> (w900:sgl)
            n522 = local read "Barrel to Screen"() -> (w897:sgl)
            n523 = local read "clayAverage"() -> (w918:sgl)
            n524 = Divide(x=w903, y=sgl 2.0) -> (x/y=w898:sgl)
            n525 = local read "RoomHum"() -> (w913:sgl)
            n526 = local read "clayTemp"() -> (w916:sgl)
            n527 = local read "clayCalib"() -> (w919:string)
            n528 = local read "RoomT"() -> (w914:sgl)
            n529 = Add(x=w897, y=w900) -> (x+y=w904:sgl)
            n530 = Subtract(x=w897, y=w898) -> (x-y=w899:sgl)
            n531 = Subtract(x=w900, y=w898) -> (x-y=w901:sgl)
            n532 = Format Into String(w904) -> (resulting string=w905:string)  [unwired: 3 in, 1 out]
            n533 = Format Into String(w899) -> (resulting string=w906:string)  [unwired: 3 in, 1 out]
            n534 = Format Into String(w903) -> (resulting string=w907:string)  [unwired: 3 in, 1 out]
            n535 = Format Into String(w901) -> (resulting string=w908:string)  [unwired: 3 in, 1 out]
            n536 = Format Into String(w900) -> (resulting string=w909:string)  [unwired: 3 in, 1 out]
            n537 = Format Into String(w913) -> (resulting string=w911:string)  [unwired: 3 in, 1 out]
            n538 = Format Into String(format string=w896, w914) -> (resulting string=w912:string)  [unwired: 2 in, 1 out]
            n539 = Format Into String(format string=w896, w916) -> (resulting string=w915:string)  [unwired: 2 in, 1 out]
            n540 = Format Into String(format string=w896, w918) -> (resulting string=w917:string)  [unwired: 2 in, 1 out]
            n541 = Bundle(w905, w906, w907, w908, w909, w911, w912, w915, "clayCalib"=w919, w917) -> (w920:T25)  [unwired: 1 out]
            n542 = Cluster To Array(cluster=w920) -> (array=w910:string[])
          }
          frame #2 {
            # "RESULTS"
            n543 = control-ref of="Methods"() -> (w921:refnum<vi>)
            n544 = call "Dropdown Selection (SubVI).vi"("reference"=w921) -> ("element"=w922:string)
            n545 = for {
              tunnel: w931 -> [w959] mode=indexing
              tunnel: [w958] -> w930 mode=indexing
              tunnel: [w957] -> w929
              i -> [w957]
              n546 = Unbundle By Name(w959) -> ("BackFace\nDepth"=w958:sgl)
            }
            n547 = Increment(x=w929) -> (x+1=w927:i32)
            n548 = Add Array Elements(numeric array=w930) -> (sum=w928:sgl)
            n549 = To Single Precision Float(number=w927) -> (single precision float=w926:sgl)
            n550 = Divide(x=w928, y=w926) -> (x/y=w925:sgl)
            n551 = Format Into String(format string="%1.1f", w925) -> (resulting string=w924:string)  [unwired: 2 in, 1 out]
            n552 = case shown="\"V50\"" w922 {
              tunnel: [w947 w956] -> w934
              tunnel: w924 -> [w935 w955]
              frame "V50" {
                w941 = "%1d" ("format string")
                n553 = local read "Z.M.R."() -> (w939:sgl)
                n554 = Less Than 0?(x=w939) -> (x < 0?=w940:bool)
                n555 = local read "rangeOfResults"() -> (w943:i32)
                n556 = local read "computed_V50"() -> (w946:sgl)
                n557 = local read "lowComplete"() -> (w944:i32)
                n558 = local read "highPartial"() -> (w945:i32)
                n559 = case shown="True" w940 {
                  tunnel: w939 -> [w952 _]
                  tunnel: [w952 sgl 0.0 ("Z.M.R.")] -> w938
                  frame False {
                  }
                  frame True {
                  }
                }
                n560 = Format Into String(format string="%1.1f", w946) -> (resulting string=w950:string)  [unwired: 2 in, 1 out]
                n561 = Format Into String(format string=w941, w945) -> (resulting string=w949:string)  [unwired: 2 in, 1 out]
                n562 = Format Into String(format string=w941, w944) -> (resulting string=w948:string)  [unwired: 2 in, 1 out]
                n563 = Format Into String(format string=w941, w943) -> (resulting string=w951:string)  [unwired: 2 in, 1 out]
                n564 = Format Into String(format string="%1.1f", w938) -> (resulting string=w937:string)  [unwired: 2 in, 1 out]
                n565 = Bundle(w950, w949, w948, w951, w937, w935, w935) -> (w947:T26)  [unwired: 1 out]
              }
              frame Default {
                w954 = "" ("Empty String Constant")
                n566 = Bundle(w954, w954, w954, w954, w954, w955, w955) -> (w956:T26)  [unwired: 1 out]
              }
            }
            n567 = Cluster To Array(cluster=w934) -> (array=w933:string[])
            n568 = Build Array(w933) -> (w932:string[][])
          }
          frame #3 {
            # "PB Req"
            # "SAMPLE"
            n569 = control-ref of="Methods"() -> (w962:refnum<vi>)
            n570 = call "Dropdown Selection (SubVI).vi"("reference"=w962) -> ("element"=w964:string)
            n571 = Equal?(x=w964, y="V50") -> (x = y?=w963:bool)
            n572 = local read "totalSampleWt"() -> (w974:sgl)
            n573 = case shown="True" w963 {
              tunnel: ["n/a" w984] -> w968
              frame False {
              }
              frame True {
                n574 = local read "minV50"() -> (w983:i32)
                n575 = Format Into String(w983) -> (resulting string=w984:string)  [unwired: 3 in, 1 out]
              }
            }
            n576 = local read "Type of work"() -> (w960:string)
            n577 = control-ref of="SampleDimensions"() -> (w980:refnum<vi>)
            n578 = control-ref of="SampleCoverings"() -> (w981:refnum<vi>)
            n579 = control-ref of="Models"() -> (w967:refnum<vi>)
            n580 = local read "serialNum"() -> (w976:string)
            n581 = local read "SampleID"() -> (w978:string)
            n582 = local read "Thickness"() -> (w971:dbl)
            n583 = local read "totalBAW"() -> (w970:sgl)
            n584 = call "Dropdown Selection (SubVI).vi"("reference"=w980) -> ("element"=w977:string)
            n585 = call "Dropdown Selection (SubVI).vi"("reference"=w967) -> ("element"=w966:string)
            n586 = call "Dropdown Selection (SubVI).vi"("reference"=w981) -> ("element"=w975:string)
            n587 = Format Into String(w974) -> (resulting string=w973:string)  [unwired: 3 in, 1 out]
            n588 = Format Into String(w971) -> (resulting string=w972:string)  [unwired: 3 in, 1 out]
            n589 = Format Into String(w970) -> (resulting string=w969:string)  [unwired: 3 in, 1 out]
            n590 = Bundle("SampleID"=w978, "element"=w977, "Type of work"=w960, "serialNum"=w976, "element"=w966, w973, w972, w969, "element"=w975, w968) -> (w979:T27)  [unwired: 1 out]
            n591 = Cluster To Array(cluster=w979) -> (array=w961:string[])
          }
          frame #4 {
            # "SHOT TABLE"
            n592 = control-ref of="Methods"() -> (w986:refnum<vi>)
            n593 = call "Dropdown Selection (SubVI).vi"("reference"=w986) -> ("element"=w985:string)
            n594 = for {
              tunnel: w987 -> [w1026] mode=indexing
              shift-right: [w1003] -> _
              shift-left: T17 [] -> [w1005]
              tunnel: [w1003] -> w990
              tunnel: w985 -> [w999]
              n595 = Unbundle By Name(w1026) -> ("shot order"=w1025:i32, "Powder Loading"=w1024:sgl, "Uncorrected Impact"=w1023:sgl, "UncorrectedRed_PB"=w1022:sgl, "UncorrectedAvgVel_PB"=w1021:sgl, "velLoss_PB"=w1020:sgl, "strikeVel_PB"=w1019:sgl, "SHOT STATUS"=w1008:u16, "usedv50"=w1018:bool, "Shot Angle"=w1000:u16, "BackFace\nDepth"=w1001:sgl)
              n596 = case shown="\"V50\"" w999 {
                tunnel: w1018 -> [w1028 _]
                tunnel: [w1027 w1032] -> w1017
                tunnel: w1000 -> [_ w1031]
                frame "V50" {
                  n597 = case shown="True" w1028 {
                    tunnel: ["" ("Empty String Constant") "*"] -> w1027
                    frame False {
                    }
                    frame True {
                    }
                  }
                }
                frame Default {
                  n598 = Format Into String(w1031) -> (resulting string=w1032:string)  [unwired: 3 in, 1 out]
                }
              }
              n599 = case shown="1" w1008 {
                tunnel: ["P" "C"] -> w1007
                frame 0, Default {
                }
                frame 1 {
                }
              }
              n600 = Format Into String(format string="%2d", w1025) -> (resulting string=w1010:string)  [unwired: 2 in, 1 out]
              n601 = Format Into String(w1024) -> (resulting string=w1011:string)  [unwired: 3 in, 1 out]
              n602 = Format Into String(w1023) -> (resulting string=w1012:string)  [unwired: 3 in, 1 out]
              n603 = Format Into String(w1022) -> (resulting string=w1013:string)  [unwired: 3 in, 1 out]
              n604 = Format Into String(w1021) -> (resulting string=w1014:string)  [unwired: 3 in, 1 out]
              n605 = Format Into String(w1020) -> (resulting string=w1015:string)  [unwired: 3 in, 1 out]
              n606 = Format Into String(w1019) -> (resulting string=w1016:string)  [unwired: 3 in, 1 out]
              n607 = Format Into String(w1001) -> (resulting string=w1009:string)  [unwired: 3 in, 1 out]
              n608 = Build Array(w1010, w1011, w1012, w1013, w1014, w1015, w1016, w1007, w1017, w1009) -> (w1004:string[])
              n609 = Array To Cluster(array=w1004) -> (cluster=w1006:T29)
              n610 = Build Array (concatenate)(w1005, w1006) -> (w1003:T17)
            }
            n611 = Array Size(array=w990) -> (size(s)=w992:i32)
            n612 = Equal To 0?(x=w992) -> (x = 0?=w988:bool)
            n613 = case shown="True" w988 {
              tunnel: [w995 T17 [{"[0]"="", "[1]"="", "[2]"="", "[3]"="", "[4]"="", "[5]"="", "[6]"="", "[7]"="", "[8]"="", "[9]"=""}]] -> w989
              tunnel: w990 -> [w995 _]
              frame False {
              }
              frame True {
              }
            }
            n614 = Sort 1D Array(array=w989) -> (sorted array=w991:T17)
            n615 = for {
              tunnel: w991 -> [w998] mode=indexing
              tunnel: [w997] -> w994 mode=indexing
              n616 = Cluster To Array(cluster=w998) -> (array=w997:string[])
            }
          }
          frame #5 {
            # "THREAT"
            # "Range # (supports a PB reporting requirement)"
            # "Project Name goes here.\nSupports a PB reporting requirement."
            # "GENERAL"
            n617 = local read "threatDetails"() -> (w1036:T1)
            n618 = Unbundle By Name(w1036) -> ("barrelLength"=w1040:string)
            n619 = Unbundle By Name(w1036) -> ("grainSize"=w1035:string)
            n620 = local read "Shot Angle"() -> (w1041:u16)
            n621 = control-ref of="WeaponTypes"() -> (w1050:refnum<vi>)
            n622 = control-ref of="ThreatGroups"() -> (w1049:refnum<vi>)
            n623 = control-ref of="PowderTypes"() -> (w1048:refnum<vi>)
            n624 = control-ref of="Recorders"() -> (w1051:refnum<vi>)
            n625 = control-ref of="Shooters"() -> (w1052:refnum<vi>)
            n626 = Format Into String(w1041) -> (resulting string=w1042:string)  [unwired: 3 in, 1 out]
            n627 = call "Dropdown Selection (SubVI).vi"("reference"=w1050) -> ("element"=w1046:string)
            n628 = call "Dropdown Selection (SubVI).vi"("reference"=w1049) -> ("element"=w1045:string)
            n629 = call "Dropdown Selection (SubVI).vi"("reference"=w1048) -> ("element"=w1044:string)
            n630 = call "Dropdown Selection (SubVI).vi"("reference"=w1051) -> ("element"=w1043:string)
            n631 = call "Dropdown Selection (SubVI).vi"("reference"=w1052) -> ("element"=w1039:string)
            n632 = Bundle("element"=w1046, "element"=w1045, "grainSize"=w1035, "element"=w1044, "barrelLength"=w1040, w1042, "element"="1", "element"=w1039, "element"=w1043) -> (w1047:T31)  [unwired: 1 out]
            n633 = Cluster To Array(cluster=w1047) -> (array=w1037:string[])
            n634 = local read "Comments"() -> (w1056:string)
            n635 = local read "ProjectID"() -> (w1053:string)
            n636 = local read "LastSample"() -> (w1061:i32)
            n637 = control-ref of="TestStandards"() -> (w1060:refnum<vi>)
            n638 = control-ref of="Methods"() -> (w1059:refnum<vi>)
            n639 = call "Dropdown Selection (SubVI).vi"("reference"=w1060) -> ("element"=w1055:string)
            n640 = call "Dropdown Selection (SubVI).vi"("reference"=w1059) -> ("element"=w1058:string)
            n641 = Increment(x=w1061) -> (x+1=w1057:i32)
          }
        }
        n642 = To Variant(anything=w844) -> (Variant=w838:variant)
        n643 = To Variant(anything=w843) -> (Variant=w837:variant)
        n644 = To Variant(anything=w842) -> (Variant=w836:variant)
        n645 = To Variant(anything=w841) -> (Variant=w835:variant)
        n646 = To Variant(anything=w840) -> (Variant=w834:variant)
        n647 = To Variant(anything=w839) -> (Variant=w833:variant)
        n648 = To Variant(anything=w826) -> (Variant=w832:variant)
        n649 = To Variant(anything=w825) -> (Variant=w831:variant)
        n650 = To Variant(anything=w824) -> (Variant=w830:variant)
        n651 = To Variant(anything=w823) -> (Variant=w827:variant)
        n652 = To Variant(anything=w822) -> (Variant=w828:variant)
        n653 = To Variant(anything=w821) -> (Variant=w829:variant)
        n654 = call "TestReport_XL.vi"("Enable"=w846, "blockFabric"=w838, "blockRange"=w837, "blockResults"=w836, "blockSample"=w835, "blockShotTbl"=w834, "error in (no error)"=w818, "blockThreat"=w833, "method"=w832, "projName"=w831, "projNum"=w830, "recNum"=w827, "remark"=w828, "standard"=w829) -> ("error out"=w845:errorcluster)  [unwired: 5 in, 8 out]
        n655 = call <vilib>:"Simple Error Handler.vi"("error in (no error)"=w845) -> ("error out"=w847:errorcluster)  [unwired: 1 in, 7 out]
        n656 = case shown="No Error" w847 {
          selector: w847 -> [w1062 w1064]
          tunnel: [w1062 w1064] -> w817
          frame No Error {
            n657 = One Button Dialog(message=" VsVr Ballistic Test Report is ready") -> ()  [unwired: 2 out]
          }
          frame Error {
          }
        }
      }
      frame 4 {
        # "This section saves the shots to the data base"
        n658 = stacked-sequence {
          seq-local: [w1130 _ _] -> [_ w1216 _]
          seq-local: [w1132 _ _] -> [_ w1213 _]
          seq-local: [_ w1201 _] -> [_ _ w1230]
          seq-local: [_ w1203 _] -> [_ _ w1229]
          seq-local: [w1128 _ _] -> [_ _ w1222]
          seq-local: [w1102 _ _] -> [_ w1159 _]
          tunnel: [_ _ w1224] -> w1070
          tunnel: [_ _ w1227] -> w1071
          tunnel: w1066 -> [_ w1168 w1221]
          tunnel: w1068 -> [w1104 _ _]
          tunnel: ["SampleDescrip" _ _] -> _
          tunnel: ["Areal Density" _ _] -> _
          tunnel: ["Areal density text" _ _] -> _
          tunnel: ["SoftwareVersion" _ _] -> _
          tunnel: ["Fabric Description" _ _] -> _
          tunnel: ["Threat" _ _] -> _
          tunnel: ["old threat" _ _] -> _
          tunnel: ["line direction map" _ _] -> _
          tunnel: ["Methods" _ _] -> _
          tunnel: ["SampleCoverings" _ _] -> _
          tunnel: ["Ballisticians" _ _] -> _
          tunnel: ["Submitters" _ _] -> _
          tunnel: ["SampleDimensions" _ _] -> _
          tunnel: ["PowderTypes" _ _] -> _
          tunnel: ["SampleTypes" _ _] -> _
          tunnel: ["TestConditions" _ _] -> _
          tunnel: ["ModelMfrs" _ _] -> _
          tunnel: ["Assemblers" _ _] -> _
          tunnel: ["N.I.J" _ _] -> _
          tunnel: ["SampleClamping" _ _] -> _
          tunnel: ["FrontLayer" _ _] -> _
          tunnel: ["BackLayer" _ _] -> _
          frame #0 {
            # "Legacy requirements:"
            # "Shared requirements:"
            n659 = local read "fab1_totalWt"() -> (w1140:sgl)
            n660 = local read "fab2_totalWt"() -> (w1139:sgl)
            n661 = local read "fab3_totalWt"() -> (w1138:sgl)
            n662 = local read "fab4_totalWt"() -> (w1137:sgl)
            n663 = local read "fab5_totalWt"() -> (w1136:sgl)
            n664 = local read "fab6_totalWt"() -> (w1135:sgl)
            n665 = Build Array(w1140, w1139, w1138, w1137, w1136, w1135) -> (w1134:sgl[])
            n666 = call "SQL Statement for Sample Descritpion.vi"("error IN"=w1104, "Layer Weight Array"=w1134, "VALUES clause IN"=" VALUES (%d " ("SQL statement IN"), "INSERT clause IN"="INSERT INTO Experiments " ("SQL statement IN")) -> ("error OUT"=w1103:errorcluster, "VALUES clause OUT"=w1133:string, "INSERT clause OUT"=w1131:string)  [unwired: 1 out]
            n667 = local read "LastSample"() -> (w1129:i32)
            n668 = Increment(x=w1129) -> (x+1=w1128:i32)
            n669 = local read "rangeOfResults"() -> (w1106:i32)
            n670 = local read "lowComplete"() -> (w1107:i32)
            n671 = local read "clayAverage"() -> (w1109:sgl)
            n672 = local read "highPartial"() -> (w1108:i32)
            n673 = control-ref of="SampleClamping"() -> (w1101:refnum<vi>)
            n674 = control-ref of="BackLayer"() -> (w1077:refnum<vi>)
            n675 = control-ref of="FrontLayer"() -> (w1076:refnum<vi>)
            n676 = control-ref of="Ballisticians"() -> (w1123:refnum<vi>)
            n677 = control-ref of="Shooters"() -> (w1119:refnum<vi>)
            n678 = control-ref of="Recorders"() -> (w1118:refnum<vi>)
            n679 = control-ref of="Submitters"() -> (w1122:refnum<vi>)
            n680 = control-ref of="SampleCoverings"() -> (w1115:refnum<vi>)
            n681 = control-ref of="ThreatGroups"() -> (w1114:refnum<vi>)
            n682 = call "Dropdown Selection (SubVI).vi"("reference"=w1123) -> ("element"=w1121:string)
            n683 = call "Dropdown Selection (SubVI).vi"("reference"=w1119) -> ("element"=w1117:string)
            n684 = call "Dropdown Selection (SubVI).vi"("reference"=w1118) -> ("element"=w1116:string)
            n685 = call "Dropdown Selection (SubVI).vi"("reference"=w1122) -> ("element"=w1120:string)
            n686 = call "Dropdown Selection (SubVI).vi"("reference"=w1115) -> ("element"=w1113:string)
            n687 = call "Dropdown Selection (SubVI).vi"("reference"=w1114) -> ("element"=w1112:string)
            n688 = call "Dropdown Selection (SubVI).vi"("reference"=w1101) -> ("element"=w1100:string)
            n689 = call "Dropdown Selection (SubVI).vi"("reference"=w1077) -> ("element"=w1075:string)
            n690 = call "Dropdown Selection (SubVI).vi"("reference"=w1076) -> ("element"=w1074:string)
            n691 = flat-sequence {
              tunnel: ["TestStandards"] -> _
              tunnel: ["Shooters"] -> _
              tunnel: ["Recorders"] -> _
              tunnel: ["WeaponTypes"] -> _
              tunnel: ["Models"] -> _
              tunnel: ["serialNum"] -> _
              tunnel: ["layerStitch_1"] -> _
              tunnel: ["layerStitch_2"] -> _
              tunnel: ["layerStitch_3"] -> _
              tunnel: ["layerStitch_4"] -> _
              tunnel: ["layerStitch_5"] -> _
              tunnel: ["layerStitch_6"] -> _
              tunnel: ["minV50"] -> _
              frame #0 {
                # "PB-only requirements:"
              }
            }
            n692 = Concatenate Strings(w1131, ", expt, [date], Ballistician1, Ballistician2, Ballistician3, Submitter1, SampleCovering, ProjectileType, ClayTemp, ClayCalibration, ClayAvgThickness, highPartial, lowComplete, rangeOfResults, clamping, FrontPly, BackPly," ("Substring")) -> (w1130:string)
            n693 = Format Into String(format string=", %d, #%s#, '%s', '%s', '%s', '%s', '%s', '%s', %.1f, '%s', %.1f, %d, %d, %d, '%s', '%s', '%s'" ("Format String"), initial string=w1133, error in=w1103, w1128, "currentDateTime", w1121, w1117, w1116, w1120, w1113, w1112, "clayTemp", "clayCalib", w1109, w1108, w1107, w1106, w1100, w1075, w1074) -> (resulting string=w1132:string, error out=w1102:errorcluster)
          }
          frame #1 {
            w1215 = " Angle, Conditions, SampleType, ThreatGrain, ThreatDetail, V50dc, V50, maker, thickness, powder, numshots, backing, totalnumberplys, testcomments, NIJ1, method, temperature, humidity, Dimensions, zmr, ProjectID, SampleID, panelmaker, panelWeight, totalBAW)"  # INSERT clause continued
            # "Although shot angle is defined for the overall\nexperiment, it is also recorded for each shot."
            n694 = local read "computed_V50"() -> (w1211:sgl)
            n695 = local read "Drag Corrected"() -> (w1206:bool)
            n696 = local read "Impact factor"() -> (w1208:sgl)
            n697 = Array Size(array=w1168) -> (size(s)=w1199:i32)
            n698 = Select(t=w1208, s=w1206, f=sgl 1.0) -> (s? t:f=w1207:sgl)
            n699 = Divide(x=w1211, y=w1207) -> (x/y=w1210:sgl)
            n700 = control-ref of="ModelMfrs"() -> (w1194:refnum<vi>)
            n701 = control-ref of="PowderTypes"() -> (w1192:refnum<vi>)
            n702 = call "Dropdown Selection (SubVI).vi"("reference"=w1194) -> ("element"=w1193:string)
            n703 = call "Dropdown Selection (SubVI).vi"("reference"=w1192) -> ("element"=w1176:string)
            n704 = local read "GrainSize"() -> (w1157:u16)
            n705 = local read "Z.M.R."() -> (w1182:sgl)
            n706 = local read "Shot Angle"() -> (w1170:u16)
            n707 = Less Than 0?(x=w1182) -> (x < 0?=w1181:bool)
            n708 = local read "totalNumLayers"() -> (w1198:i32)
            n709 = control-ref of="ThreatDetails"() -> (w1154:refnum<vi>)
            n710 = control-ref of="SampleTypes"() -> (w1164:refnum<vi>)
            n711 = control-ref of="TestConditions"() -> (w1183:refnum<vi>)
            n712 = control-ref of="SampleBackings"() -> (w1191:refnum<vi>)
            n713 = Format Into String(w1157) -> (resulting string=w1156:string)  [unwired: 3 in, 1 out]
            n714 = local read "totalBAW"() -> (w1184:sgl)
            n715 = case shown="True" w1181 {
              tunnel: w1182 -> [w1219 _]
              tunnel: [w1219 sgl 0.0 ("Z.M.R.")] -> w1180
              frame False {
              }
              frame True {
              }
            }
            n716 = control-ref of="SampleDimensions"() -> (w1187:refnum<vi>)
            n717 = control-ref of="N.I.J"() -> (w1189:refnum<vi>)
            n718 = control-ref of="Methods"() -> (w1174:refnum<vi>)
            n719 = control-ref of="Assemblers"() -> (w1185:refnum<vi>)
            n720 = call "Dropdown Selection (SubVI).vi"("reference"=w1154) -> ("element"=w1155:string)
            n721 = call "Dropdown Selection (SubVI).vi"("reference"=w1164) -> ("element"=w1163:string)
            n722 = call "Dropdown Selection (SubVI).vi"("reference"=w1183) -> ("element"=w1169:string)
            n723 = call "Dropdown Selection (SubVI).vi"("reference"=w1191) -> ("element"=w1190:string)
            n724 = Equal?(x=w1156, y="") -> (x = y?=w1178:bool)
            n725 = call "Dropdown Selection (SubVI).vi"("reference"=w1189) -> ("element"=w1188:string)
            n726 = call "Dropdown Selection (SubVI).vi"("reference"=w1174) -> ("element"=w1173:string)
            n727 = call "Dropdown Selection (SubVI).vi"("reference"=w1187) -> ("element"=w1186:string)
            n728 = call "Dropdown Selection (SubVI).vi"("reference"=w1185) -> ("element"=w1175:string)
            n729 = case shown="False" w1178 {
              tunnel: [w1217 "0" ("element")] -> w1177
              tunnel: w1156 -> [w1217 _]
              frame False {
              }
              frame True {
              }
            }
            n730 = call "Prepare DB Connect Path (SubVI).vi"("connectString"=path "BIMS_Collector.udl", "error in"=w1159) -> ("appended path"=w1158:path, "error out"=w1160:errorcluster)  [unwired: 1 out]
            n731 = Format Into String(format string=", %d, '%s', '%s', '%s', '%s', %.4f, %.1f, '%s', %.4f, '%s', %d, '%s', %d, '%s', '%s', '%s', %.1f, %.1f, '%s', %.1f, '%s', '%s', '%s', %.1f, %.1f);" ("Format String"), initial string=w1213, error in=w1160, w1170, w1169, w1163, w1177, w1155, w1211, w1210, w1193, "Thickness", w1176, w1199, w1190, w1198, "Comments", w1188, w1173, "RoomT", "RoomHum", w1186, w1180, "ProjectID", "SampleID", w1175, "totalSampleWt", w1184) -> (resulting string=w1212:string, error out=w1162:errorcluster)
            n732 = call-poly <vilib>:"DB Tools Open Connection.vi"("error in (no error)"=w1162, "connection information"=w1158) -> ("error out"=w1171:errorcluster, "connection reference"=w1172:T33)  [unwired: 3 in, 3 out]
            n733 = Concatenate Strings(w1216, w1215, w1212) -> (w1205:string)
            n734 = call-poly <vilib>:"DB Tools Execute Query.vi"("error in (no error)"=w1171, "SQL query"=w1205, "connection reference"=w1172) -> ("error out"=w1204:errorcluster, "recordset reference"=w1202:T34)  [unwired: 1 in, 4 out]
            n735 = call-poly <vilib>:"DB Tools Free Object.vi"("error in (no error)"=w1204, "recordset reference"=w1202) -> ("error out"=w1203:errorcluster, "connection reference"=w1201:T33)  [unwired: 8 out]
          }
          frame #2 {
            # "Experiment.expt"
            n736 = local read "LastShot"() -> (w1228:i32)
            n737 = Increment(x=w1228) -> (x+1=w1226:i32)
            n738 = for {
              tunnel: w1221 -> [w1274] mode=indexing
              tunnel: w1230 -> [w1249]
              tunnel: w1229 -> [w1233]
              tunnel: [w1247] -> w1223
              tunnel: [w1248] -> w1225
              tunnel: w1226 -> [w1254]
              tunnel: [w1246] -> w1227
              tunnel: w1222 -> [w1242]
              i -> [w1246]
              w1234 = sgl 1.0 ("f")
              # "Shot.id"
              n739 = Add(x=w1254, y=w1246) -> (x+y=w1253:i32)
              n740 = Unbundle By Name(w1274) -> ("IMPACT VELOCITY"=w1260:sgl, "Redundant_Velocity"=w1239:sgl, "RESIDUAL  VELOCITY"=w1238:sgl, "Shot Description"=w1240:string, "Powder Loading"=w1264:sgl, "Barrel Temperature"=w1265:sgl, "TIME / DATE"=w1266:string, "shot order"=w1267:i32, "Shot Angle"=w1268:u16, "BackFace\nDepth"=w1269:sgl, "BackFace\nDiameter"=w1270:sgl, "SHOT STATUS"=w1272:u16, "Projectile Mass"=w1263:sgl, "usedv50"=w1262:bool, "Energy Loss (J)"=w1261:sgl, "avgVel_PB"=w1245:sgl, "velLoss_PB"=w1244:sgl, "strikeVel_PB"=w1243:sgl, "Frag Rod"=w1231:sgl)
              n741 = local read "Drag Corrected"() -> (w1236:bool)
              n742 = local read "Residual factor"() -> (w1258:sgl)
              n743 = local read "Impact factor"() -> (w1235:sgl)
              n744 = Greater Than 0?(x=w1272) -> (x > 0?=w1271:bool)
              n745 = Select(t=w1235, s=w1236, f=w1234) -> (s? t:f=w1256:sgl)
              n746 = Select(t=w1235, s=w1236, f=w1234) -> (s? t:f=w1241:sgl)
              n747 = Select(t=w1258, s=w1236, f=w1234) -> (s? t:f=w1257:sgl)
              n748 = Divide(x=w1260, y=w1256) -> (x/y=w1255:sgl)
              n749 = Divide(x=w1239, y=w1241) -> (x/y=w1237:sgl)
              n750 = Divide(x=w1238, y=w1257) -> (x/y=w1259:sgl)
              n751 = Format Into String(format string="INSERT INTO shots (impactdc, redundantdc, residualdc,  comment, loading, barreltemp, [date], [order], shotangle, bfdepth, bfdiameter, [complete], expt, id, weight,usedv50, loss, residual, impact, redundant, avgVel_PB, velLoss_PB, strikeVel_PB, fragRod)  VALUES (%.1f, %.1f, %.1f, '%s', %.4f, %.1f, #%s#, %d, %d, %.3f, %.3f, %d, %d, %d, %.4f, %d, %.4f, %.1f, %.1f, %.1f, %.1f, %.1f, %.1f, %.1f)" ("Substring"), error in=w1233, w1260, w1239, w1238, w1240, w1264, w1265, w1266, w1267, w1268, w1269, w1270, w1271, w1242, w1253, w1263, w1262, w1261, w1259, w1255, w1237, w1245, w1244, w1243, w1231) -> (resulting string=w1250:string, error out=w1232:errorcluster)  [unwired: 1 in]
              n752 = call-poly <vilib>:"DB Tools Execute Query.vi"("error in (no error)"=w1232, "SQL query"=w1250, "connection reference"=w1249) -> ("error out"=w1252:errorcluster, "recordset reference"=w1251:T34)  [unwired: 1 in, 4 out]
              n753 = call-poly <vilib>:"DB Tools Free Object.vi"("error in (no error)"=w1252, "recordset reference"=w1251) -> ("error out"=w1247:errorcluster, "connection reference"=w1248:T33)  [unwired: 8 out]
            }
            n754 = call <vilib>:"DB Tools Close Connection.vi"("error in (no error)"=w1223, "connection reference"=w1225) -> ("error out"=w1224:errorcluster)  [unwired: 5 out]
          }
        }
        n755 = local read "configPath"() -> (w1069:path)
        n756 = case shown="No Error" w1070 {
          selector: w1070 -> [w1286 w1313]
          tunnel: [-1 -1] -> w1072
          tunnel: [Collector_State."POLL" ("progState") Collector_State."POLL" ("progState")] -> w1073
          tunnel: w1071 -> [w1297 _]
          tunnel: w1069 -> [w1281 _]
          tunnel: [w1280 w1311] -> w1067
          tunnel: w1066 -> [w1278 w1310]
          tunnel: [w1276 w1310] -> w1065
          frame No Error {
            w1287 = "Data Base Parameters" ("section")
            n757 = local read "LastShot"() -> (w1298:i32)
            n758 = Array Size(array=w1278) -> (size(s)=w1277:i32)
            n759 = flat-sequence {
              tunnel: w1280 -> [_]
              tunnel: w1275 -> [w1308]
              tunnel: [w1308] -> w1276
              frame #0 {
                w1301 = T14."Disabled and Grayed Out" ("Disabled")
                n760 = property on="saveReq" class="Str"("Visible"=TRUE) -> ()  [unwired: 2 in, 2 out]
                n761 = local write "SampleID"("") -> ()
                n762 = property on="clearShots" class="Bool"("Disabled"=T14."Enabled") -> ()  [unwired: 2 in, 2 out]
                n763 = property on="addShot" class="Bool"("Disabled"=w1301) -> ()  [unwired: 2 in, 2 out]
                n764 = property on="undoLastShot" class="Bool"("Disabled"=w1301) -> ()  [unwired: 2 in, 2 out]
                n765 = property on="saveShots" class="Bool"("Disabled"=w1301) -> ()  [unwired: 2 in, 2 out]
                n766 = One Button Dialog(message="Data Saved. Enter new Sample ID.") -> ()  [unwired: 1 in, 1 out]
                n767 = property on="mainTabCntrl" class="TabCtl (strict)"("Value"=enum32{"Setup", "Measure", "History", "System"}."Setup" ("mainTabCntrl")) -> ()  [unwired: 2 in, 2 out]
                n768 = property on="SampleEntryTabCntrl" class="TabCtl (strict)"("Value"=enum32{"Environment", "Sample"}."Sample" ("SampleEntryTabCntrl")) -> ()  [unwired: 2 in, 2 out]
                n769 = property on="Sample SubTabCntrl" class="TabCtl (strict)"("Value"=T2."General Specification" ("Sample SubTabCntrl")) -> ()  [unwired: 2 in, 2 out]
              }
            }
            n770 = Increment(x=w1298) -> (x+1=w1292:i32)
            n771 = call <vilib>:"Open Config Data (compatibility).vi"("error in (no error)"=w1286, "configuration file path"=w1281) -> ("error out"=w1291:errorcluster, "refnum"=w1290:T35)  [unwired: 7 in, 1 out]
            n772 = Add(x=w1292, y=w1297) -> (x+y=w1293:i32)
            n773 = local read "LastSample"() -> (w1294:i32)
            n774 = for {
              N: w1277 -> [_]
              shift-right: [w1299] -> w1275
              shift-left: w1278 -> [w1300]
              n775 = Delete From Array(array=w1300) -> (array with subset deleted=w1299:T7[])  [unwired: 2 in, 1 out]
            }
            n776 = local write "LastShot"(w1293) -> ()
            n777 = call-poly <vilib>:"Write Key.vi"("section"=w1287, "error in (no error)"=w1291, "value"=w1293, "key"="Last Shot Saved ", "refnum"=w1290) -> ("error out"=w1289:errorcluster, "refnum out"=w1288:T35)  [unwired: 5 out]
            n778 = Increment(x=w1294) -> (x+1=w1282:i32)
            n779 = local write "LastSample"(w1282) -> ()
            n780 = call-poly <vilib>:"Write Key.vi"("section"=w1287, "error in (no error)"=w1289, "value"=w1282, "key"="Last Panel Saved ", "refnum"=w1288) -> ("error out"=w1279:errorcluster)  [unwired: 6 out]
            n781 = To Double Precision Float(number=w1282) -> (double precision float=w1285:dbl)
            n782 = call <vilib>:"Close Config Data.vi"("error in (no error)"=w1279, "refnum"=w1288) -> ("error out"=w1280:errorcluster)  [unwired: 1 in, 8 out]
            n783 = property on="Record #" class="DigNum (strict)"("Maximum"=w1285) -> ()  [unwired: 2 in, 2 out]
            n784 = property on="SHOTS" class="Arr (strict)"("Val(Sgnl)"=w1275) -> ()  [unwired: 2 in, 2 out]
          }
          frame Error {
            n785 = One Button Dialog(message="Error saving Data. ") -> ()  [unwired: 2 out]
            n786 = call <vilib>:"General Error Handler.vi"("error in (no error)"=w1313) -> ("error out"=w1311:errorcluster)  [unwired: 2 in, 12 out]
          }
        }
      }
      frame 5 {
        # "Shot Order"
        # "This section accepts new data to the shot table."
        n787 = property on="undoLastShot" class="Bool"(error in=w1323, "Disabled"=u8 0) -> (error out=w1322:errorcluster)  [unwired: 1 in, 1 out]
        n788 = local read "residual/speed"() -> (w1349:sgl)
        n789 = local read "Impact/speed"() -> (w1353:sgl)
        n790 = Array Size(array=w1329) -> (size(s)=w1334:i32)
        n791 = Increment(x=w1334) -> (x+1=w1354:i32)
        n792 = case shown="\"grains\"" "loadingUnits" {
          tunnel: [w1361 w1362] -> w1318
          tunnel: "Powder Loading" -> [w1361 w1363]
          frame "grams", Default {
            # "Always save in grams."
          }
          frame "grains" {
            # "Always save in grams."
            n793 = Multiply(x=w1363, y=sgl 0.06479891) -> (x*y=w1362:sgl)
          }
        }
        n794 = local read "Current/residual/speed"() -> (w1337:sgl)
        n795 = local read "CorrectedVelScrnSet2"() -> (w1358:sgl)
        n796 = local read "MeasVelScrnSet2"() -> (w1355:sgl)
        n797 = local read "CorrectedVelScrnSet1"() -> (w1338:sgl)
        n798 = local read "MeasVelScrnSet1"() -> (w1356:sgl)
        n799 = local read "Current/avg/speed"() -> (w1360:sgl)
        n800 = local read "Corrected Residual"() -> (w1336:sgl)
        n801 = local read "BACKFACE DEPTH"() -> (w1340:sgl)
        n802 = local read "Redundant/speed"() -> (w1357:sgl)
        n803 = local read "conversion factor"() -> (w1347:sgl)
        n804 = local read "Projectile Mass"() -> (w1326:sgl)
        n805 = local read "SHOT STATUS"() -> (w1333:u16)
        n806 = local read "Avg/speed"() -> (w1359:sgl)
        n807 = Multiply(x=w1353, y=w1347) -> (x*y=w1345:sgl)
        n808 = Multiply(x=w1347, y=w1349) -> (x*y=w1346:sgl)
        n809 = Multiply(x=w1345, y=w1345) -> (x*y=w1341:sgl)
        n810 = Multiply(x=w1346, y=w1346) -> (x*y=w1342:sgl)
        n811 = Subtract(x=w1341, y=w1342) -> (x-y=w1343:sgl)
        n812 = Format Date/Time String(time format string (%c)="%x   %H:%M:%S") -> (date/time string=w1350:string)  [unwired: 2 out]
        "SUBMIT DATE/TIME" <- w1350
        n813 = Compound Arithmetic op=MULTIPLY(w1326, w1343, sgl 0.0005 ("Input")) -> (w1348:sgl)
        n814 = Index Array(array=w1329) -> (element=w1332:T7)  [unwired: 1 in]
        n815 = Bundle By Name(cluster=w1332, "TIME / DATE"=w1350, "shot order"=w1354, "IMPACT VELOCITY"=w1353, "RESIDUAL  VELOCITY"=w1349, "Shot Description"="Shot Description", "Powder Loading"=w1318, "Barrel Temperature"="Barrel Temp", "SHOT STATUS"=w1333, "BackFace\nDepth"=w1340, "Shot Angle"="Shot Angle", "Uncorrected Impact"=w1356, "Corrected Impact"=w1338, "Uncorrected Residual"=w1337, "Corrected residual"=w1336, "Projectile Mass"=w1326, "Energy Loss (J)"=w1348, "UncorrectedRed_PB"=w1355, "Redundant_Velocity"=w1357, "CorrectedRed_PB"=w1358, "UncorrectedAvgVel_PB"=w1360, "avgVel_PB"=w1359, "Frag Rod"="Frag Rod", "V50userExcl"=FALSE) -> (w1335:T7)
        n816 = Build Array (concatenate)(w1329, w1335) -> (w1325:T7[])
        n817 = stacked-sequence {
          tunnel: w1325 -> [w1368]
          tunnel: [w1368] -> w1324
          tunnel: w1322 -> [w1367]
          tunnel: [w1366] -> w1321
          frame #0 {
            n818 = property on="shotsTabCntrl" class="TabCtl (strict)"(error in=w1367, "Value"=T5."Shots Table" ("shotsTabCntrl")) -> (error out=w1366:errorcluster)  [unwired: 1 in, 1 out]
            n819 = local write "backdepth"(sgl 0.0 ("BACKFACE DEPTH")) -> ()
          }
        }
      }
      frame 6 {
        # "This section will clear the shot table and re-enable the \"ADD SHOT\" button to get ready for a new test panel."
        n820 = Two Button Dialog(message="Shot table cleared even if not saved. Are you sure?", 1:"NO" ("F button name (\"Cancel\")"), 2:"YES" ("T button name (\"OK\")")) -> (T button?=w1373:bool)
        n821 = case shown="True" w1373 {
          tunnel: [w1379 T7[] [] ("SHOTS")] -> w1378
          tunnel: w1374 -> [w1379 _]
          frame False {
          }
          frame True {
            w1380 = T14."Disabled and Grayed Out" ("Disabled")
            n822 = invoke on="Table of Shots" class="Tbl (strict)" method="Reinit To Default"() -> ()  [unwired: 3 in, 3 out]
            n823 = invoke on="SHOTS" class="Arr (strict)" method="Reinit To Default"() -> ()  [unwired: 3 in, 3 out]
            n824 = property on="addShot" class="Bool"("Disabled"=T14."Enabled") -> ()  [unwired: 2 in, 2 out]
            n825 = property on="clearShots" class="Bool"("Disabled"=w1380) -> ()  [unwired: 2 in, 2 out]
            n826 = property on="undoLastShot" class="Bool"("Disabled"=w1380) -> ()  [unwired: 2 in, 2 out]
            n827 = property on="saveShots" class="Bool"("Disabled"=w1380) -> ()  [unwired: 2 in, 2 out]
            n828 = property on="saveReq" class="Str"("Visible"=TRUE) -> ()  [unwired: 2 in, 2 out]
          }
        }
      }
      frame 7 {
        n829 = property on="SHOTS" class="Arr (strict)"(error in=w1386) -> (error out=w1385:errorcluster, "Index Values"=w1390:u32[])  [unwired: 1 in, 1 out]
        n830 = Array Size(array=w1397) -> (size(s)=w1393:i32)
        n831 = Index Array "Index Array"(array=w1390) -> (element=w1395:u32)  [unwired: 1 in]
        n832 = To Unsigned Long Integer(number=w1393) -> (unsigned 32bit integer=w1389:u32)
        n833 = Increment(x=w1395) -> (x+1=w1394:u32)
        n834 = Quotient & Remainder(x=w1394, y=w1389) -> (x-y*floor(x/y)=w1392:u32)  [unwired: 1 out]
        n835 = Replace Array Subset "Replace Array Subset"(array=w1390, new element=w1392) -> (w1391:u32[])  [unwired: 1 in]
        n836 = property on="SHOTS" class="Arr (strict)"(error in=w1385, "Index Values"=w1391) -> (error out=w1384:errorcluster, "Value"=w1396:T7[])  [unwired: 1 in, 1 out]
      }
      frame 8 {
        # "This section undoes new shot data OR deletes the currently accessed previous shot"
        n837 = local read "deleteShot"() -> (w1404:bool)
        n838 = case shown="True" w1404 {
          tunnel: w1403 -> [w1407 w1420]
          tunnel: [w1408 w1421] -> w1402
          frame False {
            n839 = Array Size(array=w1407) -> (size(s)=w1405:i32)
            n840 = while {
              tunnel: [w1411] -> w1406
              tunnel: w1405 -> [w1413]
              tunnel: w1407 -> [w1415] mode=indexing
              i -> [w1411]
              stop <- w1414 stop-if-true
              n841 = Unbundle By Name(w1415) -> ("shot order"=w1412:i32)
              n842 = Equal?(x=w1412, y=w1413) -> (x = y?=w1414:bool)
            }
            n843 = Delete From Array "Delete From Array"(array=w1407, index=w1406) -> (array with subset deleted=w1408:T7[])  [unwired: 1 in, 1 out]
            n844 = local write "SUBMIT DATE/TIME"("" ("Empty String Constant")) -> ()
            n845 = property on="undoLastShot" class="Bool"("Disabled"=u8 2) -> ()  [unwired: 2 in, 2 out]
          }
          frame True {
            n846 = property on="SHOTS" class="Arr (strict)"() -> ("Index Values"=w1429:u32[])  [unwired: 2 in, 2 out]
            n847 = local write "deleteShot"(FALSE) -> ()
            n848 = Index Array(array=w1429, index=0 ("Index")) -> (element=w1419:u32)
            n849 = To Long Integer(number=w1419) -> (32bit integer=w1416:i32)
            n850 = Index Array(array=w1420, index=w1416) -> (element=w1418:T7)
            n851 = Unbundle By Name(w1418) -> ("shot order"=w1417:i32)
            n852 = Format Into String(format string="The currently displayed Shot, #%d", w1417) -> (resulting string=w1426:string)  [unwired: 2 in, 1 out]
            n853 = Concatenate Strings(w1426, ", will be deleted.  IT CANNOT RECOVERED!  Do you want to DELETE the shot?" ("message")) -> (w1425:string)
            n854 = Two Button Dialog(message=w1425, 1:"NO I do NOT want to delete.  Cancel Request" ("F button name (\"Cancel\")"), 2:"YES I want to delete the shot" ("T button name (\"OK\")")) -> (T button?=w1432:bool)
            n855 = case shown="True" w1432 {
              tunnel: w1420 -> [w1445 w1448]
              tunnel: [w1445 w1450] -> w1423
              tunnel: w1416 -> [_ w1447]
              tunnel: [10000 ("shot order") w1449] -> w1422
              frame False {
              }
              frame True {
                n856 = Index Array(array=w1448, index=w1447) -> (element=w1446:T7)
                n857 = Unbundle By Name(w1446) -> ("shot order"=w1449:i32)
                n858 = Delete From Array(array=w1448, index=w1447) -> (array with subset deleted=w1450:T7[])  [unwired: 1 in, 1 out]
              }
            }
            n859 = for {
              tunnel: [w1439] -> w1421 mode=indexing
              tunnel: w1423 -> [w1434] mode=indexing
              tunnel: w1422 -> [w1438]
              n860 = Unbundle By Name(w1434) -> ("shot order"=w1436:i32)
              n861 = Decrement(x=w1436) -> (x-1=w1435:i32)
              n862 = Greater?(x=w1436, y=w1438) -> (0:w1437:bool)
              n863 = case shown="True" w1437 {
                tunnel: w1435 -> [_ w1442]
                tunnel: w1434 -> [w1440 w1443]
                tunnel: [w1440 w1441] -> w1439
                frame False {
                }
                frame True {
                  n864 = Bundle By Name(cluster=w1443, "shot order"=w1442) -> (w1441:T7)
                }
              }
            }
          }
        }
        n865 = property on="SHOTS" class="Arr (strict)"(error in=w1398, "Val(Sgnl)"=w1402) -> (error out=w1399:errorcluster)  [unwired: 1 in, 1 out]
      }
      frame 9 {
        n866 = local write "SUBMIT DATE/TIME"("" ("Empty String Constant")) -> ()
        n867 = Concatenate Strings("L|", "6|") -> (w1457:string)
        n868 = case shown="\"Simulated\", Default" "MeasSrc" {
          tunnel: w1457 -> [_ _ w1473]
          tunnel: w1452 -> [w1463 w1468 w1472]
          tunnel: [w1461 w1468 w1469] -> w1451
          frame "Simulated", Default {
            n869 = flat-sequence {
              tunnel: w1463 -> [w1464]
              tunnel: [w1464] -> w1462
              tunnel: [w1466] -> w1461
              tunnel: w1462 -> [w1466]
              frame #0 {
                n870 = local write "readyClock"(FALSE ("RANGE RESET")) -> ()
              }
              frame #1 {
                n871 = Wait (ms)(milliseconds to wait=u32 100) -> ()  [unwired: 1 out]
              }
            }
          }
          frame "Radar" {
          }
          frame "Screens" {
            w1479 = u32 22 items=["NI-DAQ version", "device name", "base address", "data transfer mode for analog input", "data transfer mode for analog output group 1", "data transfer mode for analog output group 2", "data transfer mode for GPCTR 0", "data transfer mode for GPCTR 1", "data transfer mode for digital I/O group 1", "data transfer mode for digital I/O group 2", "device type code", "DMA A level", "DMA B level", "DMA C level", "interrupt A level", "interrupt B level", "reserved", "lpt device mode", "DAQCard-700 counter 1 source", "interrupt generation mode", "device state during suspend mode", "computer name", "serial number", "counter type", "Scarab A Memory Size", "Scarab B Memory Size"] ("information type")
            w1478 = u32 1  # device
            n872 = Concatenate Strings(w1473, "2|") -> (w1474:string)
            n873 = call <vilib>:"Get DAQ Device Information.vi"("error in (no error)"=w1472, "information type"=w1479, "task ID or device"=w1478) -> ("error out"=w1471:errorcluster, "information string"=w1477:string)  [unwired: 7 out]
            n874 = disable-structure "Diagram Disable Structure" shown="Enabled" {
              disable-tunnel: w1474 -> [w1484 _]
              disable-tunnel: w1471 -> [w1481 w1486]
              disable-tunnel: [w1480 w1486] -> w1470
              frame Disabled {
                n875 = Current VI's Path() -> (path=w1485:path)
                n876 = call "Where Am I (SubVI).vi"("TL Calling Location"=w1484, "Call VI path"=w1485) -> ("I'm here"=w1483:string)
                n877 = call "Error Check (SubVI).vi"("calling VI"=w1483, "tag #"=0, "error IN"=w1481) -> ("error OUT"=w1480:errorcluster)  [unwired: 2 in]
              }
              frame Enabled {
                # "Debug code is disabled"
              }
            }
            n878 = case shown="Error" w1470 {
              selector: w1470 -> [w1487 _]
              tunnel: w1477 -> [w1497 _]
              tunnel: [w1497 "DEVICE NOT READY!" ("information string")] -> w1476
              tunnel: [w1488 errorcluster {"status"=FALSE, "code"=0, "source"=""} ("error out")] -> w1469
              frame No Error {
                # "assign task IDs to counters"
                n879 = call "Config Counter to Measure Two Edge Separation.vi"("error IN"=w1487, "Counter"="Impact Timer", "device"="DAQ Card") -> ("error out"=w1499:errorcluster, "task ID out"=w1493:u32)  [unwired: 1 in]
                "impact/ID" <- w1493
                n880 = local write "readyClock"(FALSE ("RANGE RESET")) -> ()
                n881 = call "Config Counter to Measure Two Edge Separation.vi"("error IN"=w1499, "Counter"="Residual  Timer", "device"="DAQ Card") -> ("error out"=w1501:errorcluster, "task ID out"=w1491:u32)  [unwired: 1 in]
                "residual/ID" <- w1491
                n882 = call "Config Counter to Measure Two Edge Separation.vi"("error IN"=w1501, "Counter"="Redundant Timer", "device"="DAQ Card") -> ("error out"=w1500:errorcluster, "task ID out"=w1492:u32)  [unwired: 1 in]
                "Red/ID" <- w1492
                n883 = Bundle("task ID out"=w1493, "task ID out"=w1492, "task ID out"=w1491) -> (w1489:T36)  [unwired: 1 out]
                n884 = call <vilib>:"Simple Error Handler.vi"("error in (no error)"=w1500) -> ("error out"=w1488:errorcluster)  [unwired: 1 in, 7 out]
                n885 = global write "BIMS_Collector Globals.vi" "Screens"(w1489) -> ()
              }
              frame Error {
                n886 = One Button Dialog(message="Error initializing Timer board.  Switching to simulation") -> ()  [unwired: 2 out]
                n887 = local write "MeasSrc"(DataSource."Simulated" ("MeasSrc")) -> ()
              }
            }
            "Device S/N" <- w1476
          }
        }
      }
      frame 9 {
        n888 = local write "processShots"(FALSE ("ProcessShots")) -> ()
        n889 = local read "Drag Corrected"() -> (w1511:bool)
        n890 = stacked-sequence {
          seq-local: [_ w1569 _ _] -> [_ _ w1598 w1648]
          seq-local: [w1533 _ _ _] -> [_ w1565 _ _]
          seq-local: [w1531 _ _ _] -> [_ w1566 _ _]
          seq-local: [w1532 _ _ _] -> [_ w1567 _ _]
          tunnel: [_ _ _ w1642] -> w1512
          tunnel: w1511 -> [w1535 w1568 _ _]
          tunnel: w1508 -> [_ w1564 _ _]
          tunnel: w1507 -> [w1530 _ _ _]
          tunnel: [w1530 _ _ _] -> w1506
          frame #0 {
            n891 = disable-structure "Diagram Disable Structure" shown="Enabled" {
              disable-tunnel: [w1552 w1559] -> w1540
              frame Disabled {
                n892 = local read "factor array"() -> (w1554:sgl[])
                n893 = local read "Threat"() -> (w1551:u16)
                n894 = To Long Integer(number=w1551) -> (32bit integer=w1553:i32)
                n895 = Index Array(array=w1554, index=w1553) -> (element=w1552:sgl)
              }
              frame Enabled {
                n896 = local read "threatDetails"() -> (w1558:T1)
                n897 = Unbundle By Name(w1558) -> ("dragCorrection"=w1556:string)
                n898 = Not Equal?(x=w1556, y="") -> (x != y?=w1557:bool)
                n899 = case shown="True" w1557 {
                  tunnel: [sgl 1.0 ("default value 1") w1562] -> w1559
                  tunnel: w1556 -> [_ w1561]
                  frame False {
                  }
                  frame True {
                    n900 = Scan From String(input string=w1561, default 1=sgl 0.0 ("default value 1")) -> (output 1=w1562:sgl)  [unwired: 3 in, 3 out]
                  }
                }
              }
            }
            "correction coefficient" <- w1540
            n901 = local read "Current/avg/speed"() -> (w1536:sgl)
            n902 = local read "mid_to_targ_dist"() -> (w1537:sgl)
            n903 = local read "lengthUnits"() -> (w1534:string)
            n904 = call "Compute Strike Velocity.vi"("drag coefficient"=w1540, "decay distance"=w1537, "raw velocity"=w1536, "distance units"=w1534) -> ("correction factor"=w1533:sgl, "strike velocity"=w1538:sgl)  [unwired: 1 out]
            "DC_ factor" <- w1533
            "Corrected Average" <- w1538
            n905 = call "Velocity Correction.vi"("raw impact"="MeasVelScrnSet1", "distance units"=w1534, "raw redundant"="MeasVelScrnSet2", "raw residual"="Current/residual/speed", "screen set midpt to target"="Set#1_to_Target", "residual screen to target"="Residual/Target Dist", "correction coefficient"=w1540) -> ("corrected impact"=w1545:sgl, "corrected redundant"=w1541:sgl, "corrected residual"=w1543:sgl, "impact factor"=w1531:sgl, "conversion factor"=→"conversion factor":sgl, "residual factor"=w1532:sgl)  [unwired: 3 out]
            "Residual factor" <- w1532
            "Impact factor" <- w1531
            "CorrectedVelScrnSet1" <- w1545
            "Corrected Residual" <- w1543
            "CorrectedVelScrnSet2" <- w1541
            n906 = Select(t=w1541, s=w1535, f="MeasVelScrnSet2") -> (s? t:f=→"Redundant/speed":sgl)
            n907 = Select(t=w1538, s=w1535, f=w1536) -> (s? t:f=→"Avg/speed":sgl)
            n908 = Select(t=w1545, s=w1535, f="MeasVelScrnSet1") -> (s? t:f=→"Impact/speed":sgl)
            n909 = Select(t=w1543, s=w1535, f="Current/residual/speed") -> (s? t:f=→"residual/speed":sgl)
            n910 = Add(x="MeasVelScrnSet2", y="MeasVelScrnSet1") -> (x+y=w1517:sgl)
            n911 = Subtract(x="MeasVelScrnSet2", y="MeasVelScrnSet1") -> (x-y=w1516:sgl)
            n912 = Divide(x=w1517, y=sgl 200.0) -> (x/y=w1518:sgl)
            n913 = Divide(x=w1516, y=w1518) -> (x/y=w1522:sgl)
            "%_Difference" <- w1522
            n914 = Absolute Value(x=w1522) -> (abs(x)=w1524:sgl)
            n915 = Less?(x=w1524, y="percent warning") -> (x < y?=w1529:bool)
            n916 = Select(t=u32 65343, s=w1529, f=u32 15668992) -> (s? t:f=w1525:u32)
            n917 = Select(t=u32 0, s=w1529, f=u32 16777226) -> (s? t:f=w1528:u32)
            n918 = property on="%_Difference" class="DigNum (strict)"("Numeric Text.Text Colors:BG Color"=w1525, "NumText.TextColor"=w1528) -> ()  [unwired: 2 in, 2 out]
          }
          frame #1 {
            # "<-- DC_factor (for Average of impact and redundant)"
            # "IF drag corrected THEN apply factors"
            # "Residual factor"
            # "Impact factor\n(also applies to\nredundant velocity)"
            n919 = for {
              tunnel: w1564 -> [w1577] mode=indexing
              tunnel: w1567 -> [w1586]
              tunnel: w1566 -> [w1581]
              tunnel: w1568 -> [w1575]
              tunnel: [w1588] -> w1569 mode=indexing
              tunnel: w1565 -> [w1570]
              n920 = Unbundle By Name(w1577) -> ("UncorrectedAvgVel_PB"=w1576:sgl)
              n921 = Unbundle By Name(w1577) -> ("Uncorrected Impact"=w1580:sgl)
              n922 = Unbundle By Name(w1577) -> ("Uncorrected Residual"=w1585:sgl)
              n923 = Unbundle By Name(w1577) -> ("UncorrectedRed_PB"=w1583:sgl)
              n924 = Multiply(x=w1570, y=w1576) -> (x*y=w1573:sgl)
              n925 = Multiply(x=w1581, y=w1583) -> (x*y=w1582:sgl)
              n926 = Multiply(x=w1581, y=w1580) -> (x*y=w1571:sgl)
              n927 = Multiply(x=w1586, y=w1585) -> (x*y=w1578:sgl)
              n928 = Select(t=w1573, s=w1575, f=w1576) -> (s? t:f=w1574:sgl)
              n929 = Select(t=w1582, s=w1575, f=w1583) -> (s? t:f=w1584:sgl)
              n930 = Select(t=w1578, s=w1575, f=w1585) -> (s? t:f=w1587:sgl)
              n931 = Select(t=w1571, s=w1575, f=w1580) -> (s? t:f=w1579:sgl)
              n932 = Subtract(x=w1574, y=w1573) -> (x-y=w1572:sgl)
              n933 = Bundle By Name(cluster=w1577, "velLoss_PB"=w1572, "strikeVel_PB"=w1573, "avgVel_PB"=w1574, "CorrectedRed_PB"=w1582, "Redundant_Velocity"=w1584, "Corrected Impact"=w1571, "IMPACT VELOCITY"=w1579, "Corrected residual"=w1578, "RESIDUAL  VELOCITY"=w1587) -> (w1588:T7)
            }
          }
          frame #2 {
            w1599 = sgl[] [] ("Partial")
            # "This section calculates the V50"
            n934 = for {
              shift-right: [w1623] -> w1601
              shift-left: w1599 -> [w1624]
              shift-right: [w1621] -> w1600
              shift-left: w1599 -> [w1622]
              tunnel: w1598 -> [w1615] mode=indexing
              n935 = Unbundle By Name(w1615) -> ("SHOT STATUS"=w1620:u16)
              n936 = Unbundle By Name(w1615) -> ("V50userExcl"=w1614:bool)
              n937 = Unbundle By Name(w1615) -> ("IMPACT VELOCITY"=w1619:sgl)
              n938 = Unbundle By Name(w1615) -> ("strikeVel_PB"=w1618:sgl)
              n939 = Select(t=w1618, s="ScreenSetAvgg", f=w1619) -> (s? t:f=w1617:sgl)
              n940 = case shown="False" w1614 {
                tunnel: w1624 -> [w1630 w1640]
                tunnel: [w1629 w1640] -> w1623
                tunnel: w1622 -> [w1628 w1639]
                tunnel: [w1627 w1639] -> w1621
                tunnel: w1620 -> [w1626 _]
                tunnel: w1617 -> [w1625 _]
                frame False {
                  n941 = case shown="1" w1626 {
                    tunnel: w1625 -> [w1631 w1635]
                    tunnel: [w1634 w1636] -> w1629
                    tunnel: w1630 -> [w1633 w1636]
                    tunnel: w1628 -> [w1632 w1638]
                    tunnel: [w1632 w1637] -> w1627
                    frame 0, Default {
                      n942 = Build Array (concatenate)(w1633, w1631) -> (w1634:sgl[])
                    }
                    frame 1 {
                      n943 = Build Array (concatenate)(w1638, w1635) -> (w1637:sgl[])
                    }
                  }
                }
                frame True {
                }
              }
            }
            n944 = Sort 1D Array(array=w1601) -> (sorted array=w1613:sgl[])
            n945 = Sort 1D Array(array=w1600) -> (sorted array=w1606:sgl[])
            "Complete" <- w1606
            n946 = Reverse 1D Array(array=w1613) -> (reversed array=w1604:sgl[])
            "Partial" <- w1604
            n947 = Array Size(array=w1606) -> (size(s)=→"#_completes":i32)
            n948 = Array Size(array=w1604) -> (size(s)=→"#_partials":i32)
            n949 = Array Max & Min(array=w1604) -> (max value=w1610:sgl)  [unwired: 3 out]
            n950 = Array Max & Min(array=w1606) -> (min value=w1608:sgl)  [unwired: 3 out]
            n951 = call "Compute V50.vi"("Partial"=w1604, "Maximum Deviation"="maxDev", "Complete"=w1606) -> ("Pairs"=→"Pairs":i16, "zmr"=w1589:sgl, "V50"=→"computed_V50":sgl)  [unwired: 2 out]
            "Z.M.R." <- w1589
            n952 = To Long Integer(number=w1610) -> (32bit integer=→"highPartial":i32)
            n953 = To Long Integer(number=w1608) -> (32bit integer=→"lowComplete":i32)
            n954 = Absolute Value(x=w1589) -> (abs(x)=→"zmr 2":sgl)
            n955 = Less Than 0?(x=w1589) -> (x < 0?=w1592:bool)
            n956 = Select(t="Low C minus High P", s=w1592, f="ZMR") -> (s? t:f=w1595:string)
            n957 = Select(t=u32 65336, s=w1592, f=u32 16755266) -> (s? t:f=w1596:u32)
            n958 = property on="zmr 2" class="DigNum (strict)"("Caption.Text"=w1595, "Numeric Text.Text Colors:BG Color"=w1596) -> ()  [unwired: 2 in, 2 out]
          }
          frame #3 {
            n959 = local read "Pairs"() -> (w1653:i16)
            n960 = Sort 1D Array(array=w1648) -> (sorted array=w1651:T7[])
            n961 = for {
              tunnel: w1651 -> [w1697] mode=indexing
              tunnel: w1653 -> [w1707]
              shift-right: [w1706] -> _
              shift-left: i16 0 -> [w1705]
              tunnel: [w1699] -> w1649 mode=indexing
              # "this section marks the lowest completes that are used in V50"
              n962 = Unbundle By Name(w1697) -> ("SHOT STATUS"=w1703:u16, "Projectile Mass"=w1701:sgl, "avgVel_PB"=w1700:sgl, "RESIDUAL  VELOCITY"=w1702:sgl)
              n963 = Unbundle By Name(w1697) -> ("V50userExcl"=w1698:bool)
              n964 = local read "conversion factor"() -> (w1709:sgl)
              n965 = case shown="False" w1698 {
                tunnel: w1707 -> [w1720 _]
                tunnel: [w1719 w1729] -> w1706
                tunnel: w1705 -> [w1718 w1729]
                tunnel: [w1717 FALSE] -> w1704
                tunnel: w1703 -> [w1716 _]
                frame False {
                  n966 = case shown="1" w1716 {
                    tunnel: w1720 -> [_ w1727]
                    tunnel: [FALSE w1726] -> w1717
                    tunnel: [w1722 w1725] -> w1719
                    tunnel: w1718 -> [w1722 w1723]
                    frame 0, Default {
                    }
                    frame 1 {
                      n967 = Less?(x=w1723, y=w1727) -> (x < y?=w1726:bool)
                      n968 = Add(x=w1723, y=i16 1 ("t")) -> (x+y=w1725:i16)
                    }
                  }
                }
                frame True {
                }
              }
              n969 = Multiply(x=w1709, y=w1702) -> (x*y=w1710:sgl)
              n970 = Multiply(x=w1700, y=w1709) -> (x*y=w1711:sgl)
              n971 = Multiply(x=w1711, y=w1711) -> (x*y=w1715:sgl)
              n972 = Multiply(x=w1710, y=w1710) -> (x*y=w1714:sgl)
              n973 = Subtract(x=w1715, y=w1714) -> (x-y=w1713:sgl)
              n974 = Compound Arithmetic op=MULTIPLY(w1701, w1713, sgl 0.0005 ("Input")) -> (w1708:sgl)
              n975 = Bundle By Name(cluster=w1697, "usedv50"=w1704, "Energy Loss (J)"=w1708) -> (w1699:T7)
            }
            n976 = Reverse 1D Array(array=w1649) -> (reversed array=w1650:T7[])
            n977 = for {
              tunnel: w1650 -> [w1673] mode=indexing
              tunnel: w1653 -> [w1680]
              shift-right: [w1678] -> _
              shift-left: i16 0 -> [w1679]
              tunnel: [w1676] -> w1642 mode=indexing
              # "chooses highest partials used in v50"
              n978 = Unbundle By Name(w1673) -> ("SHOT STATUS"=w1681:u16, "usedv50"=w1675:bool)
              n979 = Unbundle By Name(w1673) -> ("V50userExcl"=w1674:bool)
              n980 = case shown="True" w1674 {
                tunnel: w1681 -> [w1687 _]
                tunnel: w1680 -> [w1686 _]
                tunnel: w1679 -> [w1685 w1696]
                tunnel: [w1684 w1696] -> w1678
                tunnel: [w1683 FALSE ("usedv50")] -> w1677
                tunnel: w1675 -> [w1682 _]
                frame False {
                  n981 = case shown="1" w1687 {
                    tunnel: w1686 -> [w1691 _]
                    tunnel: [w1690 w1694] -> w1683
                    tunnel: w1685 -> [w1688 w1693]
                    tunnel: [w1689 w1693] -> w1684
                    tunnel: w1682 -> [_ w1694]
                    frame 0, Default {
                      n982 = Less?(x=w1688, y=w1691) -> (x < y?=w1690:bool)
                      n983 = Add(x=w1688, y=i16 1) -> (x+y=w1689:i16)
                    }
                    frame 1 {
                    }
                  }
                }
                frame True {
                }
              }
              n984 = Bundle By Name(cluster=w1673, "usedv50"=w1677) -> (w1676:T7)
            }
            n985 = for {
              shift-right: [w1659] -> w1641
              shift-left: sgl[] [] ("Partial") -> [w1656]
              tunnel: w1642 -> [w1658] mode=indexing
              n986 = local read "ScreenSetAvgg"() -> (w1663:bool)
              n987 = Unbundle By Name(w1658) -> ("IMPACT VELOCITY"=w1661:sgl)
              n988 = Unbundle By Name(w1658) -> ("V50userExcl"=w1657:bool, "usedv50"=w1655:bool)
              n989 = Unbundle By Name(w1658) -> ("strikeVel_PB"=w1662:sgl)
              n990 = Select(t=w1662, s=w1663, f=w1661) -> (s? t:f=w1660:sgl)
              n991 = case shown="False" w1657 {
                tunnel: w1660 -> [w1664 _]
                tunnel: [w1665 w1672] -> w1659
                tunnel: w1656 -> [w1666 w1672]
                tunnel: w1655 -> [w1667 _]
                frame False {
                  n992 = case shown="True" w1667 {
                    tunnel: w1666 -> [w1668 w1671]
                    tunnel: [w1668 w1670] -> w1665
                    tunnel: w1664 -> [_ w1669]
                    frame False {
                    }
                    frame True {
                      n993 = Build Array (concatenate)(w1671, w1669) -> (w1670:sgl[])
                    }
                  }
                }
                frame True {
                }
              }
            }
            n994 = Array Max & Min(array=w1641) -> (max value=w1647:sgl, min value=w1646:sgl)  [unwired: 2 out]
            n995 = property on="SHOTS" class="Arr (strict)"("Val(Sgnl)"=w1642) -> ()  [unwired: 2 in, 2 out]
            n996 = Subtract(x=w1647, y=w1646) -> (x-y=w1645:sgl)
            n997 = To Long Integer(number=w1645) -> (32bit integer=→"rangeOfResults":i32)
          }
        }
      }
      frame 11 {
        n998 = local read "SafetyInterlock"() -> (w1738:cluster{"ARMED":bool})
        n999 = Unbundle By Name(w1738) -> ("ARMED"=w1737:bool)
        n1000 = Not(x="InterlockExists") -> (.not. x?=w1733:bool)
        n1001 = Or(x=w1737, y=w1733) -> (x .or. y?=w1734:bool)
        n1002 = case shown="True" w1734 {
          tunnel: [Collector_State."POLL" ("progState") w1747] -> w1736
          tunnel: [-1 ("index of element") w1746] -> w1735
          tunnel: "InterlockExists" -> [_ w1745]
          tunnel: [w1740 w1744] -> w1731
          tunnel: w1730 -> [w1740 w1743]
          frame False {
          }
          frame True {
            n1003 = stacked-sequence {
              tunnel: [_ Collector_State."PROCESS SHOTS" ("progState")] -> w1747
              tunnel: [_ -1] -> w1746
              tunnel: w1745 -> [w1750 _]
              tunnel: [w1748 _] -> w1744
              tunnel: w1743 -> [w1749 _]
              frame #0 {
                n1004 = local read "MeasSrc"() -> (w1752:T6)
                n1005 = case shown="\"Simulated\", Default" w1752 {
                  tunnel: [w1755 w1779 w1790] -> w1751
                  tunnel: w1750 -> [_ _ w1788]
                  tunnel: w1749 -> [w1753 w1778 w1786]
                  tunnel: [w1753 w1778 w1787] -> w1748
                  frame "Simulated", Default {
                    # "Simulated"
                    n1006 = local read "minV50"() -> (w1761:i32)
                    n1007 = local read "Powder Loading"() -> (w1777:sgl)
                    n1008 = To Single Precision Float(number=w1761) -> (single precision float=w1760:sgl)
                    n1009 = call "Get Shell Speed.vi"("loading"=w1777, "v50"=w1760) -> ("impact"=w1765:sgl, "residual"=w1772:sgl)  [unwired: 1 in, 2 out]
                    n1010 = Random Number (0-1)() -> (number: 0 to 1=w1770:dbl)
                    n1011 = To Single Precision Float(number=w1770) -> (single precision float=w1766:sgl)
                    n1012 = Multiply(x=w1766, y=sgl 0.002) -> (x*y=w1769:sgl)
                    n1013 = local read "SafetyInterlock"() -> (w1756:cluster{"ARMED":bool})
                    n1014 = Add(x=w1769, y=sgl 0.999) -> (x+y=w1767:sgl)
                    n1015 = Greater Than 0?(x=w1772) -> (x > 0?=w1774:bool)
                    n1016 = Multiply(x=w1765, y=w1767) -> (x*y=w1764:sgl)
                    n1017 = Bundle By Name(cluster=w1756, "ARMED"=FALSE) -> (w1757:cluster{"ARMED":bool})
                    n1018 = Add(x=w1765, y=w1764) -> (x+y=w1762:sgl)
                    n1019 = Select(t=u16 1, s=w1774, f=u16 0) -> (s? t:f=w1773:u16)
                    n1020 = local write "readyClock"(TRUE ("RANGE RESET")) -> ()
                    n1021 = local write "SafetyInterlock"(w1757) -> ()
                    n1022 = Divide(x=w1762, y=sgl 2.0 ("v50")) -> (x/y=w1755:sgl)
                    n1023 = local write "Current/residual/speed"(w1772) -> ()
                    n1024 = local write "SHOT STATUS"(w1773) -> ()
                    n1025 = local write "Current/sthotstatus"(w1773) -> ()
                    n1026 = local write "MeasVelScrnSet1"(w1765) -> ()
                    n1027 = local write "MeasVelScrnSet2"(w1764) -> ()
                    n1028 = Wait (ms)(milliseconds to wait=u32 500 ("number")) -> ()  [unwired: 1 out]
                  }
                  frame "Radar" {
                    # "Radar -- (future)"
                    n1029 = local read "MeasVelScrnSet1"() -> (w1781:sgl)
                    n1030 = local read "MeasVelScrnSet2"() -> (w1780:sgl)
                    n1031 = Add(x=w1781, y=w1780) -> (x+y=w1782:sgl)
                    n1032 = Divide(x=w1782, y=sgl 2.0) -> (x/y=w1779:sgl)
                  }
                  frame "Screens" {
                    # "This section checks to see if the counters have been fired.  If they have then the counter times are read"
                    n1033 = Concatenate Strings("-1|", "F0|") -> (w1791:string)
                    n1034 = case shown="True" w1788 {
                      tunnel: w1786 -> [w1798 w1799]
                      tunnel: [w1798 w1799] -> w1785
                      frame False {
                      }
                      frame True {
                      }
                    }
                    n1035 = global read "BIMS_Collector Globals.vi" "Screens"() -> (w1789)
                    n1036 = Unbundle By Name(w1789) -> ("ScrnSet1CntrID"=w1794)
                    n1037 = Concatenate Strings(w1791, "2|") -> (w1795:string)
                    n1038 = call "Check DAQ Status.vi"("errIN"=w1785, "TL Calling Location"=w1795, "Task ID"=w1794) -> ("error out"=w1797:errorcluster, "Armed?"=w1784:bool)  [unwired: 1 out]
                    n1039 = case shown="False" w1784 {
                      tunnel: w1797 -> [w1827 w1865]
                      tunnel: w1794 -> [w1810 _]
                      tunnel: w1795 -> [w1823 _]
                      tunnel: w1789 -> [w1813 _]
                      tunnel: [w1801 w1866] -> w1790
                      tunnel: [w1800 w1865] -> w1787
                      frame False {
                        n1040 = local read "Set#1 Separation"() -> (w1830:sgl)
                        n1041 = Concatenate Strings(w1823, "F|") -> (w1818:string)
                        n1042 = call "Read TIO Count.vi"("TL Calling Location"=w1818, "error In"=w1827, "task IN"=w1810) -> ("error out"=w1812:errorcluster, "time (secs)"=w1832:sgl)  [unwired: 1 in, 4 out]
                        n1043 = Divide(x=w1830, y=w1832) -> (x/y=w1806:sgl)
                        n1044 = call "Arm TIO Channel.vi"("error IN"=w1812, "task ID IN"=w1810) -> ("error out"=w1811:errorcluster)  [unwired: 1 in, 2 out]
                        n1045 = Unbundle By Name(w1813) -> ("ScrnSet2CntrID"=w1815)
                        n1046 = Concatenate Strings(w1818, "a|") -> (w1821:string)
                        n1047 = call "Check DAQ Status.vi"("errIN"=w1811, "TL Calling Location"=w1821, "Task ID"=w1815) -> ("error out"=w1826:errorcluster, "Armed?"=w1817:bool)  [unwired: 1 out]
                        n1048 = case shown="False" w1817 {
                          tunnel: [w1843 sgl 0.0] -> w1807
                          tunnel: w1826 -> [w1842 w1847]
                          tunnel: [w1837 w1847] -> w1828
                          tunnel: w1815 -> [w1836 _]
                          tunnel: w1818 -> [w1840 _]
                          frame False {
                            n1049 = local read "Set#2 Separation"() -> (w1844:sgl)
                            n1050 = Concatenate Strings(w1840, "Fa|") -> (w1839:string)
                            n1051 = call "Read TIO Count.vi"("TL Calling Location"=w1839, "error In"=w1842, "task IN"=w1836) -> ("error out"=w1838:errorcluster, "time (secs)"=w1845:sgl)  [unwired: 1 in, 4 out]
                            n1052 = Divide(x=w1844, y=w1845) -> (x/y=w1843:sgl)
                            n1053 = call "Arm TIO Channel.vi"("error IN"=w1838, "task ID IN"=w1836) -> ("error out"=w1837:errorcluster)  [unwired: 1 in, 2 out]
                          }
                          frame True {
                          }
                        }
                        n1054 = Unbundle By Name(w1813) -> ("residualCntrID"=w1814)
                        n1055 = Add(x=w1806, y=w1807) -> (x+y=w1808:sgl)
                        n1056 = Concatenate Strings(w1818, "b|") -> (w1819:string)
                        n1057 = call "Check DAQ Status.vi"("errIN"=w1828, "TL Calling Location"=w1819, "Task ID"=w1814) -> ("error out"=w1825:errorcluster, "Armed?"=w1816:bool)  [unwired: 1 out]
                        n1058 = Divide(x=w1808, y=sgl 2.0) -> (x/y=w1801:sgl)
                        n1059 = case shown="True" w1816 {
                          tunnel: w1825 -> [w1854 w1863]
                          tunnel: [w1859 w1864] -> w1831
                          tunnel: w1814 -> [w1849 _]
                          tunnel: [w1848 w1863] -> w1802
                          tunnel: [w1856 sgl 0.0] -> w1829
                          tunnel: w1818 -> [w1851 _]
                          frame False {
                            w1860 = u16 1 items=["Partial", "Complete"] ("SHOT STATUS")
                            w1861 = u16 0 items=["Partial", "Complete"] ("SHOT STATUS")
                            n1060 = local read "Residual/Separation"() -> (w1855:sgl)
                            n1061 = Concatenate Strings(w1851, "Fb|") -> (w1852:string)
                            n1062 = call "Read TIO Count.vi"("TL Calling Location"=w1852, "error In"=w1854, "task IN"=w1849) -> ("error out"=w1850:errorcluster, "timeout"=w1857:bool, "time (secs)"=w1858:sgl)  [unwired: 1 in, 3 out]
                            n1063 = Divide(x=w1855, y=w1858) -> (x/y=w1856:sgl)
                            n1064 = call "Arm TIO Channel.vi"("error IN"=w1850, "task ID IN"=w1849) -> ("error out"=w1848:errorcluster)  [unwired: 1 in, 2 out]
                            n1065 = Select(t=w1861, s=w1857, f=w1860) -> (s? t:f=w1859:u16)
                          }
                          frame True {
                            w1864 = u16 1 items=["Partial", "Complete"] ("SHOT STATUS")
                          }
                        }
                        n1066 = local write "Current/residual/speed"(w1829) -> ()
                        n1067 = local write "MeasVelScrnSet1"(w1806) -> ()
                        n1068 = local write "MeasVelScrnSet2"(w1807) -> ()
                        n1069 = local write "SHOT STATUS"(w1831) -> ()
                        n1070 = local write "Current/sthotstatus"(w1831) -> ()
                        n1071 = case shown="No Error" w1802 {
                          selector: w1802 -> [w1835 _]
                          frame No Error {
                            # "=false"
                            n1072 = Unbundle By Name(w1835) -> ("status"=w1834:bool)
                            n1073 = Not(x=w1834) -> (.not. x?=w1833:bool)
                            n1074 = local write "readyClock"(w1833) -> ()
                          }
                          frame Error {
                          }
                        }
                        n1075 = local read "SafetyInterlock"() -> (w1803:cluster{"ARMED":bool})
                        n1076 = Bundle By Name(cluster=w1803, "ARMED"=FALSE) -> (w1804:cluster{"ARMED":bool})
                        n1077 = local write "SafetyInterlock"(w1804) -> ()
                        n1078 = call <vilib>:"Simple Error Handler.vi"("error in (no error)"=w1802) -> ("error out"=w1800:errorcluster)  [unwired: 1 in, 7 out]
                      }
                      frame True {
                        # "Error -10600 occurrs in \"Read Count.vi\"\n\n  Possible reason(s): NI-DAQ LV: No setup operation has been performed for the specified resources. Or, some resources require a specific ordering of calls for proper setup.  \n\n  Solution: To avoid this error, you must call the Dig_Line_Config function to setup the direction for each digital line prior to calling the Dig_Grp_Config function."
                        n1079 = local read "MeasVelScrnSet1"() -> (w1868:sgl)
                        n1080 = local read "MeasVelScrnSet2"() -> (w1867:sgl)
                        n1081 = Add(x=w1868, y=w1867) -> (x+y=w1869:sgl)
                        n1082 = Divide(x=w1869, y=sgl 2.0) -> (x/y=w1866:sgl)
                      }
                    }
                  }
                }
                "Current/avg/speed" <- w1751
              }
              frame #1 {
              }
            }
          }
        }
      }
    }
    "SMErr" <- w13
  }
  n1083 = while "U/I Event Handler" {
    shift-right: [w1874] -> _
    shift-left: w7 -> [w1875]
    stop <- FALSE stop-if-true
    n1084 = event shown="[23] \"RefreshMetadata\": Value Change" {
      selector: _ -> [_ _ _ _ _ _ _ _ _ _ _ _ _ _ _ _ _ _ _ _ _ _ _ _ _ _]
      dyn-events: _ -> [_ _ _ _ _ _ _ _ _ _ _ _ _ _ _ _ _ _ _ _ _ _ _ _ _ _]
      timeout: 100 -> [_ _ _ _ _ _ _ _ _ _ _ _ _ _ _ _ _ _ _ _ _ _ _ _ _ _]
      tunnel: w1875 -> [w1879 _ w1896 w1906 w1915 w1925 w1962 w1981 w1989 w2015 w2054 w2097 w2133 w2138 w2176 w2213 w2217 w2227 w2255 w2262 w2288 w2307 w2310 w2338 w2370 _]
      tunnel: [w1879 w1883 w1896 w1903 w1914 w1924 w1961 w1980 w1987 w2024 w2053 w2094 w2133 w2138 w2176 w2213 w2216 w2223 w2255 w2259 w2285 w2307 w2310 w2340 w2370 w2378] -> w1874
      tunnel: [FALSE ("UpdateMetadata") "EXIT" "diagPageVisible" "runtimeMenusVisible" "ARM" "QueryLoad" FALSE ("UpdateMetadata") FALSE ("UpdateMetadata") FALSE ("UpdateMetadata") FALSE ("UpdateMetadata") FALSE ("UpdateMetadata") FALSE ("UpdateMetadata") FALSE ("UpdateMetadata") FALSE ("UpdateMetadata") FALSE ("UpdateMetadata") FALSE ("UpdateMetadata") FALSE ("UpdateMetadata") FALSE ("UpdateMetadata") "Drag Corrected" FALSE ("UpdateMetadata") "PublishNewRecords" FALSE ("UpdateMetadata") FALSE ("UpdateMetadata") "RefreshMetadata" FALSE ("UpdateMetadata") FALSE ("UpdateMetadata")] -> w1873
      event Timeout {
        n1085 = event-data() -> ()  [unwired: 2 out]
        n1086 = Get Date/Time In Seconds() -> (seconds since 1Jan1904=w1881:timestamp)
        n1087 = Format Date/Time String(seconds (now)=w1881) -> (date/time string=→"TimeNow":string)  [unwired: 2 out]
      }
      event "EXIT": Value Change {
        n1088 = event-data() -> ()  [unwired: 2 out]
        n1089 = property on="Property Node" class="Application"(error in=errorcluster {"status"=FALSE, "code"=0, "source"=""} ("error in (no error)")) -> (error out=w1883:errorcluster, "Application:Kind"=w1888:T37)  [unwired: 1 in, 1 out]
        n1090 = Two Button Dialog(message="Exit BIMS Collector?\nAll Unsaved data will be lost.", 1:"NO" ("F button name (\"Cancel\")"), 2:"YES" ("T button name (\"OK\")")) -> (T button?=w1889:bool)
        n1091 = case shown="\"Development System\"" w1888 {
          tunnel: w1889 -> [w1890 w1891 w1892]
          frame Default {
            n1092 = Stop(stop? (T)=w1890) -> ()
          }
          frame "Development System" {
            n1093 = Stop(stop? (T)=w1891) -> ()
          }
          frame "Run Time System" {
            n1094 = Quit LabVIEW(quit? (T)=w1892) -> ()
          }
        }
      }
      event "diagPageVisible": Value Change {
        # "Toggles display of \"Internal Use\" tab for diagnostics purposes"
        # "Key navigation ONLY: Cntrl-Shift-F11"
        n1095 = event-data() -> ("NewVal"=w1899:bool)  [unwired: 1 out]
        n1096 = property on="aboutTabCntrl" class="TabCtl (strict)"(error in=errorcluster {"status"=FALSE, "code"=0, "source"=""} ("error in (no error)")) -> (error out=w1898:errorcluster, "Pages"=w1902:refnum<vi>[])  [unwired: 1 in, 1 out]
        n1097 = Index Array(array=w1902, index=3) -> (element=w1900:refnum<vi>)
        n1098 = property on="Property Node" class="Page"(reference=w1900, error in=w1898, "PageVis"=w1899) -> (error out=w1897:errorcluster)  [unwired: 1 out]
        n1099 = property on="diagPageVisible" class="Bool (strict)"(error in=w1897, "Value"=w1899) -> (error out=w1894:errorcluster)  [unwired: 1 in, 1 out]
        n1100 = call <vilib>:"General Error Handler.vi"("error in (no error)"=w1894) -> ()  [unwired: 2 in, 13 out]
      }
      event "runtimeMenusVisible": Value Change {
        # "Key navigation ONLY: Cntrl-Shift-F10"
        n1101 = event-data() -> ("NewVal"=w1908:bool)  [unwired: 1 out]
        n1102 = control-ref of="This VI"() -> (w1907:refnum<vi>)
        n1103 = property class="VI"(reference=w1907, error in=w1906, "Front Panel.ShowMenuBar"=w1908) -> (reference out=w1905:refnum<vi>, error out=w1904:errorcluster)
        n1104 = Close Reference(reference=w1905, error in (no error)=w1904) -> (error out=w1903:errorcluster)
      }
      event "ARM": Value Change {
        # "This section will arm the system"
        n1105 = event-data() -> ()  [unwired: 2 out]
        n1106 = disable-structure shown="Disabled" {
          frame Disabled {
            "DIO" <- u32 21 ("DIO")
          }
          frame Enabled {
          }
        }
        n1107 = Bundle By Name(cluster=cluster{"ARMED":bool} {"ARMED"=FALSE} ("Safety_Interlock"), "ARMED"=TRUE) -> (→"SafetyInterlock":cluster{"ARMED":bool})
        n1108 = local write "SUBMIT DATE/TIME"("" ("Empty String Constant")) -> ()
        n1109 = local read "MeasSrc"() -> (w1916:T6)
        n1110 = case shown="\"Screens\"" w1916 {
          tunnel: w1915 -> [w1919 w1920 w1922]
          tunnel: [w1919 w1920 w1922] -> w1914
          frame "Simulated", Default {
          }
          frame "Radar" {
          }
          frame "Screens" {
            n1111 = local write "readyClock"(TRUE ("readyClock")) -> ()
          }
        }
      }
      event "QueryLoad": Value Change {
        w1930 = "%x" ("time format string (%c)")
        w1946 = "" ("replace string (\"\")")
        # "This section plots  Impact velocity vs. loadingdata"
        n1112 = event-data() -> ()  [unwired: 2 out]
        n1113 = Format Date/Time String(time format string (%c)=w1930, seconds (now)="lkupStartDate") -> (date/time string=w1929:string)  [unwired: 1 out]
        n1114 = Format Date/Time String(time format string (%c)=w1930, seconds (now)="lkupEndDate") -> (date/time string=w1928:string)  [unwired: 1 out]
        n1115 = call "Trim String.vi"("inStr"="Powder.freeTxt") -> ("outStr"=w1944:string)
        n1116 = call "Trim String.vi"("inStr"="Threat.freeTxt") -> ("outStr"=w1945:string)
        n1117 = invoke on="v50_table" class="Tbl" method="Reinit To Default"(error in=w1925) -> (error out=w1937:errorcluster)  [unwired: 2 in, 2 out]
        n1118 = invoke on="Vel.vs.Loading" class="WFGraph (strict)" method="Reinit To Default"(error in=w1937) -> (error out=w1932:errorcluster)  [unwired: 2 in, 2 out]
        n1119 = Format Into String(format string="SELECT TOP %d dbsrc.experiment.threat, dbsrc.shots.loading, dbsrc.shots.impact, dbsrc.experiment.powder, dbsrc.shots.date from dbsrc.shots, dbsrc.experiment where dbsrc.shots.expt = dbsrc.experiment.expt and dbsrc.shots.loading > 0 and dbsrc.shots.date between '%s' and '%s' and dbsrc.shots.impact between 10 and 5000 and dbsrc.experiment.powder like '%%%s%%' and dbsrc.experiment.threat like '%%%s%%' and experiment.threat<>'' order by dbsrc.experiment.threat, dbsrc.shots.loading, dbsrc.shots.impact;" ("Format String"), error in=w1932, "maxRecs", w1929, w1928, w1944, w1945) -> (resulting string=w1950:string, error out=w1935:errorcluster)  [unwired: 1 in]
        n1120 = Search and Replace String(input string=w1950, search string=" and experiment.powder like '%%'", replace string=w1946, error in=w1935) -> (result string=w1948:string, error out=w1936:errorcluster)  [unwired: 6 out]
        n1121 = Search and Replace String(input string=w1948, search string="and experiment.threat like '%%'", replace string=w1946, error in=w1936) -> (result string=w1939:string, error out=w1934:errorcluster)  [unwired: 6 out]
        n1122 = call "Fetch Data (SubVI).vi"("error IN"=w1934, "query string"=w1939) -> ("error OUT"=w1924:errorcluster, "recordset data"=w1940:string[][])  [unwired: 4 out]
        "v50_table" <- w1940
        n1123 = Fract/Exp String To Number(string=w1940) -> (number=w1954:dbl[][])  [unwired: 4 out]
        n1124 = Array Size(array=w1940) -> (size(s)=w1942:i32[])
        n1125 = Index Array(array=w1942) -> (element=→"ActualNumRecs":i32)  [unwired: 1 in]
        n1126 = Index Array(array=w1954, index (col)=2 ("Disabled Index (col)")) -> (element=w1953:dbl[])  [unwired: 1 in]
        n1127 = Index Array(array=w1954, index (col)=1 ("Disabled Index (col)")) -> (element=w1952:dbl[])  [unwired: 1 in]
        n1128 = Bundle(w1952, w1953) -> (→"Vel.vs.Loading":cluster{dbl[], dbl[]})  [unwired: 1 out]
      }
      event "ThreatGroups": Value Change {
        n1129 = event-data() -> ()  [unwired: 2 out]
        n1130 = control-ref of="ThreatGroups"() -> (w1963:refnum<vi>)
        n1131 = property on="Property Node" class="Ring (strict)"(reference=w1963, error in=w1962) -> (error out=w1960:errorcluster, "RingText.Text"=w1958:string)  [unwired: 1 out]
        n1132 = Not Equal?(x=w1958, y="") -> (x != y?=w1957:bool)
        n1133 = case shown="True" w1957 {
          tunnel: w1958 -> [_ w1973]
          tunnel: [w1965 w1971] -> w1961
          tunnel: w1960 -> [w1968 w1970]
          frame False {
            n1134 = property on="ThreatDetails" class="Ring (strict)"(error in=w1968, "Strings []"=string[] [], "Value"=u16 0 ("Value (Signaling)")) -> (error out=w1966:errorcluster)  [unwired: 1 in, 1 out]
            n1135 = invoke on="threatDetails" class="Clust (strict)" method="Reinit To Default"(error in=w1966) -> (error out=w1965:errorcluster)  [unwired: 2 in, 2 out]
          }
          frame True {
            n1136 = call "Select Threat Details.vi"("threatGroup"=w1973) -> ("threatDetails"=w1972:string[])  [unwired: 1 out]
            n1137 = property on="ThreatDetails" class="Ring (strict)"(error in=w1970, "Strings []"=w1972, "Val(Sgnl)"=u16 0 ("Value (Signaling)")) -> (error out=w1971:errorcluster)  [unwired: 1 in, 1 out]
          }
        }
      }
      event "panelSearch": Value Change {
        # "This section returns past panels"
        n1138 = event-data() -> ()  [unwired: 2 out]
        n1139 = control-ref of="pastPanels"() -> (w1983:refnum<vi>)
        n1140 = control-ref of="Mfr_0"() -> (w1977:refnum<vi>)
        n1141 = control-ref of="SampleStyle_0"() -> (w1978:refnum<vi>)
        n1142 = control-ref of="Requestors_0"() -> (w1976:refnum<vi>)
        n1143 = control-ref of="ThreatSize_0"() -> (w1975:refnum<vi>)
        n1144 = call "queryPanels (SubVI).vi"("ThreatSize_0"=w1975, "Mfr_0"=w1977, "Requestors_0"=w1976, "Style_0"=w1978, "error in"=w1981, "srchParams"="srchParams", "pastPanels"=w1983) -> ("error out"=w1980:errorcluster, "recordset data"=→"pastPanels":string[][], "actualNumPanels"=→"actualNumPanels":i32)  [unwired: 2 in]
      }
      event "pastPanels": Mouse Up {
        n1145 = event-data() -> ("CtlRef"=w1997:refnum<vi>)  [unwired: 1 out]
        n1146 = property on="Property Node" class="Tbl (strict)"(reference=w1997, error in=w1989) -> (error out=w1988:errorcluster, "Value"=w1996:string[][], "EditPos"=w1995:T38)  [unwired: 1 out]
        n1147 = Unbundle By Name(w1995) -> ("Row"=w1994:i32)
        n1148 = Index Array(array=w1996, index (row)=w1994, index (col)=0 ("disabled index (col)")) -> (element=w1993:string)
        n1149 = Scan From String(input string=w1993, error in=w1988, default 1=1 ("Record #")) -> (error out=w1987:errorcluster, output 1=w1991:i32)  [unwired: 2 in, 2 out]
        n1150 = local write "Record #"(w1991) -> ()
      }
      event "ThreatDetails", "SampleID": Value Change {
        # "A Sample ID is entered"
        # "A range is selected"
        # "A measurement requires the selection of a threat,\nso delay enabling the \"Measure\" tab until a grain wt\nis chosen."
        n1151 = event-data() -> ()  [unwired: 2 out]
        n1152 = control-ref of="ThreatGroups"() -> (w2016:refnum<vi>)
        n1153 = control-ref of="ThreatDetails"() -> (w2013:refnum<vi>)
        n1154 = call "Get Projectile Atributes from ThreatGroupDetail.vi"("error IN"=w2015, "ThreatDetail"=w2013, "ThreatGroup"=w2016) -> ("error out"=w2014:errorcluster, "projectileAttribs"=w2012:T39)  [unwired: 1 out]
        "threatDetails" <- w2012
        n1155 = Unbundle By Name(w2012) -> ("grainSize"=w2005:string)
        n1156 = Equal?(x=w2005, y="") -> (x = y?=w2006:bool)
        n1157 = case shown="False" w2006 {
          tunnel: w2005 -> [w2034 _]
          tunnel: [w2033 u16 0 ("GrainSize")] -> w2011
          frame False {
            # "A grain size is selected"
            n1158 = Scan From String(input string=w2034) -> (output 1=w2033:u16)  [unwired: 3 in, 4 out]
            "GrainSize" <- w2033
          }
          frame True {
            # "A grain size not selected"
          }
        }
        n1159 = Equal?(x=w2005, y="") -> (x = y?=w2031:bool)
        n1160 = local read "rangeSetup"() -> (w2028:u16)
        n1161 = case shown="False" w2031 {
          tunnel: [w2038 sgl 0.0] -> w2027
          tunnel: w2005 -> [w2036 _]
          frame False {
            w2040 = sgl 0.0  # sgl
            n1162 = Scan From String(format string="%f " ("Format String"), input string=w2036, default 1=w2040) -> (output 1=w2039:sgl)  [unwired: 2 in, 3 out]
            n1163 = disable-structure shown="Enabled" {
              disable-tunnel: w2039 -> [w2043 w2044]
              disable-tunnel: [w2042 w2044] -> w2038
              frame Disabled {
                n1164 = Multiply(x=sgl 0.06479891, y=w2043) -> (x*y=w2042:sgl)
              }
              frame Enabled {
              }
            }
          }
          frame True {
          }
        }
        "Projectile Mass" <- w2027
        n1165 = local read "SampleID"() -> (w2010:string)
        n1166 = Greater Than 0?(x=w2028) -> (x > 0?=w2029:bool)
        n1167 = Greater Than 0?(x=w2011) -> (x > 0?=w2030:bool)
        n1168 = Not Equal?(x=w2010, y="") -> (x != y?=w2008:bool)
        n1169 = Compound Arithmetic op=AND(w2030, w2029, w2008) -> (w2003:bool)
        n1170 = property on="mainTabCntrl" class="TabCtl (strict)"(error in=w2014) -> (error out=w2020:errorcluster, "Pages"=w2023:refnum<vi>[])  [unwired: 1 in, 1 out]
        n1171 = Not(x=w2003) -> (.not. x?=w2019:bool)
        n1172 = Index Array(array=w2023, index=1) -> (element=w2021:refnum<vi>)
        n1173 = Select(t=T15."Page Enabled" ("Page Enabled State"), s=w2003, f=T15."Page Disabled & Grayed" ("Page Enabled State")) -> (s? t:f=w2002:T15)
        n1174 = property on="Property Node" class="Page"(reference=w2021, error in=w2020, "PageEnb"=w2002) -> (error out=w2018:errorcluster)  [unwired: 1 out]
        n1175 = Select(t=T14."Enabled" ("Disabled"), s=w2003, f=T14."Disabled and Grayed Out" ("Disabled")) -> (s? t:f=w2000:T14)
        n1176 = property on="ARM" class="Bool"(error in=w2018, "Disabled"=w2000) -> (error out=w2026:errorcluster)  [unwired: 1 in, 1 out]
        n1177 = property on="addShot" class="Bool"(error in=w2026, "Disabled"=w2000) -> (error out=w2025:errorcluster)  [unwired: 1 in, 1 out]
        n1178 = property on="instruct_addShot" class="Str"(error in=w2025, "Visible"=w2019) -> (error out=w2024:errorcluster)  [unwired: 1 in, 1 out]
      }
      event "Mfr_1", "Mfr_2", "Mfr_3", "Mfr_4", "Mfr_5", "Mfr_6", "Mfr_0": Value Change {
        n1179 = event-data() -> ("CtlRef"=w2062:refnum<vi>)  [unwired: 1 out]
        n1180 = property on="Property Node" class="Ring (strict)"(reference=w2062, error in=w2054) -> (error out=w2052:errorcluster, "Label.Text"=w2058:string, "RingText.Text"=w2059:string)  [unwired: 1 out]
        n1181 = flat-sequence {
          tunnel: ["Mfr_1"] -> _
          tunnel: ["Mfr_2"] -> _
          tunnel: ["Mfr_3"] -> _
          tunnel: ["Mfr_4"] -> _
          tunnel: ["Mfr_5"] -> _
          tunnel: ["Mfr_6"] -> _
          frame #0 {
          }
        }
        n1182 = call "Select Sample Style.vi"("error IN"=w2052, "Mfr"=w2059) -> ("error Out"=w2051:errorcluster, "SampleStyles"=w2047:string[])  [unwired: 4 out]
        n1183 = Scan From String(format string="Mfr_%d", input string=w2058, error in=w2051, default 1=0 ("Mfr#")) -> (error out=w2048:errorcluster, output 1=w2057:i32)  [unwired: 1 in, 2 out]
        n1184 = case shown="1" w2057 {
          tunnel: [w2074 w2077 w2080 w2083 w2086 w2089 w2092] -> w2056
          tunnel: [w2073 w2076 w2079 w2082 w2085 w2088 w2091] -> w2049
          tunnel: w2048 -> [w2073 w2076 w2079 w2082 w2085 w2088 w2091]
          tunnel: w2047 -> [w2072 w2075 w2078 w2081 w2084 w2087 w2090]
          tunnel: [w2071 w2075 w2078 w2081 w2084 w2087 w2090] -> w2046
          frame 0, Default {
            n1185 = Delete From Array(array=w2072, length=1, index=0) -> (array with subset deleted=w2071:string[])  [unwired: 1 out]
            n1186 = control-ref of="SampleStyle_0"() -> (w2074:refnum<vi>)
          }
          frame 1 {
            n1187 = control-ref of="SampleStyle_1"() -> (w2077:refnum<vi>)
          }
          frame 2 {
            n1188 = control-ref of="SampleStyle_2"() -> (w2080:refnum<vi>)
          }
          frame 3 {
            n1189 = control-ref of="SampleStyle_3"() -> (w2083:refnum<vi>)
          }
          frame 4 {
            n1190 = control-ref of="SampleStyle_4"() -> (w2086:refnum<vi>)
          }
          frame 5 {
            n1191 = control-ref of="SampleStyle_5"() -> (w2089:refnum<vi>)
          }
          frame 6 {
            n1192 = control-ref of="SampleStyle_6"() -> (w2092:refnum<vi>)
          }
        }
        n1193 = property on="Property Node" class="Ring (strict)"(reference=w2056, error in=w2049, "Strings []"=w2046, "Val(Sgnl)"=u16 0 ("Value (Signaling)")) -> (error out=w2053:errorcluster)  [unwired: 1 out]
      }
      event "SampleStyle_1", "SampleStyle_2", "SampleStyle_3", "SampleStyle_4", "SampleStyle_5", "SampleStyle_6", "SampleStyle_0": Value Change {
        n1194 = event-data() -> ("CtlRef"=w2103:refnum<vi>)  [unwired: 1 out]
        n1195 = call "Get Sample Style Atributes.vi"("StyleNumRef"=w2103) -> ("SampleSpecs"=w2098:T40)  [unwired: 1 in]
        n1196 = flat-sequence {
          tunnel: ["SampleStyle_1"] -> _
          tunnel: ["SampleStyle_2"] -> _
          tunnel: ["SampleStyle_3"] -> _
          tunnel: ["SampleStyle_4"] -> _
          tunnel: ["SampleStyle_5"] -> _
          tunnel: ["SampleStyle_6"] -> _
          frame #0 {
          }
        }
        n1197 = property on="Property Node" class="Ring (strict)"(reference=w2103, error in=w2097) -> (error out=w2096:errorcluster, "Label.Text"=w2102:string)  [unwired: 1 out]
        n1198 = Scan From String(format string="SampleStyle_%d", input string=w2102, error in=w2096, default 1=0 ("default value 1")) -> (error out=w2095:errorcluster, output 1=w2100:i32)  [unwired: 1 in, 2 out]
        n1199 = case shown="1" w2100 {
          tunnel: w2098 -> [w2112 w2115 w2118 w2121 w2124 w2127 w2130]
          tunnel: w2095 -> [w2111 w2114 w2117 w2120 w2123 w2126 w2129]
          tunnel: [w2110 w2113 w2116 w2119 w2122 w2125 w2128] -> w2094
          frame 0, Default {
            n1200 = property on="SampleAttribs_0" class="Clust (strict)"(error in=w2111, "Val(Sgnl)"=w2112) -> (error out=w2110:errorcluster)  [unwired: 1 in, 1 out]
            "SampleAttribs_0" <- w2112
          }
          frame 1 {
            n1201 = property on="SampleAttribs_1" class="Clust (strict)"(error in=w2114, "Val(Sgnl)"=w2115) -> (error out=w2113:errorcluster)  [unwired: 1 in, 1 out]
            "SampleAttribs_1" <- w2115
          }
          frame 2 {
            n1202 = property on="SampleAttribs_2" class="Clust (strict)"(error in=w2117, "Val(Sgnl)"=w2118) -> (error out=w2116:errorcluster)  [unwired: 1 in, 1 out]
            "SampleAttribs_2" <- w2118
          }
          frame 3 {
            n1203 = property on="SampleAttribs_3" class="Clust (strict)"(error in=w2120, "Val(Sgnl)"=w2121) -> (error out=w2119:errorcluster)  [unwired: 1 in, 1 out]
            "SampleAttribs_3" <- w2121
          }
          frame 4 {
            n1204 = property on="SampleAttribs_4" class="Clust (strict)"(error in=w2123, "Val(Sgnl)"=w2124) -> (error out=w2122:errorcluster)  [unwired: 1 in, 1 out]
            "SampleAttribs_4" <- w2124
          }
          frame 5 {
            n1205 = property on="SampleAttribs_5" class="Clust (strict)"(error in=w2126, "Val(Sgnl)"=w2127) -> (error out=w2125:errorcluster)  [unwired: 1 in, 1 out]
            "SampleAttribs_5" <- w2127
          }
          frame 6 {
            n1206 = property on="SampleAttribs_6" class="Clust (strict)"(error in=w2129, "Val(Sgnl)"=w2130) -> (error out=w2128:errorcluster)  [unwired: 1 in, 1 out]
            "SampleAttribs_6" <- w2130
          }
        }
      }
      event "SHOTS", "Sort by AVG": Value Change {
        n1207 = event-data() -> ()  [unwired: 2 out]
        n1208 = local read "Site"() -> (w2131:string)
        n1209 = local read "SHOTS"() -> (w2135:T7[])
        n1210 = call "Update Shot Table.vi"("Sort by AVG"="Sort by AVG", "Site"=w2131, "shotsArr"=w2135) -> ("shotTable OUT"=→"Table of Shots":string[][])
      }
      event "Layer_1.plyNum", "Layer_2.plyNum", "Layer_3.plyNum", "Layer_4.plyNum", "Layer_5.plyNum", "Layer_6.plyNum", "SampleAttribs_1.ozPerYd2", "SampleAttribs_2.ozPerYd2", "SampleAttribs_3.ozPerYd2", "SampleAttribs_4.ozPerYd2", "SampleAttribs_5.ozPerYd2", "SampleAttribs_6.ozPerYd2": Value Change {
        n1211 = event-data() -> ()  [unwired: 2 out]
        n1212 = global read "BIMS_Collector Globals.vi" "SampleAttribs"() -> (w2146:T23)
        n1213 = Build Array("Layer_1", "Layer_2", "Layer_3", "Layer_4", "Layer_5", "Layer_6") -> (w2139:T41)
        n1214 = global write "BIMS_Collector Globals.vi" "LayerSpecs"(w2139) -> ()
        n1215 = for {
          tunnel: w2139 -> [w2167] mode=indexing
          shift-right: [w2169] -> w2148
          shift-left: 0 -> [w2168]
          tunnel: [w2166] -> w2158 mode=indexing
          tunnel: w2146 -> [w2164] mode=indexing
          n1216 = Unbundle By Name(w2164) -> ("ozPerYd2"=w2160:string)
          n1217 = Equal?(x=w2160, y="" ("Empty String Constant")) -> (x = y?=w2159:bool)
          n1218 = case shown="False" w2159 {
            tunnel: [w2173 sgl 0.0 ("default value 1")] -> w2163
            tunnel: w2160 -> [w2170 _]
            frame False {
              n1219 = Scan From String(format string="%f", input string=w2170, default 1=sgl 0.0 ("default value 1")) -> (output 1=w2173:sgl)  [unwired: 2 in, 3 out]
            }
            frame True {
            }
          }
          n1220 = Unbundle By Name(w2167) -> ("plyNum"=w2165:i32)
          n1221 = Add(x=w2168, y=w2165) -> (x+y=w2169:i32)
          n1222 = To Single Precision Float(number=w2165) -> (single precision float=w2162:sgl)
          n1223 = Multiply(x=w2162, y=w2163) -> (x*y=w2166:sgl)
        }
        "totalNumLayers" <- w2148
        n1224 = Divide(x=w2158, y=sgl 144.0) -> (x/y=w2156:sgl[])
        n1225 = Index Array(array=w2156) -> (element #1=→"fab1_totalWt":sgl, element #2=→"fab2_totalWt":sgl, element #3=→"fab3_totalWt":sgl, element #4=→"fab4_totalWt":sgl, element #5=→"fab5_totalWt":sgl, element #6=→"fab6_totalWt":sgl)  [unwired: 6 in]
        n1226 = Add Array Elements(numeric array=w2156) -> (sum=→"totalBAW":sgl)
      }
      event "clayCalArray": Value Change {
        n1227 = event-data() -> ()  [unwired: 2 out]
        n1228 = for {
          tunnel: "clayCalArray" -> [w2202] mode=indexing
          shift-right: [w2201] -> w2184
          shift-left: "" ("Empty String Constant") -> [w2199]
          shift-right: [w2196] -> w2180
          shift-left: i16[] [] -> [w2195]
          n1229 = Greater Than 0?(x=w2202) -> (x > 0?=w2203:bool)
          n1230 = case shown="False" w2203 {
            tunnel: w2202 -> [_ w2209]
            tunnel: ["##" ("clayCalib") w2211] -> w2200
            tunnel: w2199 -> [w2206 w2210]
            tunnel: [w2206 w2210] -> w2198
            tunnel: [w2204 w2208] -> w2196
            tunnel: w2195 -> [w2204 w2207]
            frame False {
            }
            frame True {
              n1231 = Format Into String(w2209) -> (resulting string=w2211:string)  [unwired: 3 in, 1 out]
              n1232 = Build Array (concatenate)(w2207, w2209) -> (w2208:i16[])
            }
          }
          n1233 = Concatenate Strings(w2198, w2200, "-" ("string")) -> (w2201:string)
        }
        n1234 = String Length(string=w2184) -> (length=w2185:i32)
        n1235 = Add Array Elements(numeric array=w2180) -> (sum=w2189:i16)
        n1236 = Array Size(array=w2180) -> (size(s)=w2190:i32)
        n1237 = Decrement(x=w2185) -> (x-1=w2182:i32)
        n1238 = To Single Precision Float(number=w2189) -> (single precision float=w2188:sgl)
        n1239 = To Single Precision Float(number=w2190) -> (single precision float=w2178:sgl)
        n1240 = String Subset(string=w2184, length (rest)=w2182) -> (substring=w2183:string)  [unwired: 1 out]
        n1241 = Equal To 0?(x=w2178) -> (x = 0?=w2177:bool)
        n1242 = local write "clayCalib"(w2183) -> ()
        n1243 = case shown="True" w2177 {
          tunnel: w2188 -> [w2193 w2194]
          tunnel: w2178 -> [w2192 _]
          tunnel: [w2191 w2194] -> w2187
          frame False {
            n1244 = Divide(x=w2193, y=w2192) -> (x/y=w2191:sgl)
          }
          frame True {
          }
        }
        "clayAverage" <- w2187
      }
      event "reportV50_History": Value Change {
        n1245 = event-data() -> ()  [unwired: 2 out]
        n1246 = local write "lookupRec"(TRUE ("lookupRec")) -> ()
      }
      event "Methods": Value Change {
        n1247 = event-data() -> ("CtlRef"=w2221:refnum<vi>)  [unwired: 1 out]
        n1248 = call "Dropdown Selection (SubVI).vi"("reference"=w2221) -> ("element"=w2220:string)
        n1249 = Equal?(x=w2220, y="V50") -> (x = y?=w2218:bool)
        n1250 = property on="minV50" class="DigNum (strict)"(error in=w2217, "Visible"=w2218) -> (error out=w2216:errorcluster)  [unwired: 1 in, 1 out]
      }
      event "rangeSetup": Value Change {
        n1251 = event-data() -> ("NewVal"=w2231:u16)  [unwired: 1 out]
        n1252 = case shown="2" w2231 {
          tunnel: ["0" ("section") "5.0" ("section") "7.5" ("section") "45.0" ("section")] -> w2237
          frame 0, Default {
          }
          frame 1 {
          }
          frame 2 {
          }
          frame 3 {
          }
        }
        n1253 = local read "configPath"() -> (w2239:path)
        n1254 = local read "GrainSize"() -> (w2230:u16)
        n1255 = Greater Than 0?(x=w2231) -> (x > 0?=w2234:bool)
        n1256 = Greater Than 0?(x=w2230) -> (x > 0?=w2232:bool)
        n1257 = call <vilib>:"Open Config Data (compatibility).vi"("error in (no error)"=w2227, "configuration file path"=w2239) -> ("error out"=w2247:errorcluster, "refnum"=w2249:T35)  [unwired: 7 in, 1 out]
        n1258 = And(x=w2234, y=w2232) -> (x .and. y?=w2233:bool)
        n1259 = call-poly <vilib>:"Write Key.vi"("write raw string? (F)"=TRUE, "section"="Ballistic Parameters", "error in (no error)"=w2247, "value"=w2237, "key"="MidPoint To Target Distance", "refnum"=w2249) -> ("error out"=w2246:errorcluster, "refnum out"=w2245:T35)  [unwired: 4 out]
        n1260 = call <vilib>:"Close Config Data.vi"("error in (no error)"=w2246, "refnum"=w2245) -> ("error out"=w2238:errorcluster)  [unwired: 1 in, 8 out]
        n1261 = Not(x=w2233) -> (.not. x?=w2243:bool)
        n1262 = Select(t=u8 0 ("y"), s=w2233, f=u8 2 ("y")) -> (s? t:f=w2229:u8)
        n1263 = Scan From String(input string=w2237, error in=w2238, default 1=sgl 0.0 ("default value 1")) -> (error out=w2226:errorcluster, output 1=w2236:sgl)  [unwired: 2 in, 2 out]
        n1264 = local write "mid_to_targ_dist"(w2236) -> ()
        n1265 = property on="ARM" class="Bool"(error in=w2226, "Disabled"=w2229) -> (error out=w2225:errorcluster)  [unwired: 1 in, 1 out]
        n1266 = property on="addShot" class="Bool"(error in=w2225, "Disabled"=w2229) -> (error out=w2224:errorcluster)  [unwired: 1 in, 1 out]
        n1267 = property on="instruct_addShot" class="Str"(error in=w2224, "Visible"=w2243) -> (error out=w2223:errorcluster)  [unwired: 1 in, 1 out]
        "instruct_addShot" <- "RANGE SETUP and THREAT must be selected before shots can be added." ("instruct_addShot")
      }
      event "Drag Corrected", "maxDev": Value Change {
        n1268 = event-data() -> ()  [unwired: 2 out]
        n1269 = local write "processShots"(TRUE ("ProcessShots")) -> ()
      }
      event "MC Listbox of Shots": Mouse Up {
        n1270 = event-data() -> ()  [unwired: 2 out]
        n1271 = flat-sequence {
          tunnel: w2262 -> [w2266]
          tunnel: [w2264] -> w2261
          tunnel: ["MC Listbox of Shots"] -> w2258
          tunnel: w2261 -> [w2270]
          tunnel: [w2269] -> w2260
          tunnel: w2258 -> [_]
          tunnel: w2260 -> [w2275]
          tunnel: [w2273] -> w2259
          frame #0 {
            n1272 = property on="Table of Shots" class="Tbl (strict)"(error in=w2266) -> (error out=w2265:errorcluster, "Value"=w2267:string[][])  [unwired: 1 in, 1 out]
            n1273 = local write "STOP (Shots MC LB)"(FALSE ("STOP (Shots MC LB)")) -> ()
            n1274 = property on="MC Listbox of Shots" class="MCListbox (strict)"(error in=w2265, "ItemNames"=w2267) -> (error out=w2264:errorcluster)  [unwired: 1 in, 1 out]
          }
          frame #1 {
            n1275 = control-ref of="MC Listbox of Shots"() -> (w2272:refnum<vi>)
            n1276 = control-ref of="STOP (Shots MC LB)"() -> (w2271:refnum<vi>)
            n1277 = call "multicolumn listbox sort.vi"("error IN"=w2270, "Bool Refnum"=w2271, "MCListbox Refnum"=w2272) -> ("error out"=w2269:errorcluster)  [unwired: 4 in]
          }
          frame #2 {
            n1278 = property on="MC Listbox of Shots" class="MCListbox (strict)"(error in=w2275) -> (error out=w2274:errorcluster, "ItemNames"=w2276:string[][])  [unwired: 1 in, 1 out]
            n1279 = property on="Table of Shots" class="Tbl (strict)"(error in=w2274, "Val(Sgnl)"=w2276) -> (error out=w2273:errorcluster)  [unwired: 1 in, 1 out]
          }
        }
      }
      event "PublishNewRecords": Value Change {
        w2282 = "\\" ("string")
        w2293 = TRUE  # overwrite (F)
        # "2. INSERT new records to Experiments and  \n      Shots tables in local Export.mdb file."
        # "1. SELECT new records from local MDB \n     by comparing against last record numbers \n     found in IMPORT table on BIMS server."
        # "Pushes latest ballistics performance data up to BIMS Server\n\n - Attempts connection with server (reports connection success in msgbox)\n - If successful:\n   - Exports all experiment/shot records since last table marker to [site].mdb file\n   - Sends export.mdb file to drop location on BIMS File Server\n   - Executes SSIS package to import records from export.mdb file\n - Otherwise provides option to try again or cancel"
        # "3. Copy Export.mdb file to [sitename].mdb in [sitename] \n      FileDrop folder on BIMS server."
        n1280 = event-data() -> ()  [unwired: 2 out]
        n1281 = property on="Loading" class="Ring (strict)"(error in=w2288, "Visible"=TRUE) -> (error out=w2287:errorcluster)  [unwired: 1 in, 1 out]
        n1282 = local read "Site"() -> (w2277:string)
        n1283 = call "Export New Records.vi"("error IN"=w2287, "Site"=w2277) -> ("error out"=w2295:errorcluster)  [unwired: 3 in, 6 out]
        n1284 = Concatenate Strings("\\\\" ("string"), "Server", w2282, "Folder", w2282, w2277, ".mdb" ("string")) -> (w2278:string)
        n1285 = String To Path(string=w2278) -> (path=w2291:path)
        n1286 = Copy(8:w2295, 9:w2293, 10:w2291, 11:path "C:/Ballistics/Export.mdb" ("source path")) -> (0:w2292:errorcluster)  [unwired: 3 out]
        n1287 = case shown="No Error" w2292 {
          selector: w2292 -> [w2297 w2299]
          tunnel: [w2297 w2298] -> w2286
          frame No Error {
            n1288 = One Button Dialog(message="New sample performance records submitted \nto BIMS Warehouse successfully.\n\nPublishing will occur in under five minutes.") -> ()  [unwired: 2 out]
          }
          frame Error {
            n1289 = call <vilib>:"General Error Handler.vi"("error in (no error)"=w2299) -> ("error out"=w2298:errorcluster)  [unwired: 2 in, 12 out]
          }
        }
        n1290 = property on="Loading" class="Ring (strict)"(error in=w2286, "Visible"=FALSE) -> (error out=w2285:errorcluster)  [unwired: 1 in, 1 out]
      }
      event "arrIDC": Mouse Up {
        n1291 = event-data() -> ()  [unwired: 2 out]
        "velProfile" <- cluster{dbl, dbl}[] [] ("velProfile")
        "arrIDC" <- dbl[] [] ("arrIDC")
        "relativeTime" <- cluster{"ts2":dbl, "ts3":dbl, "ts1":dbl} {"ts2"=0.0, "ts3"=0.0, "ts1"=0.0} ("relativeTime")
        "velMeasProf" <- T8 {"v2"=0.0, "vB"=0.0, "vOuter"=0.0, "v1"=0.0, "vA"=0.0, "vInner"=0.0} ("velMeasProf")
        "velCompProf" <- cluster{"vStrike":dbl, "vA":dbl} {"vStrike"=0.0, "vA"=0.0} ("velCompProf")
        "displacement" <- T9 {"ds_v2"=6.75, "ds2"=5.0833, "ds_vB"=4.9167, "ds3"=4.75, "ds_vAvg"=6.9167, "ds_v1"=7.0833, "ds1"=8.75, "ds_vA"=8.9167, "ds0"=9.0833} ("displacement")
      }
      event "SampleBackings": Value Change {
        # "Clay is the default sample backing material.\n\n  If another selection is made, then grey out and disable all controls relating to clay."
        n1292 = event-data() -> ()  [unwired: 2 out]
        n1293 = case shown="0, Default" "SampleBackings" {
          tunnel: [T14."Disabled and Grayed Out" ("Disabled") T14."Enabled" ("Disabled") T14."Disabled and Grayed Out" ("Disabled")] -> w2308
          frame 0, Default {
          }
          frame 1 {
          }
          frame 2.. {
          }
        }
        n1294 = property on="clayCalArray" class="Arr (strict)"("DisabledEnum"=w2308) -> ()  [unwired: 2 in, 2 out]
        n1295 = property on="clayAverage" class="DigNum (strict)"("DisabledEnum"=w2308) -> ()  [unwired: 2 in, 2 out]
        n1296 = property on="clayTemp" class="DigNum (strict)"("DisabledEnum"=w2308) -> ()  [unwired: 2 in, 2 out]
      }
      event "RefreshMetadata": Value Change {
        # "Pulls latest metadata down from BIMS Database Server\n - Attempts connection with server \n        (reports failure if connection is unsuccessful)\n - If successful:\n   - Updates local database records from server\n   - Updates dropdown listboxes from local database"
        n1297 = event-data() -> ()  [unwired: 2 out]
        n1298 = property on="Loading" class="Ring (strict)"(error in=w2338, "Visible"=TRUE) -> (error out=w2337:errorcluster)  [unwired: 1 in, 1 out]
        n1299 = control-ref of="LayerStitchTypes"() -> (w2322:refnum<vi>)
        n1300 = control-ref of="BackLayer"() -> (w2333:refnum<vi>)
        n1301 = control-ref of="FrontLayer"() -> (w2334:refnum<vi>)
        n1302 = control-ref of="ThreatGroups"() -> (w2335:refnum<vi>)
        n1303 = control-ref of="SampleClamping"() -> (w2343:refnum<vi>)
        n1304 = control-ref of="SampleTypes"() -> (w2360:refnum<vi>)
        n1305 = control-ref of="SampleDimensions"() -> (w2359:refnum<vi>)
        n1306 = control-ref of="ModelMfrs"() -> (w2358:refnum<vi>)
        n1307 = control-ref of="Assemblers"() -> (w2357:refnum<vi>)
        n1308 = control-ref of="Submitters"() -> (w2356:refnum<vi>)
        n1309 = control-ref of="PowderTypes"() -> (w2355:refnum<vi>)
        n1310 = control-ref of="Methods"() -> (w2352:refnum<vi>)
        n1311 = control-ref of="TestConditions"() -> (w2351:refnum<vi>)
        n1312 = control-ref of="SampleBackings"() -> (w2350:refnum<vi>)
        n1313 = control-ref of="Ballisticians"() -> (w2349:refnum<vi>)
        n1314 = control-ref of="Shooters"() -> (w2348:refnum<vi>)
        n1315 = control-ref of="Recorders"() -> (w2347:refnum<vi>)
        n1316 = Build Array(w2322, w2333, w2334, w2335, w2343, w2360, w2359, w2358, w2357, w2356, w2355, w2352, w2351, w2350, w2349, w2348, w2347) -> (w2354:refnum<vi>[])
        n1317 = call "Update Metadata using listbox names.vi"("error in"=w2337, "Site"="Site", "RefNumArrIn"=w2354) -> ("error out"=w2361:errorcluster, "RefNumArrOut"=w2353:refnum<vi>[])  [unwired: 1 in, 6 out]
        n1318 = call "Fill Lists from DB (1st Pass).vi"("error in"=w2361, "RefNumArray"=w2353) -> ("error out"=w2323:errorcluster)  [unwired: 1 in, 4 out]
        n1319 = call "Fill Stitch Lists.vi"("error IN"=w2323) -> ("error OUT"=w2318:errorcluster)  [unwired: 6 in]
        n1320 = control-ref of="ThreatSize_0"() -> (w2316:refnum<vi>)
        n1321 = control-ref of="Requestors_0"() -> (w2321:refnum<vi>)
        n1322 = Build Array(w2316, w2321) -> (w2320:refnum<vi>[])
        n1323 = call "Fill Lists from DB (2nd Pass).vi"("errorIN"=w2318, "colNames"=string[] ["GrainSize", "requestor"] ("lkupTableNames"), "lkupTableNames"=string[] ["ThreatDetails", "Submitters"], "RefNumArray"=w2320) -> ("error OUT"=w2317:errorcluster)  [unwired: 3 in]
        n1324 = flat-sequence {
          frame #0 {
            n1325 = local write "RefreshMetadata"(FALSE ("UpdateMetadata")) -> ()
            n1326 = local write "TimeNow"("Connecting to BIMS Server . . ." ("TimeNow")) -> ()
          }
        }
        n1327 = call "Create local tables from Server DB.vi"("error in"=w2317, "Site"="Site", "tableNames"=string[] ["Threats", "ThreatDetails", "ThreatCalibers", "Mfrs", "SampleStyles", "SampleSpecs", "FiberTypes"]) -> ("error out"=w2345:errorcluster)  [unwired: 1 in, 7 out]
        n1328 = call "Fill Lists From DB (3rd Pass).vi"("error IN"=w2345) -> ("error OUT"=w2325:errorcluster)  [unwired: 3 in, 3 out]
        n1329 = control-ref of="ModelMfrs"() -> (w2332:refnum<vi>)
        n1330 = property class="Ring (strict)"(reference=w2332, error in=w2325) -> (reference out=w2331:refnum<vi>, error out=w2330:errorcluster, "Strings []"=w2329:string[])
        n1331 = Delete From Array(array=w2329, length=1, index=0) -> (array with subset deleted=w2328:string[])  [unwired: 1 out]
        n1332 = property class="Ring (strict)"(reference=w2331, error in=w2330, "Strings []"=w2328) -> (error out=w2324:errorcluster)  [unwired: 1 out]
        n1333 = case shown="No Error" w2324 {
          selector: w2324 -> [w2362 w2365]
          tunnel: [w2362 w2365] -> w2341
          frame No Error {
            n1334 = local write "TimeNow"("Collector Metadata is READY!" ("TimeNow")) -> ()
            n1335 = Wait (ms)(milliseconds to wait=u32 2000) -> ()  [unwired: 1 out]
          }
          frame Error {
            n1336 = call <vilib>:"General Error Handler.vi"("error in (no error)"=w2365) -> ()  [unwired: 2 in, 13 out]
          }
        }
        n1337 = property on="Loading" class="Ring (strict)"(error in=w2341, "Visible"=FALSE) -> (error out=w2340:errorcluster)  [unwired: 1 in, 1 out]
      }
      event "loadingUnits": Value Change {
        n1338 = local read "Powder Loading"() -> (w2369:sgl)
        n1339 = event-data() -> ("NewVal"=w2368:enum32{"grams", "grains"})  [unwired: 6 out]
        n1340 = case shown="\"grams\", Default" w2368 {
          tunnel: w2369 -> [w2374 w2375]
          frame "grams", Default {
            n1341 = Multiply(x=w2374, y=sgl 0.06479891) -> (x*y=w2372:sgl)
            n1342 = local write "Powder Loading"(w2372) -> ()
          }
          frame "grains" {
            n1343 = Multiply(x=w2375, y=sgl 15.432359) -> (x*y=w2376:sgl)
            n1344 = local write "Powder Loading"(w2376) -> ()
          }
        }
      }
      event "clearErrors": Value Change {
        w2378 = errorcluster {"status"=FALSE, "code"=0, "source"=""} ("error in")
        n1345 = event-data() -> ()  [unwired: 7 out]
        n1346 = local write "SMErr"(w2378) -> ()
      }
    }
    "U/I EvErr" <- w1874
    "booleanDump" <- w1873
  }
